vi "ex_allChanPropsMod.vi"(4 "error in (no error)":errorcluster, 5 "propertySource":string, 6 "DAQmx Channel":refnum<k21>, 7 "DAQmx Task":refnum<k21>) -> (0 "error out":errorcluster, 1 "TDM Property":T1, 2 "dup DAQmx Channel":refnum<k21>)   [LabVIEW 2020]
uses:
  <vilib>/express/express shared/ExFile.llb/ex_TdmProperty.ctl
  <vilib>/express/express shared/ex_EditUserDefinedProperties/usiDataType.ctl
  <vilib>/Platform/express/ex_EditUserDefinedProperties/ex_setTdmProperty_BLN.vi
  <vilib>/Platform/express/ex_EditUserDefinedProperties/ex_setTdmProperty_DBL.vi
  <vilib>/Platform/express/ex_EditUserDefinedProperties/ex_setTdmProperty_STR.vi
  <vilib>/Platform/express/ex_EditUserDefinedProperties/ex_setTdmProperty_I32.vi
  <vilib>/Platform/express/ex_EditUserDefinedProperties/ex_setTdmProperty_TME.vi
  <vilib>/Platform/express/ex_EditUserDefinedProperties/ex_setTdmProperty_1dDBL.vi
  <resource>/objmgr/daqmx.rc
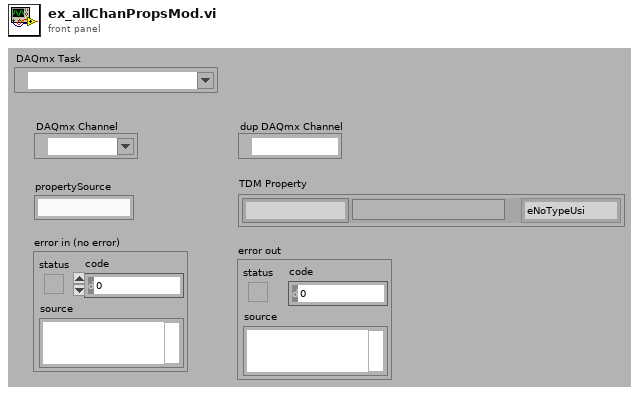
[diagram p1: front panel]
types:
  T1 = typedef "ex_TdmProperty.ctl" = cluster{"Name":string, "Type":T2, "Value":variant}
  T2 = typedef "usiDataType.ctl" = enum16{"eNoTypeUsi", "eInt8Usi", "eInt16Usi", "eInt32Usi", "eInt64Usi", "eUInt8Usi", "eUInt16Usi", "eUInt32Usi", "eUInt64Usi", "eFloat32Usi", "eFloat64Usi", "- 0", "- 1", "- 2", "- 3", "- 4", "- 5", "- 6", "- 7", "- 8", "- 9", "eString8Usi", "eString16Usi", "eStringUsi", "eEnumUsi", "- 10", "- 11", "- 12", "- 13", "- 14", "eTimeUsi", "- 15", "- 16", "- 17", "- 18", "- 19", "- 20", "- 21", "- 22", "- 23", "eInstanceUsi", "eStoreUsi"}
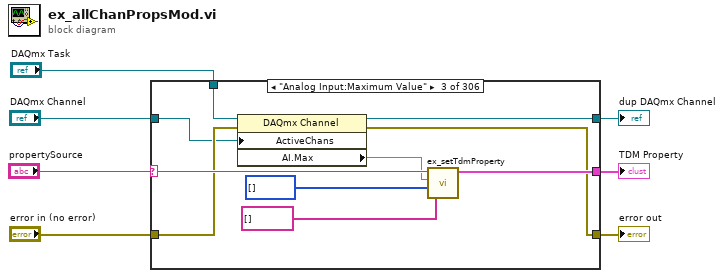
[diagram p0: block diagram]
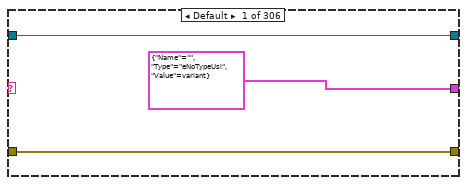
[diagram p2: hidden frame]
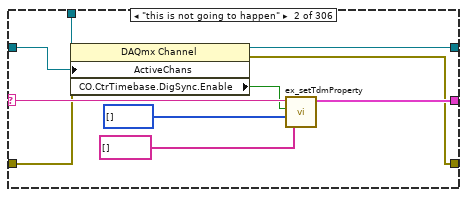
[diagram p3: hidden frame]
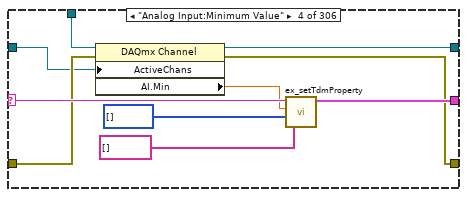
[diagram p4: hidden frame]
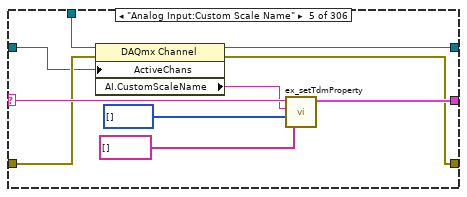
[diagram p5: hidden frame]
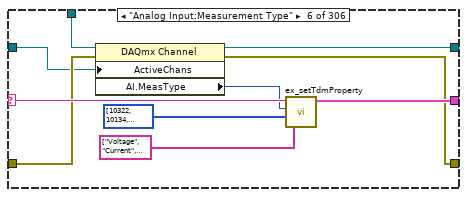
[diagram p6: hidden frame]
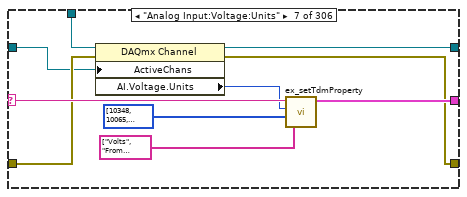
[diagram p7: hidden frame]
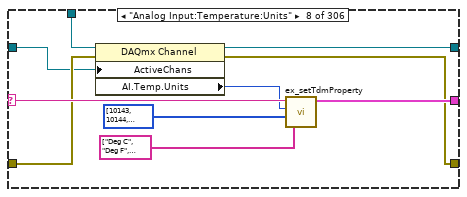
[diagram p8: hidden frame]
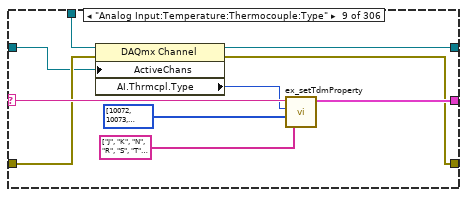
[diagram p9: hidden frame]
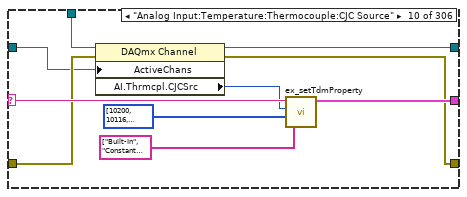
[diagram p10: hidden frame]
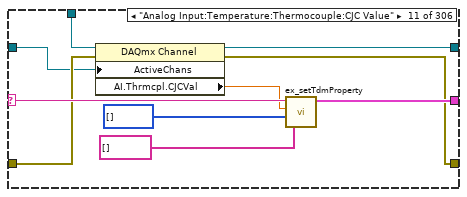
[diagram p11: hidden frame]
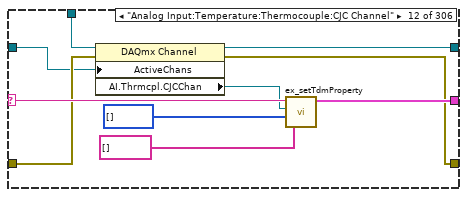
[diagram p12: hidden frame]
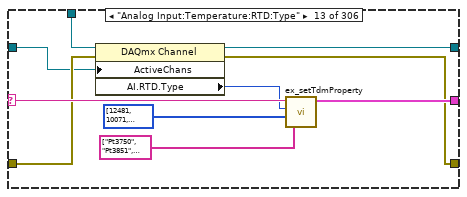
[diagram p13: hidden frame]
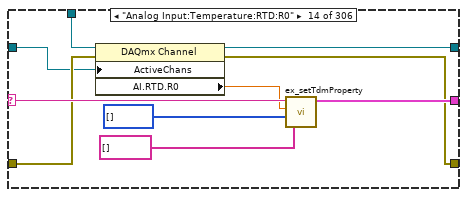
[diagram p14: hidden frame]
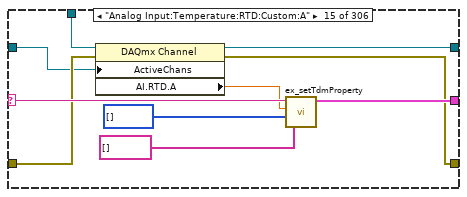
[diagram p15: hidden frame]
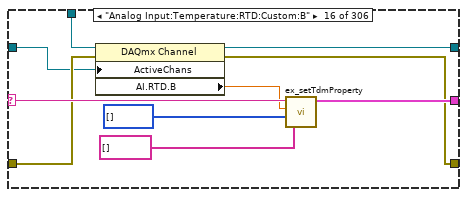
[diagram p16: hidden frame]
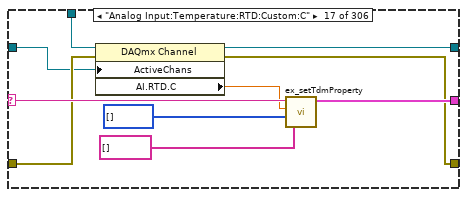
[diagram p17: hidden frame]
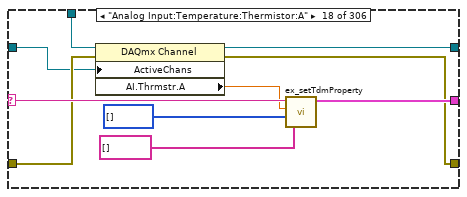
[diagram p18: hidden frame]
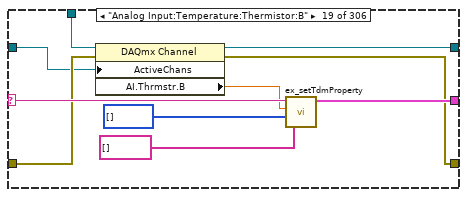
[diagram p19: hidden frame]
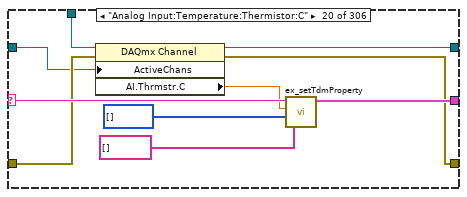
[diagram p20: hidden frame]
diagram:
  n1 = case shown="\"Analog Input:Maximum Value\"" "propertySource" {
    selector: "propertySource" -> [_ w19 w29 w39 w49 w59 w69 w79 w89 w99 w109 w119 w129 w139 w149 w159 w169 w179 w189 w199 w209 w219 w229 w239 w249 w259 w269 w279 w289 w299 w309 w319 w329 w339 w349 w359 w369 w379 w389 w399 w409 w419 w429 w439 w449 w459 w469 w479 w489 w499 w509 w519 w529 w539 w549 w559 w569 w579 w589 w599 w609 w619 w629 w639 w649 w659 w669 w679 w689 w699 w709 w719 w729 w739 w749 w759 w769 w779 w789 w799 w809 w819 w829 w839 w849 w859 w869 w879 w889 w899 w909 w919 w929 w939 w949 w959 w969 w979 w989 w999 w1009 w1019 w1029 w1039 w1049 w1059 w1069 w1079 w1089 w1099 w1109 w1119 w1129 w1139 w1149 w1159 w1169 w1179 w1189 w1199 w1209 w1219 w1229 w1239 w1249 w1259 w1269 w1279 w1289 w1299 w1309 w1319 w1329 w1339 w1349 w1359 w1369 w1379 w1389 w1399 w1409 w1419 w1429 w1439 w1449 w1459 w1469 w1479 w1489 w1499 w1509 w1519 w1529 w1539 w1549 w1559 w1569 w1579 w1589 w1599 w1609 w1619 w1629 w1639 w1649 w1659 w1669 w1679 w1689 w1699 w1709 w1719 w1729 w1739 w1749 w1759 w1769 w1779 w1789 w1799 w1809 w1819 w1829 w1839 w1849 w1859 w1869 w1879 w1889 w1899 w1909 w1919 w1929 w1939 w1949 w1959 w1969 w1979 w1989 w1999 w2009 w2019 w2029 w2039 w2049 w2059 w2069 w2079 w2089 w2099 w2109 w2119 w2129 w2139 w2149 w2159 w2169 w2179 w2189 w2199 w2209 w2219 w2229 w2239 w2249 w2259 w2269 w2279 w2289 w2299 w2309 w2319 w2329 w2339 w2349 w2359 w2369 w2379 w2389 w2399 w2409 w2419 w2429 w2439 w2449 w2459 w2469 w2479 w2489 w2499 w2509 w2519 w2529 w2539 w2549 w2559 w2569 w2579 w2589 w2599 w2609 w2619 w2629 w2639 w2649 w2659 w2669 w2679 w2689 w2699 w2709 w2719 w2729 w2739 w2749 w2759 w2769 w2779 w2789 w2799 w2809 w2819 w2829 w2839 w2849 w2859 w2869 w2879 w2889 w2899 w2909 w2919 w2929 w2939 w2949 w2959 w2969 w2979 w2989 w2999 w3009 w3019 w3029 w3039 w3049 w3059]
    tunnel: "error in (no error)" -> [w10 w17 w27 w37 w47 w57 w67 w77 w87 w97 w107 w117 w127 w137 w147 w157 w167 w177 w187 w197 w207 w217 w227 w237 w247 w257 w267 w277 w287 w297 w307 w317 w327 w337 w347 w357 w367 w377 w387 w397 w407 w417 w427 w437 w447 w457 w467 w477 w487 w497 w507 w517 w527 w537 w547 w557 w567 w577 w587 w597 w607 w617 w627 w637 w647 w657 w667 w677 w687 w697 w707 w717 w727 w737 w747 w757 w767 w777 w787 w797 w807 w817 w827 w837 w847 w857 w867 w877 w887 w897 w907 w917 w927 w937 w947 w957 w967 w977 w987 w997 w1007 w1017 w1027 w1037 w1047 w1057 w1067 w1077 w1087 w1097 w1107 w1117 w1127 w1137 w1147 w1157 w1167 w1177 w1187 w1197 w1207 w1217 w1227 w1237 w1247 w1257 w1267 w1277 w1287 w1297 w1307 w1317 w1327 w1337 w1347 w1357 w1367 w1377 w1387 w1397 w1407 w1417 w1427 w1437 w1447 w1457 w1467 w1477 w1487 w1497 w1507 w1517 w1527 w1537 w1547 w1557 w1567 w1577 w1587 w1597 w1607 w1617 w1627 w1637 w1647 w1657 w1667 w1677 w1687 w1697 w1707 w1717 w1727 w1737 w1747 w1757 w1767 w1777 w1787 w1797 w1807 w1817 w1827 w1837 w1847 w1857 w1867 w1877 w1887 w1897 w1907 w1917 w1927 w1937 w1947 w1957 w1967 w1977 w1987 w1997 w2007 w2017 w2027 w2037 w2047 w2057 w2067 w2077 w2087 w2097 w2107 w2117 w2127 w2137 w2147 w2157 w2167 w2177 w2187 w2197 w2207 w2217 w2227 w2237 w2247 w2257 w2267 w2277 w2287 w2297 w2307 w2317 w2327 w2337 w2347 w2357 w2367 w2377 w2387 w2397 w2407 w2417 w2427 w2437 w2447 w2457 w2467 w2477 w2487 w2497 w2507 w2517 w2527 w2537 w2547 w2557 w2567 w2577 w2587 w2597 w2607 w2617 w2627 w2637 w2647 w2657 w2667 w2677 w2687 w2697 w2707 w2717 w2727 w2737 w2747 w2757 w2767 w2777 w2787 w2797 w2807 w2817 w2827 w2837 w2847 w2857 w2867 w2877 w2887 w2897 w2907 w2917 w2927 w2937 w2947 w2957 w2967 w2977 w2987 w2997 w3007 w3017 w3027 w3037 w3047 w3057]
    tunnel: [w10 w16 w26 w36 w46 w56 w66 w76 w86 w96 w106 w116 w126 w136 w146 w156 w166 w176 w186 w196 w206 w216 w226 w236 w246 w256 w266 w276 w286 w296 w306 w316 w326 w336 w346 w356 w366 w376 w386 w396 w406 w416 w426 w436 w446 w456 w466 w476 w486 w496 w506 w516 w526 w536 w546 w556 w566 w576 w586 w596 w606 w616 w626 w636 w646 w656 w666 w676 w686 w696 w706 w716 w726 w736 w746 w756 w766 w776 w786 w796 w806 w816 w826 w836 w846 w856 w866 w876 w886 w896 w906 w916 w926 w936 w946 w956 w966 w976 w986 w996 w1006 w1016 w1026 w1036 w1046 w1056 w1066 w1076 w1086 w1096 w1106 w1116 w1126 w1136 w1146 w1156 w1166 w1176 w1186 w1196 w1206 w1216 w1226 w1236 w1246 w1256 w1266 w1276 w1286 w1296 w1306 w1316 w1326 w1336 w1346 w1356 w1366 w1376 w1386 w1396 w1406 w1416 w1426 w1436 w1446 w1456 w1466 w1476 w1486 w1496 w1506 w1516 w1526 w1536 w1546 w1556 w1566 w1576 w1586 w1596 w1606 w1616 w1626 w1636 w1646 w1656 w1666 w1676 w1686 w1696 w1706 w1716 w1726 w1736 w1746 w1756 w1766 w1776 w1786 w1796 w1806 w1816 w1826 w1836 w1846 w1856 w1866 w1876 w1886 w1896 w1906 w1916 w1926 w1936 w1946 w1956 w1966 w1976 w1986 w1996 w2006 w2016 w2026 w2036 w2046 w2056 w2066 w2076 w2086 w2096 w2106 w2116 w2126 w2136 w2146 w2156 w2166 w2176 w2186 w2196 w2206 w2216 w2226 w2236 w2246 w2256 w2266 w2276 w2286 w2296 w2306 w2316 w2326 w2336 w2346 w2356 w2366 w2376 w2386 w2396 w2406 w2416 w2426 w2436 w2446 w2456 w2466 w2476 w2486 w2496 w2506 w2516 w2526 w2536 w2546 w2556 w2566 w2576 w2586 w2596 w2606 w2616 w2626 w2636 w2646 w2656 w2666 w2676 w2686 w2696 w2706 w2716 w2726 w2736 w2746 w2756 w2766 w2776 w2786 w2796 w2806 w2816 w2826 w2836 w2846 w2856 w2866 w2876 w2886 w2896 w2906 w2916 w2926 w2936 w2946 w2956 w2966 w2976 w2986 w2996 w3006 w3016 w3026 w3036 w3046 w3056] -> w4
    tunnel: "DAQmx Channel" -> [w9 w12 w22 w32 w42 w52 w62 w72 w82 w92 w102 w112 w122 w132 w142 w152 w162 w172 w182 w192 w202 w212 w222 w232 w242 w252 w262 w272 w282 w292 w302 w312 w322 w332 w342 w352 w362 w372 w382 w392 w402 w412 w422 w432 w442 w452 w462 w472 w482 w492 w502 w512 w522 w532 w542 w552 w562 w572 w582 w592 w602 w612 w622 w632 w642 w652 w662 w672 w682 w692 w702 w712 w722 w732 w742 w752 w762 w772 w782 w792 w802 w812 w822 w832 w842 w852 w862 w872 w882 w892 w902 w912 w922 w932 w942 w952 w962 w972 w982 w992 w1002 w1012 w1022 w1032 w1042 w1052 w1062 w1072 w1082 w1092 w1102 w1112 w1122 w1132 w1142 w1152 w1162 w1172 w1182 w1192 w1202 w1212 w1222 w1232 w1242 w1252 w1262 w1272 w1282 w1292 w1302 w1312 w1322 w1332 w1342 w1352 w1362 w1372 w1382 w1392 w1402 w1412 w1422 w1432 w1442 w1452 w1462 w1472 w1482 w1492 w1502 w1512 w1522 w1532 w1542 w1552 w1562 w1572 w1582 w1592 w1602 w1612 w1622 w1632 w1642 w1652 w1662 w1672 w1682 w1692 w1702 w1712 w1722 w1732 w1742 w1752 w1762 w1772 w1782 w1792 w1802 w1812 w1822 w1832 w1842 w1852 w1862 w1872 w1882 w1892 w1902 w1912 w1922 w1932 w1942 w1952 w1962 w1972 w1982 w1992 w2002 w2012 w2022 w2032 w2042 w2052 w2062 w2072 w2082 w2092 w2102 w2112 w2122 w2132 w2142 w2152 w2162 w2172 w2182 w2192 w2202 w2212 w2222 w2232 w2242 w2252 w2262 w2272 w2282 w2292 w2302 w2312 w2322 w2332 w2342 w2352 w2362 w2372 w2382 w2392 w2402 w2412 w2422 w2432 w2442 w2452 w2462 w2472 w2482 w2492 w2502 w2512 w2522 w2532 w2542 w2552 w2562 w2572 w2582 w2592 w2602 w2612 w2622 w2632 w2642 w2652 w2662 w2672 w2682 w2692 w2702 w2712 w2722 w2732 w2742 w2752 w2762 w2772 w2782 w2792 w2802 w2812 w2822 w2832 w2842 w2852 w2862 w2872 w2882 w2892 w2902 w2912 w2922 w2932 w2942 w2952 w2962 w2972 w2982 w2992 w3002 w3012 w3022 w3032 w3042 w3052]
    tunnel: [w9 w20 w30 w40 w50 w60 w70 w80 w90 w100 w110 w120 w130 w140 w150 w160 w170 w180 w190 w200 w210 w220 w230 w240 w250 w260 w270 w280 w290 w300 w310 w320 w330 w340 w350 w360 w370 w380 w390 w400 w410 w420 w430 w440 w450 w460 w470 w480 w490 w500 w510 w520 w530 w540 w550 w560 w570 w580 w590 w600 w610 w620 w630 w640 w650 w660 w670 w680 w690 w700 w710 w720 w730 w740 w750 w760 w770 w780 w790 w800 w810 w820 w830 w840 w850 w860 w870 w880 w890 w900 w910 w920 w930 w940 w950 w960 w970 w980 w990 w1000 w1010 w1020 w1030 w1040 w1050 w1060 w1070 w1080 w1090 w1100 w1110 w1120 w1130 w1140 w1150 w1160 w1170 w1180 w1190 w1200 w1210 w1220 w1230 w1240 w1250 w1260 w1270 w1280 w1290 w1300 w1310 w1320 w1330 w1340 w1350 w1360 w1370 w1380 w1390 w1400 w1410 w1420 w1430 w1440 w1450 w1460 w1470 w1480 w1490 w1500 w1510 w1520 w1530 w1540 w1550 w1560 w1570 w1580 w1590 w1600 w1610 w1620 w1630 w1640 w1650 w1660 w1670 w1680 w1690 w1700 w1710 w1720 w1730 w1740 w1750 w1760 w1770 w1780 w1790 w1800 w1810 w1820 w1830 w1840 w1850 w1860 w1870 w1880 w1890 w1900 w1910 w1920 w1930 w1940 w1950 w1960 w1970 w1980 w1990 w2000 w2010 w2020 w2030 w2040 w2050 w2060 w2070 w2080 w2090 w2100 w2110 w2120 w2130 w2140 w2150 w2160 w2170 w2180 w2190 w2200 w2210 w2220 w2230 w2240 w2250 w2260 w2270 w2280 w2290 w2300 w2310 w2320 w2330 w2340 w2350 w2360 w2370 w2380 w2390 w2400 w2410 w2420 w2430 w2440 w2450 w2460 w2470 w2480 w2490 w2500 w2510 w2520 w2530 w2540 w2550 w2560 w2570 w2580 w2590 w2600 w2610 w2620 w2630 w2640 w2650 w2660 w2670 w2680 w2690 w2700 w2710 w2720 w2730 w2740 w2750 w2760 w2770 w2780 w2790 w2800 w2810 w2820 w2830 w2840 w2850 w2860 w2870 w2880 w2890 w2900 w2910 w2920 w2930 w2940 w2950 w2960 w2970 w2980 w2990 w3000 w3010 w3020 w3030 w3040 w3050 w3060] -> w6
    tunnel: [T1 {"Name"="", "Type"=enum."eNoTypeUsi", "Value"=variant} ("TDM Property") w18 w28 w38 w48 w58 w68 w78 w88 w98 w108 w118 w128 w138 w148 w158 w168 w178 w188 w198 w208 w218 w228 w238 w248 w258 w268 w278 w288 w298 w308 w318 w328 w338 w348 w358 w368 w378 w388 w398 w408 w418 w428 w438 w448 w458 w468 w478 w488 w498 w508 w518 w528 w538 w548 w558 w568 w578 w588 w598 w608 w618 w628 w638 w648 w658 w668 w678 w688 w698 w708 w718 w728 w738 w748 w758 w768 w778 w788 w798 w808 w818 w828 w838 w848 w858 w868 w878 w888 w898 w908 w918 w928 w938 w948 w958 w968 w978 w988 w998 w1008 w1018 w1028 w1038 w1048 w1058 w1068 w1078 w1088 w1098 w1108 w1118 w1128 w1138 w1148 w1158 w1168 w1178 w1188 w1198 w1208 w1218 w1228 w1238 w1248 w1258 w1268 w1278 w1288 w1298 w1308 w1318 w1328 w1338 w1348 w1358 w1368 w1378 w1388 w1398 w1408 w1418 w1428 w1438 w1448 w1458 w1468 w1478 w1488 w1498 w1508 w1518 w1528 w1538 w1548 w1558 w1568 w1578 w1588 w1598 w1608 w1618 w1628 w1638 w1648 w1658 w1668 w1678 w1688 w1698 w1708 w1718 w1728 w1738 w1748 w1758 w1768 w1778 w1788 w1798 w1808 w1818 w1828 w1838 w1848 w1858 w1868 w1878 w1888 w1898 w1908 w1918 w1928 w1938 w1948 w1958 w1968 w1978 w1988 w1998 w2008 w2018 w2028 w2038 w2048 w2058 w2068 w2078 w2088 w2098 w2108 w2118 w2128 w2138 w2148 w2158 w2168 w2178 w2188 w2198 w2208 w2218 w2228 w2238 w2248 w2258 w2268 w2278 w2288 w2298 w2308 w2318 w2328 w2338 w2348 w2358 w2368 w2378 w2388 w2398 w2408 w2418 w2428 w2438 w2448 w2458 w2468 w2478 w2488 w2498 w2508 w2518 w2528 w2538 w2548 w2558 w2568 w2578 w2588 w2598 w2608 w2618 w2628 w2638 w2648 w2658 w2668 w2678 w2688 w2698 w2708 w2718 w2728 w2738 w2748 w2758 w2768 w2778 w2788 w2798 w2808 w2818 w2828 w2838 w2848 w2858 w2868 w2878 w2888 w2898 w2908 w2918 w2928 w2938 w2948 w2958 w2968 w2978 w2988 w2998 w3008 w3018 w3028 w3038 w3048 w3058] -> w7
    tunnel: "DAQmx Task" -> [_ w11 w21 w31 w41 w51 w61 w71 w81 w91 w101 w111 w121 w131 w141 w151 w161 w171 w181 w191 w201 w211 w221 w231 w241 w251 w261 w271 w281 w291 w301 w311 w321 w331 w341 w351 w361 w371 w381 w391 w401 w411 w421 w431 w441 w451 w461 w471 w481 w491 w501 w511 w521 w531 w541 w551 w561 w571 w581 w591 w601 w611 w621 w631 w641 w651 w661 w671 w681 w691 w701 w711 w721 w731 w741 w751 w761 w771 w781 w791 w801 w811 w821 w831 w841 w851 w861 w871 w881 w891 w901 w911 w921 w931 w941 w951 w961 w971 w981 w991 w1001 w1011 w1021 w1031 w1041 w1051 w1061 w1071 w1081 w1091 w1101 w1111 w1121 w1131 w1141 w1151 w1161 w1171 w1181 w1191 w1201 w1211 w1221 w1231 w1241 w1251 w1261 w1271 w1281 w1291 w1301 w1311 w1321 w1331 w1341 w1351 w1361 w1371 w1381 w1391 w1401 w1411 w1421 w1431 w1441 w1451 w1461 w1471 w1481 w1491 w1501 w1511 w1521 w1531 w1541 w1551 w1561 w1571 w1581 w1591 w1601 w1611 w1621 w1631 w1641 w1651 w1661 w1671 w1681 w1691 w1701 w1711 w1721 w1731 w1741 w1751 w1761 w1771 w1781 w1791 w1801 w1811 w1821 w1831 w1841 w1851 w1861 w1871 w1881 w1891 w1901 w1911 w1921 w1931 w1941 w1951 w1961 w1971 w1981 w1991 w2001 w2011 w2021 w2031 w2041 w2051 w2061 w2071 w2081 w2091 w2101 w2111 w2121 w2131 w2141 w2151 w2161 w2171 w2181 w2191 w2201 w2211 w2221 w2231 w2241 w2251 w2261 w2271 w2281 w2291 w2301 w2311 w2321 w2331 w2341 w2351 w2361 w2371 w2381 w2391 w2401 w2411 w2421 w2431 w2441 w2451 w2461 w2471 w2481 w2491 w2501 w2511 w2521 w2531 w2541 w2551 w2561 w2571 w2581 w2591 w2601 w2611 w2621 w2631 w2641 w2651 w2661 w2671 w2681 w2691 w2701 w2711 w2721 w2731 w2741 w2751 w2761 w2771 w2781 w2791 w2801 w2811 w2821 w2831 w2841 w2851 w2861 w2871 w2881 w2891 w2901 w2911 w2921 w2931 w2941 w2951 w2961 w2971 w2981 w2991 w3001 w3011 w3021 w3031 w3041 w3051]
    frame Default {
    }
    frame "this is not going to happen" {
      n2 = property class="DAQmx Channel"(reference=w11, error in=w17, "ActiveChans"=w12) -> (reference out=w20:refnum<k21>, error out=w16:errorcluster, "CO.CtrTimebase.DigSync.Enable"=w13:bool)
      n3 = call-poly <vilib>:"ex_setTdmProperty.vi"("Strings"=string[] [], "Values"=i32[] [], "Value"=w13, "Name"=w19) -> ("output cluster"=w18:T1)  [unwired: 3 in]
    }
    frame "Analog Input:Maximum Value" {
      n4 = property class="DAQmx Channel"(reference=w21, error in=w27, "ActiveChans"=w22) -> (reference out=w30:refnum<k21>, error out=w26:errorcluster, "AI.Max"=w23:dbl)
      n5 = call-poly <vilib>:"ex_setTdmProperty.vi"("Strings"=string[] [], "Values"=i32[] [], "Value"=w23, "Name"=w29) -> ("output cluster"=w28:T1)  [unwired: 3 in]
    }
    frame "Analog Input:Minimum Value" {
      n6 = property class="DAQmx Channel"(reference=w31, error in=w37, "ActiveChans"=w32) -> (reference out=w40:refnum<k21>, error out=w36:errorcluster, "AI.Min"=w33:dbl)
      n7 = call-poly <vilib>:"ex_setTdmProperty.vi"("Strings"=string[] [], "Values"=i32[] [], "Value"=w33, "Name"=w39) -> ("output cluster"=w38:T1)  [unwired: 3 in]
    }
    frame "Analog Input:Custom Scale Name" {
      n8 = property class="DAQmx Channel"(reference=w41, error in=w47, "ActiveChans"=w42) -> (reference out=w50:refnum<k21>, error out=w46:errorcluster, "AI.CustomScaleName"=w43:tag)
      n9 = call-poly <vilib>:"ex_setTdmProperty.vi"("Strings"=string[] [], "Values"=i32[] [], "Value"=w43, "Name"=w49) -> ("output cluster"=w48:T1)  [unwired: 3 in]
    }
    frame "Analog Input:Measurement Type" {
      n10 = property class="DAQmx Channel"(reference=w51, error in=w57, "ActiveChans"=w52) -> (reference out=w60:refnum<k21>, error out=w56:errorcluster, "AI.MeasType"=w53:i32)
      n11 = call-poly <vilib>:"ex_setTdmProperty.vi"("Strings"=string[] ["Voltage", "Current", "More:Voltage:Custom with Excitation", "Frequency", "Resistance", "Temperature:Thermocouple", "Temperature:Thermistor", "Temperature:RTD", "Temperature:Built-in Sensor", "Strain Gage", "Position:LVDT", "Position:RVDT", "Accelerometer", "Sound Pressure:Microphone", "TEDS Sensor"], "Values"=i32[] [10322, 10134, 10323, 10181, 10278, 10303, 10302, 10301, 10311, 10300, 10352, 10353, 10356, 10354, 12531], "Value"=w53, "Name"=w59) -> ("output cluster"=w58:T1)  [unwired: 3 in]
    }
    frame "Analog Input:Voltage:Units" {
      n12 = property class="DAQmx Channel"(reference=w61, error in=w67, "ActiveChans"=w62) -> (reference out=w70:refnum<k21>, error out=w66:errorcluster, "AI.Voltage.Units"=w63:i32)
      n13 = call-poly <vilib>:"ex_setTdmProperty.vi"("Strings"=string[] ["Volts", "From Custom Scale", "From TEDS"], "Values"=i32[] [10348, 10065, 12516], "Value"=w63, "Name"=w69) -> ("output cluster"=w68:T1)  [unwired: 3 in]
    }
    frame "Analog Input:Temperature:Units" {
      n14 = property class="DAQmx Channel"(reference=w71, error in=w77, "ActiveChans"=w72) -> (reference out=w80:refnum<k21>, error out=w76:errorcluster, "AI.Temp.Units"=w73:i32)
      n15 = call-poly <vilib>:"ex_setTdmProperty.vi"("Strings"=string[] ["Deg C", "Deg F", "Kelvins", "Deg R", "From Custom Scale"], "Values"=i32[] [10143, 10144, 10325, 10145, 10065], "Value"=w73, "Name"=w79) -> ("output cluster"=w78:T1)  [unwired: 3 in]
    }
    frame "Analog Input:Temperature:Thermocouple:Type" {
      n16 = property class="DAQmx Channel"(reference=w81, error in=w87, "ActiveChans"=w82) -> (reference out=w90:refnum<k21>, error out=w86:errorcluster, "AI.Thrmcpl.Type"=w83:i32)
      n17 = call-poly <vilib>:"ex_setTdmProperty.vi"("Strings"=string[] ["J", "K", "N", "R", "S", "T", "B", "E"], "Values"=i32[] [10072, 10073, 10077, 10082, 10085, 10086, 10047, 10055], "Value"=w83, "Name"=w89) -> ("output cluster"=w88:T1)  [unwired: 3 in]
    }
    frame "Analog Input:Temperature:Thermocouple:CJC Source" {
      n18 = property class="DAQmx Channel"(reference=w91, error in=w97, "ActiveChans"=w92) -> (reference out=w100:refnum<k21>, error out=w96:errorcluster, "AI.Thrmcpl.CJCSrc"=w93:i32)
      n19 = call-poly <vilib>:"ex_setTdmProperty.vi"("Strings"=string[] ["Built-In", "Constant Value", "Channel"], "Values"=i32[] [10200, 10116, 10113], "Value"=w93, "Name"=w99) -> ("output cluster"=w98:T1)  [unwired: 3 in]
    }
    frame "Analog Input:Temperature:Thermocouple:CJC Value" {
      n20 = property class="DAQmx Channel"(reference=w101, error in=w107, "ActiveChans"=w102) -> (reference out=w110:refnum<k21>, error out=w106:errorcluster, "AI.Thrmcpl.CJCVal"=w103:dbl)
      n21 = call-poly <vilib>:"ex_setTdmProperty.vi"("Strings"=string[] [], "Values"=i32[] [], "Value"=w103, "Name"=w109) -> ("output cluster"=w108:T1)  [unwired: 3 in]
    }
    frame "Analog Input:Temperature:Thermocouple:CJC Channel" {
      n22 = property class="DAQmx Channel"(reference=w111, error in=w117, "ActiveChans"=w112) -> (reference out=w120:refnum<k21>, error out=w116:errorcluster, "AI.Thrmcpl.CJCChan"=w113:refnum<k21>)
      n23 = call-poly <vilib>:"ex_setTdmProperty.vi"("Strings"=string[] [], "Values"=i32[] [], "Value"=w113, "Name"=w119) -> ("output cluster"=w118:T1)  [unwired: 3 in]
    }
    frame "Analog Input:Temperature:RTD:Type" {
      n24 = property class="DAQmx Channel"(reference=w121, error in=w127, "ActiveChans"=w122) -> (reference out=w130:refnum<k21>, error out=w126:errorcluster, "AI.RTD.Type"=w123:i32)
      n25 = call-poly <vilib>:"ex_setTdmProperty.vi"("Strings"=string[] ["Pt3750", "Pt3851", "Pt3911", "Pt3916", "Pt3920", "Pt3928", "Custom"], "Values"=i32[] [12481, 10071, 12482, 10069, 10053, 12483, 10137], "Value"=w123, "Name"=w129) -> ("output cluster"=w128:T1)  [unwired: 3 in]
    }
    frame "Analog Input:Temperature:RTD:R0" {
      n26 = property class="DAQmx Channel"(reference=w131, error in=w137, "ActiveChans"=w132) -> (reference out=w140:refnum<k21>, error out=w136:errorcluster, "AI.RTD.R0"=w133:dbl)
      n27 = call-poly <vilib>:"ex_setTdmProperty.vi"("Strings"=string[] [], "Values"=i32[] [], "Value"=w133, "Name"=w139) -> ("output cluster"=w138:T1)  [unwired: 3 in]
    }
    frame "Analog Input:Temperature:RTD:Custom:A" {
      n28 = property class="DAQmx Channel"(reference=w141, error in=w147, "ActiveChans"=w142) -> (reference out=w150:refnum<k21>, error out=w146:errorcluster, "AI.RTD.A"=w143:dbl)
      n29 = call-poly <vilib>:"ex_setTdmProperty.vi"("Strings"=string[] [], "Values"=i32[] [], "Value"=w143, "Name"=w149) -> ("output cluster"=w148:T1)  [unwired: 3 in]
    }
    frame "Analog Input:Temperature:RTD:Custom:B" {
      n30 = property class="DAQmx Channel"(reference=w151, error in=w157, "ActiveChans"=w152) -> (reference out=w160:refnum<k21>, error out=w156:errorcluster, "AI.RTD.B"=w153:dbl)
      n31 = call-poly <vilib>:"ex_setTdmProperty.vi"("Strings"=string[] [], "Values"=i32[] [], "Value"=w153, "Name"=w159) -> ("output cluster"=w158:T1)  [unwired: 3 in]
    }
    frame "Analog Input:Temperature:RTD:Custom:C" {
      n32 = property class="DAQmx Channel"(reference=w161, error in=w167, "ActiveChans"=w162) -> (reference out=w170:refnum<k21>, error out=w166:errorcluster, "AI.RTD.C"=w163:dbl)
      n33 = call-poly <vilib>:"ex_setTdmProperty.vi"("Strings"=string[] [], "Values"=i32[] [], "Value"=w163, "Name"=w169) -> ("output cluster"=w168:T1)  [unwired: 3 in]
    }
    frame "Analog Input:Temperature:Thermistor:A" {
      n34 = property class="DAQmx Channel"(reference=w171, error in=w177, "ActiveChans"=w172) -> (reference out=w180:refnum<k21>, error out=w176:errorcluster, "AI.Thrmstr.A"=w173:dbl)
      n35 = call-poly <vilib>:"ex_setTdmProperty.vi"("Strings"=string[] [], "Values"=i32[] [], "Value"=w173, "Name"=w179) -> ("output cluster"=w178:T1)  [unwired: 3 in]
    }
    frame "Analog Input:Temperature:Thermistor:B" {
      n36 = property class="DAQmx Channel"(reference=w181, error in=w187, "ActiveChans"=w182) -> (reference out=w190:refnum<k21>, error out=w186:errorcluster, "AI.Thrmstr.B"=w183:dbl)
      n37 = call-poly <vilib>:"ex_setTdmProperty.vi"("Strings"=string[] [], "Values"=i32[] [], "Value"=w183, "Name"=w189) -> ("output cluster"=w188:T1)  [unwired: 3 in]
    }
    frame "Analog Input:Temperature:Thermistor:C" {
      n38 = property class="DAQmx Channel"(reference=w191, error in=w197, "ActiveChans"=w192) -> (reference out=w200:refnum<k21>, error out=w196:errorcluster, "AI.Thrmstr.C"=w193:dbl)
      n39 = call-poly <vilib>:"ex_setTdmProperty.vi"("Strings"=string[] [], "Values"=i32[] [], "Value"=w193, "Name"=w199) -> ("output cluster"=w198:T1)  [unwired: 3 in]
    }
    frame "Analog Input:Temperature:Thermistor:R1" {
      n40 = property class="DAQmx Channel"(reference=w201, error in=w207, "ActiveChans"=w202) -> (reference out=w210:refnum<k21>, error out=w206:errorcluster, "AI.Thrmstr.R1"=w203:dbl)
      n41 = call-poly <vilib>:"ex_setTdmProperty.vi"("Strings"=string[] [], "Values"=i32[] [], "Value"=w203, "Name"=w209) -> ("output cluster"=w208:T1)  [unwired: 3 in]
    }
    frame "Analog Input:Temperature:Advanced:Force Read from Channel" {
      n42 = property class="DAQmx Channel"(reference=w211, error in=w217, "ActiveChans"=w212) -> (reference out=w220:refnum<k21>, error out=w216:errorcluster, "AI.ForceReadFromChan"=w213:bool)
      n43 = call-poly <vilib>:"ex_setTdmProperty.vi"("Strings"=string[] [], "Values"=i32[] [], "Value"=w213, "Name"=w219) -> ("output cluster"=w218:T1)  [unwired: 3 in]
    }
    frame "Analog Input:Current:Units" {
      n44 = property class="DAQmx Channel"(reference=w221, error in=w227, "ActiveChans"=w222) -> (reference out=w230:refnum<k21>, error out=w226:errorcluster, "AI.Current.Units"=w223:i32)
      n45 = call-poly <vilib>:"ex_setTdmProperty.vi"("Strings"=string[] ["Amps", "From Custom Scale", "From TEDS"], "Values"=i32[] [10342, 10065, 12516], "Value"=w223, "Name"=w229) -> ("output cluster"=w228:T1)  [unwired: 3 in]
    }
    frame "Analog Input:Strain:Units" {
      n46 = property class="DAQmx Channel"(reference=w231, error in=w237, "ActiveChans"=w232) -> (reference out=w240:refnum<k21>, error out=w236:errorcluster, "AI.Strain.Units"=w233:i32)
      n47 = call-poly <vilib>:"ex_setTdmProperty.vi"("Strings"=string[] ["Strain", "From Custom Scale"], "Values"=i32[] [10299, 10065], "Value"=w233, "Name"=w239) -> ("output cluster"=w238:T1)  [unwired: 3 in]
    }
    frame "Analog Input:Strain:Strain Gage:Gage Factor" {
      n48 = property class="DAQmx Channel"(reference=w241, error in=w247, "ActiveChans"=w242) -> (reference out=w250:refnum<k21>, error out=w246:errorcluster, "AI.StrainGage.GageFactor"=w243:dbl)
      n49 = call-poly <vilib>:"ex_setTdmProperty.vi"("Strings"=string[] [], "Values"=i32[] [], "Value"=w243, "Name"=w249) -> ("output cluster"=w248:T1)  [unwired: 3 in]
    }
    frame "Analog Input:Strain:Strain Gage:Poisson Ratio" {
      n50 = property class="DAQmx Channel"(reference=w251, error in=w257, "ActiveChans"=w252) -> (reference out=w260:refnum<k21>, error out=w256:errorcluster, "AI.StrainGage.PoissonRatio"=w253:dbl)
      n51 = call-poly <vilib>:"ex_setTdmProperty.vi"("Strings"=string[] [], "Values"=i32[] [], "Value"=w253, "Name"=w259) -> ("output cluster"=w258:T1)  [unwired: 3 in]
    }
    frame "Analog Input:Strain:Strain Gage:Configuration" {
      n52 = property class="DAQmx Channel"(reference=w261, error in=w267, "ActiveChans"=w262) -> (reference out=w270:refnum<k21>, error out=w266:errorcluster, "AI.StrainGage.Cfg"=w263:i32)
      n53 = call-poly <vilib>:"ex_setTdmProperty.vi"("Strings"=string[] ["Full Bridge I", "Full Bridge II", "Full Bridge III", "Half Bridge I", "Half Bridge II", "Quarter Bridge I", "Quarter Bridge II"], "Values"=i32[] [10183, 10184, 10185, 10188, 10189, 10271, 10272], "Value"=w263, "Name"=w269) -> ("output cluster"=w268:T1)  [unwired: 3 in]
    }
    frame "Analog Input:Resistance:Units" {
      n54 = property class="DAQmx Channel"(reference=w271, error in=w277, "ActiveChans"=w272) -> (reference out=w280:refnum<k21>, error out=w276:errorcluster, "AI.Resistance.Units"=w273:i32)
      n55 = call-poly <vilib>:"ex_setTdmProperty.vi"("Strings"=string[] ["Ohms", "From Custom Scale", "From TEDS"], "Values"=i32[] [10384, 10065, 12516], "Value"=w273, "Name"=w279) -> ("output cluster"=w278:T1)  [unwired: 3 in]
    }
    frame "Analog Input:Frequency:Units" {
      n56 = property class="DAQmx Channel"(reference=w281, error in=w287, "ActiveChans"=w282) -> (reference out=w290:refnum<k21>, error out=w286:errorcluster, "AI.Freq.Units"=w283:i32)
      n57 = call-poly <vilib>:"ex_setTdmProperty.vi"("Strings"=string[] ["Hz", "From Custom Scale"], "Values"=i32[] [10373, 10065], "Value"=w283, "Name"=w289) -> ("output cluster"=w288:T1)  [unwired: 3 in]
    }
    frame "Analog Input:Frequency:Voltage:Threshold Level" {
      n58 = property class="DAQmx Channel"(reference=w291, error in=w297, "ActiveChans"=w292) -> (reference out=w300:refnum<k21>, error out=w296:errorcluster, "AI.Freq.ThreshVoltage"=w293:dbl)
      n59 = call-poly <vilib>:"ex_setTdmProperty.vi"("Strings"=string[] [], "Values"=i32[] [], "Value"=w293, "Name"=w299) -> ("output cluster"=w298:T1)  [unwired: 3 in]
    }
    frame "Analog Input:Frequency:Voltage:Hysteresis" {
      n60 = property class="DAQmx Channel"(reference=w301, error in=w307, "ActiveChans"=w302) -> (reference out=w310:refnum<k21>, error out=w306:errorcluster, "AI.Freq.Hyst"=w303:dbl)
      n61 = call-poly <vilib>:"ex_setTdmProperty.vi"("Strings"=string[] [], "Values"=i32[] [], "Value"=w303, "Name"=w309) -> ("output cluster"=w308:T1)  [unwired: 3 in]
    }
    frame "Analog Input:Position:LVDT:Units" {
      n62 = property class="DAQmx Channel"(reference=w311, error in=w317, "ActiveChans"=w312) -> (reference out=w320:refnum<k21>, error out=w316:errorcluster, "AI.LVDT.Units"=w313:i32)
      n63 = call-poly <vilib>:"ex_setTdmProperty.vi"("Strings"=string[] ["Meters", "Inches", "From Custom Scale"], "Values"=i32[] [10219, 10379, 10065], "Value"=w313, "Name"=w319) -> ("output cluster"=w318:T1)  [unwired: 3 in]
    }
    frame "Analog Input:Position:LVDT:Sensitivity" {
      n64 = property class="DAQmx Channel"(reference=w321, error in=w327, "ActiveChans"=w322) -> (reference out=w330:refnum<k21>, error out=w326:errorcluster, "AI.LVDT.Sensitivity"=w323:dbl)
      n65 = call-poly <vilib>:"ex_setTdmProperty.vi"("Strings"=string[] [], "Values"=i32[] [], "Value"=w323, "Name"=w329) -> ("output cluster"=w328:T1)  [unwired: 3 in]
    }
    frame "Analog Input:Position:LVDT:Sensitivity Units" {
      n66 = property class="DAQmx Channel"(reference=w331, error in=w337, "ActiveChans"=w332) -> (reference out=w340:refnum<k21>, error out=w336:errorcluster, "AI.LVDT.SensitivityUnits"=w333:i32)
      n67 = call-poly <vilib>:"ex_setTdmProperty.vi"("Strings"=string[] ["mVolts/Volt/mMeter", "mVolts/Volt/0.001 Inch"], "Values"=i32[] [12506, 12505], "Value"=w333, "Name"=w339) -> ("output cluster"=w338:T1)  [unwired: 3 in]
    }
    frame "Analog Input:Position:RVDT:Units" {
      n68 = property class="DAQmx Channel"(reference=w341, error in=w347, "ActiveChans"=w342) -> (reference out=w350:refnum<k21>, error out=w346:errorcluster, "AI.RVDT.Units"=w343:i32)
      n69 = call-poly <vilib>:"ex_setTdmProperty.vi"("Strings"=string[] ["Degrees", "Radians", "From Custom Scale"], "Values"=i32[] [10146, 10273, 10065], "Value"=w343, "Name"=w349) -> ("output cluster"=w348:T1)  [unwired: 3 in]
    }
    frame "Analog Input:Position:RVDT:Sensitivity" {
      n70 = property class="DAQmx Channel"(reference=w351, error in=w357, "ActiveChans"=w352) -> (reference out=w360:refnum<k21>, error out=w356:errorcluster, "AI.RVDT.Sensitivity"=w353:dbl)
      n71 = call-poly <vilib>:"ex_setTdmProperty.vi"("Strings"=string[] [], "Values"=i32[] [], "Value"=w353, "Name"=w359) -> ("output cluster"=w358:T1)  [unwired: 3 in]
    }
    frame "Analog Input:Position:RVDT:Sensitivity Units" {
      n72 = property class="DAQmx Channel"(reference=w361, error in=w367, "ActiveChans"=w362) -> (reference out=w370:refnum<k21>, error out=w366:errorcluster, "AI.RVDT.SensitivityUnits"=w363:i32)
      n73 = call-poly <vilib>:"ex_setTdmProperty.vi"("Strings"=string[] ["mVolts/Volt/Degree", "mVolts/Volt/Radian"], "Values"=i32[] [12507, 12508], "Value"=w363, "Name"=w369) -> ("output cluster"=w368:T1)  [unwired: 3 in]
    }
    frame "Analog Input:Sound Pressure:Maximum Sound Pressure Level" {
      n74 = property class="DAQmx Channel"(reference=w371, error in=w377, "ActiveChans"=w372) -> (reference out=w380:refnum<k21>, error out=w376:errorcluster, "AI.SoundPressure.MaxSoundPressureLvl"=w373:dbl)
      n75 = call-poly <vilib>:"ex_setTdmProperty.vi"("Strings"=string[] [], "Values"=i32[] [], "Value"=w373, "Name"=w379) -> ("output cluster"=w378:T1)  [unwired: 3 in]
    }
    frame "Analog Input:Sound Pressure:Units" {
      n76 = property class="DAQmx Channel"(reference=w381, error in=w387, "ActiveChans"=w382) -> (reference out=w390:refnum<k21>, error out=w386:errorcluster, "AI.SoundPressure.Units"=w383:i32)
      n77 = call-poly <vilib>:"ex_setTdmProperty.vi"("Strings"=string[] ["Pascals", "From Custom Scale"], "Values"=i32[] [10081, 10065], "Value"=w383, "Name"=w389) -> ("output cluster"=w388:T1)  [unwired: 3 in]
    }
    frame "Analog Input:Sound Pressure:Microphone:Sensitivity" {
      n78 = property class="DAQmx Channel"(reference=w391, error in=w397, "ActiveChans"=w392) -> (reference out=w400:refnum<k21>, error out=w396:errorcluster, "AI.Microphone.Sensitivity"=w393:dbl)
      n79 = call-poly <vilib>:"ex_setTdmProperty.vi"("Strings"=string[] [], "Values"=i32[] [], "Value"=w393, "Name"=w399) -> ("output cluster"=w398:T1)  [unwired: 3 in]
    }
    frame "Analog Input:Acceleration:Units" {
      n80 = property class="DAQmx Channel"(reference=w401, error in=w407, "ActiveChans"=w402) -> (reference out=w410:refnum<k21>, error out=w406:errorcluster, "AI.Accel.Units"=w403:i32)
      n81 = call-poly <vilib>:"ex_setTdmProperty.vi"("Strings"=string[] ["g", "m/s^2", "From Custom Scale"], "Values"=i32[] [10186, 12470, 10065], "Value"=w403, "Name"=w409) -> ("output cluster"=w408:T1)  [unwired: 3 in]
    }
    frame "Analog Input:Acceleration:Accelerometer:Sensitivity" {
      n82 = property class="DAQmx Channel"(reference=w411, error in=w417, "ActiveChans"=w412) -> (reference out=w420:refnum<k21>, error out=w416:errorcluster, "AI.Accel.Sensitivity"=w413:dbl)
      n83 = call-poly <vilib>:"ex_setTdmProperty.vi"("Strings"=string[] [], "Values"=i32[] [], "Value"=w413, "Name"=w419) -> ("output cluster"=w418:T1)  [unwired: 3 in]
    }
    frame "Analog Input:Acceleration:Accelerometer:Sensitivity Units" {
      n84 = property class="DAQmx Channel"(reference=w421, error in=w427, "ActiveChans"=w422) -> (reference out=w430:refnum<k21>, error out=w426:errorcluster, "AI.Accel.SensitivityUnits"=w423:i32)
      n85 = call-poly <vilib>:"ex_setTdmProperty.vi"("Strings"=string[] ["mVolts/g", "Volts/g"], "Values"=i32[] [12509, 12510], "Value"=w423, "Name"=w429) -> ("output cluster"=w428:T1)  [unwired: 3 in]
    }
    frame "Analog Input:TEDS:Units" {
      n86 = property class="DAQmx Channel"(reference=w431, error in=w437, "ActiveChans"=w432) -> (reference out=w440:refnum<k21>, error out=w436:errorcluster, "AI.TEDS.Units"=w433:string)
      n87 = call-poly <vilib>:"ex_setTdmProperty.vi"("Strings"=string[] [], "Values"=i32[] [], "Value"=w433, "Name"=w439) -> ("output cluster"=w438:T1)  [unwired: 3 in]
    }
    frame "Analog Input:General Properties:Input Configuration:Coupling" {
      n88 = property class="DAQmx Channel"(reference=w441, error in=w447, "ActiveChans"=w442) -> (reference out=w450:refnum<k21>, error out=w446:errorcluster, "AI.Coupling"=w443:i32)
      n89 = call-poly <vilib>:"ex_setTdmProperty.vi"("Strings"=string[] ["AC", "DC", "GND"], "Values"=i32[] [10045, 10050, 10066], "Value"=w443, "Name"=w449) -> ("output cluster"=w448:T1)  [unwired: 3 in]
    }
    frame "Analog Input:General Properties:Input Configuration:Impedance" {
      n90 = property class="DAQmx Channel"(reference=w451, error in=w457, "ActiveChans"=w452) -> (reference out=w460:refnum<k21>, error out=w456:errorcluster, "AI.Impedance"=w453:dbl)
      n91 = call-poly <vilib>:"ex_setTdmProperty.vi"("Strings"=string[] ["50 Ohms", "75 Ohms", "1 M Ohm", "10 G Ohms"], "Values"=i32[] [50, 75, 1000000, 2147483647], "Value"=w453, "Name"=w459) -> ("output cluster"=w458:T1)  [unwired: 3 in]
    }
    frame "Analog Input:General Properties:Input Configuration:Terminal Configuration" {
      n92 = property class="DAQmx Channel"(reference=w461, error in=w467, "ActiveChans"=w462) -> (reference out=w470:refnum<k21>, error out=w466:errorcluster, "AI.TermCfg"=w463:i32)
      n93 = call-poly <vilib>:"ex_setTdmProperty.vi"("Strings"=string[] ["RSE", "NRSE", "Differential", "Pseudodifferential"], "Values"=i32[] [10083, 10078, 10106, 12529], "Value"=w463, "Name"=w469) -> ("output cluster"=w468:T1)  [unwired: 3 in]
    }
    frame "Analog Input:General Properties:Input Configuration:Input Source" {
      n94 = property class="DAQmx Channel"(reference=w471, error in=w477, "ActiveChans"=w472) -> (reference out=w480:refnum<k21>, error out=w476:errorcluster, "AI.InputSrc"=w473:string)
      n95 = call-poly <vilib>:"ex_setTdmProperty.vi"("Strings"=string[] [], "Values"=i32[] [], "Value"=w473, "Name"=w479) -> ("output cluster"=w478:T1)  [unwired: 3 in]
    }
    frame "Analog Input:General Properties:Signal Conditioning:Resistance Configuration" {
      n96 = property class="DAQmx Channel"(reference=w481, error in=w487, "ActiveChans"=w482) -> (reference out=w490:refnum<k21>, error out=w486:errorcluster, "AI.ResistanceCfg"=w483:i32)
      n97 = call-poly <vilib>:"ex_setTdmProperty.vi"("Strings"=string[] ["2-Wire", "3-Wire", "4-Wire"], "Values"=i32[] [2, 3, 4], "Value"=w483, "Name"=w489) -> ("output cluster"=w488:T1)  [unwired: 3 in]
    }
    frame "Analog Input:General Properties:Signal Conditioning:Lead Wire Resistance" {
      n98 = property class="DAQmx Channel"(reference=w491, error in=w497, "ActiveChans"=w492) -> (reference out=w500:refnum<k21>, error out=w496:errorcluster, "AI.LeadWireResistance"=w493:dbl)
      n99 = call-poly <vilib>:"ex_setTdmProperty.vi"("Strings"=string[] [], "Values"=i32[] [], "Value"=w493, "Name"=w499) -> ("output cluster"=w498:T1)  [unwired: 3 in]
    }
    frame "Analog Input:General Properties:Signal Conditioning:Bridge:Configuration" {
      n100 = property class="DAQmx Channel"(reference=w501, error in=w507, "ActiveChans"=w502) -> (reference out=w510:refnum<k21>, error out=w506:errorcluster, "AI.Bridge.Cfg"=w503:i32)
      n101 = call-poly <vilib>:"ex_setTdmProperty.vi"("Strings"=string[] ["Full Bridge", "Half Bridge", "Quarter Bridge", "No Bridge"], "Values"=i32[] [10182, 10187, 10270, 10228], "Value"=w503, "Name"=w509) -> ("output cluster"=w508:T1)  [unwired: 3 in]
    }
    frame "Analog Input:General Properties:Signal Conditioning:Bridge:Nominal Resistance" {
      n102 = property class="DAQmx Channel"(reference=w511, error in=w517, "ActiveChans"=w512) -> (reference out=w520:refnum<k21>, error out=w516:errorcluster, "AI.Bridge.NomResistance"=w513:dbl)
      n103 = call-poly <vilib>:"ex_setTdmProperty.vi"("Strings"=string[] [], "Values"=i32[] [], "Value"=w513, "Name"=w519) -> ("output cluster"=w518:T1)  [unwired: 3 in]
    }
    frame "Analog Input:General Properties:Signal Conditioning:Bridge:Initial Bridge Voltage" {
      n104 = property class="DAQmx Channel"(reference=w521, error in=w527, "ActiveChans"=w522) -> (reference out=w530:refnum<k21>, error out=w526:errorcluster, "AI.Bridge.InitialVoltage"=w523:dbl)
      n105 = call-poly <vilib>:"ex_setTdmProperty.vi"("Strings"=string[] [], "Values"=i32[] [], "Value"=w523, "Name"=w529) -> ("output cluster"=w528:T1)  [unwired: 3 in]
    }
    frame "Analog Input:General Properties:Signal Conditioning:Bridge:Shunt Cal:Shunt Cal Enable" {
      n106 = property class="DAQmx Channel"(reference=w531, error in=w537, "ActiveChans"=w532) -> (reference out=w540:refnum<k21>, error out=w536:errorcluster, "AI.Bridge.ShuntCal.Enable"=w533:bool)
      n107 = call-poly <vilib>:"ex_setTdmProperty.vi"("Strings"=string[] [], "Values"=i32[] [], "Value"=w533, "Name"=w539) -> ("output cluster"=w538:T1)  [unwired: 3 in]
    }
    frame "Analog Input:General Properties:Signal Conditioning:Bridge:Shunt Cal:Shunt Cal Select" {
      n108 = property class="DAQmx Channel"(reference=w541, error in=w547, "ActiveChans"=w542) -> (reference out=w550:refnum<k21>, error out=w546:errorcluster, "AI.Bridge.ShuntCal.Select"=w543:i32)
      n109 = call-poly <vilib>:"ex_setTdmProperty.vi"("Strings"=string[] ["A", "B", "A and B"], "Values"=i32[] [12513, 12514, 12515], "Value"=w543, "Name"=w549) -> ("output cluster"=w548:T1)  [unwired: 3 in]
    }
    frame "Analog Input:General Properties:Signal Conditioning:Bridge:Shunt Cal:Gain Adjustment" {
      n110 = property class="DAQmx Channel"(reference=w551, error in=w557, "ActiveChans"=w552) -> (reference out=w560:refnum<k21>, error out=w556:errorcluster, "AI.Bridge.ShuntCal.GainAdjust"=w553:dbl)
      n111 = call-poly <vilib>:"ex_setTdmProperty.vi"("Strings"=string[] [], "Values"=i32[] [], "Value"=w553, "Name"=w559) -> ("output cluster"=w558:T1)  [unwired: 3 in]
    }
    frame "Analog Input:General Properties:Signal Conditioning:Bridge:Balance:Coarse Potentiometer" {
      n112 = property class="DAQmx Channel"(reference=w561, error in=w567, "ActiveChans"=w562) -> (reference out=w570:refnum<k21>, error out=w566:errorcluster, "AI.Bridge.Balance.CoarsePot"=w563:i32)
      n113 = call-poly <vilib>:"ex_setTdmProperty.vi"("Strings"=string[] [], "Values"=i32[] [], "Value"=w563, "Name"=w569) -> ("output cluster"=w568:T1)  [unwired: 3 in]
    }
    frame "Analog Input:General Properties:Signal Conditioning:Bridge:Balance:Fine Potentiometer" {
      n114 = property class="DAQmx Channel"(reference=w571, error in=w577, "ActiveChans"=w572) -> (reference out=w580:refnum<k21>, error out=w576:errorcluster, "AI.Bridge.Balance.FinePot"=w573:i32)
      n115 = call-poly <vilib>:"ex_setTdmProperty.vi"("Strings"=string[] [], "Values"=i32[] [], "Value"=w573, "Name"=w579) -> ("output cluster"=w578:T1)  [unwired: 3 in]
    }
    frame "Analog Input:General Properties:Signal Conditioning:Current Shunt Resistor:Location" {
      n116 = property class="DAQmx Channel"(reference=w581, error in=w587, "ActiveChans"=w582) -> (reference out=w590:refnum<k21>, error out=w586:errorcluster, "AI.CurrentShunt.Loc"=w583:i32)
      n117 = call-poly <vilib>:"ex_setTdmProperty.vi"("Strings"=string[] ["Internal", "External"], "Values"=i32[] [10200, 10167], "Value"=w583, "Name"=w589) -> ("output cluster"=w588:T1)  [unwired: 3 in]
    }
    frame "Analog Input:General Properties:Signal Conditioning:Current Shunt Resistor:Value" {
      n118 = property class="DAQmx Channel"(reference=w591, error in=w597, "ActiveChans"=w592) -> (reference out=w600:refnum<k21>, error out=w596:errorcluster, "AI.CurrentShunt.Resistance"=w593:dbl)
      n119 = call-poly <vilib>:"ex_setTdmProperty.vi"("Strings"=string[] [], "Values"=i32[] [], "Value"=w593, "Name"=w599) -> ("output cluster"=w598:T1)  [unwired: 3 in]
    }
    frame "Analog Input:General Properties:Signal Conditioning:Excitation:Source" {
      n120 = property class="DAQmx Channel"(reference=w601, error in=w607, "ActiveChans"=w602) -> (reference out=w610:refnum<k21>, error out=w606:errorcluster, "AI.Excit.Src"=w603:i32)
      n121 = call-poly <vilib>:"ex_setTdmProperty.vi"("Strings"=string[] ["Internal", "External", "None"], "Values"=i32[] [10200, 10167, 10230], "Value"=w603, "Name"=w609) -> ("output cluster"=w608:T1)  [unwired: 3 in]
    }
    frame "Analog Input:General Properties:Signal Conditioning:Excitation:Value" {
      n122 = property class="DAQmx Channel"(reference=w611, error in=w617, "ActiveChans"=w612) -> (reference out=w620:refnum<k21>, error out=w616:errorcluster, "AI.Excit.Val"=w613:dbl)
      n123 = call-poly <vilib>:"ex_setTdmProperty.vi"("Strings"=string[] [], "Values"=i32[] [], "Value"=w613, "Name"=w619) -> ("output cluster"=w618:T1)  [unwired: 3 in]
    }
    frame "Analog Input:General Properties:Signal Conditioning:Excitation:Advanced:Use Excitation For Scaling" {
      n124 = property class="DAQmx Channel"(reference=w621, error in=w627, "ActiveChans"=w622) -> (reference out=w630:refnum<k21>, error out=w626:errorcluster, "AI.Excit.UseForScaling"=w623:bool)
      n125 = call-poly <vilib>:"ex_setTdmProperty.vi"("Strings"=string[] [], "Values"=i32[] [], "Value"=w623, "Name"=w629) -> ("output cluster"=w628:T1)  [unwired: 3 in]
    }
    frame "Analog Input:General Properties:Signal Conditioning:Excitation:Advanced:Use Multiplexed Excitation" {
      n126 = property class="DAQmx Channel"(reference=w631, error in=w637, "ActiveChans"=w632) -> (reference out=w640:refnum<k21>, error out=w636:errorcluster, "AI.Excit.UseMultiplexed"=w633:bool)
      n127 = call-poly <vilib>:"ex_setTdmProperty.vi"("Strings"=string[] [], "Values"=i32[] [], "Value"=w633, "Name"=w639) -> ("output cluster"=w638:T1)  [unwired: 3 in]
    }
    frame "Analog Input:General Properties:Signal Conditioning:Excitation:Advanced:Actual Excitation Value" {
      n128 = property class="DAQmx Channel"(reference=w641, error in=w647, "ActiveChans"=w642) -> (reference out=w650:refnum<k21>, error out=w646:errorcluster, "AI.Excit.ActualVal"=w643:dbl)
      n129 = call-poly <vilib>:"ex_setTdmProperty.vi"("Strings"=string[] [], "Values"=i32[] [], "Value"=w643, "Name"=w649) -> ("output cluster"=w648:T1)  [unwired: 3 in]
    }
    frame "Analog Input:General Properties:Signal Conditioning:Excitation:Advanced:DC or AC" {
      n130 = property class="DAQmx Channel"(reference=w651, error in=w657, "ActiveChans"=w652) -> (reference out=w660:refnum<k21>, error out=w656:errorcluster, "AI.Excit.DCorAC"=w653:i32)
      n131 = call-poly <vilib>:"ex_setTdmProperty.vi"("Strings"=string[] ["DC", "AC"], "Values"=i32[] [10050, 10045], "Value"=w653, "Name"=w659) -> ("output cluster"=w658:T1)  [unwired: 3 in]
    }
    frame "Analog Input:General Properties:Signal Conditioning:Excitation:Advanced:Voltage or Current" {
      n132 = property class="DAQmx Channel"(reference=w661, error in=w667, "ActiveChans"=w662) -> (reference out=w670:refnum<k21>, error out=w666:errorcluster, "AI.Excit.VoltageOrCurrent"=w663:i32)
      n133 = call-poly <vilib>:"ex_setTdmProperty.vi"("Strings"=string[] ["Voltage", "Current"], "Values"=i32[] [10322, 10134], "Value"=w663, "Name"=w669) -> ("output cluster"=w668:T1)  [unwired: 3 in]
    }
    frame "Analog Input:General Properties:Signal Conditioning:Excitation:AC Excitation:Frequency" {
      n134 = property class="DAQmx Channel"(reference=w671, error in=w677, "ActiveChans"=w672) -> (reference out=w680:refnum<k21>, error out=w676:errorcluster, "AI.ACExcit.Freq"=w673:dbl)
      n135 = call-poly <vilib>:"ex_setTdmProperty.vi"("Strings"=string[] [], "Values"=i32[] [], "Value"=w673, "Name"=w679) -> ("output cluster"=w678:T1)  [unwired: 3 in]
    }
    frame "Analog Input:General Properties:Signal Conditioning:Excitation:AC Excitation:Synchronization Enable" {
      n136 = property class="DAQmx Channel"(reference=w681, error in=w687, "ActiveChans"=w682) -> (reference out=w690:refnum<k21>, error out=w686:errorcluster, "AI.ACExcit.SyncEnable"=w683:bool)
      n137 = call-poly <vilib>:"ex_setTdmProperty.vi"("Strings"=string[] [], "Values"=i32[] [], "Value"=w683, "Name"=w689) -> ("output cluster"=w688:T1)  [unwired: 3 in]
    }
    frame "Analog Input:General Properties:Signal Conditioning:Excitation:AC Excitation:Wire Mode" {
      n138 = property class="DAQmx Channel"(reference=w691, error in=w697, "ActiveChans"=w692) -> (reference out=w700:refnum<k21>, error out=w696:errorcluster, "AI.ACExcit.WireMode"=w693:i32)
      n139 = call-poly <vilib>:"ex_setTdmProperty.vi"("Strings"=string[] ["4-Wire", "5-Wire"], "Values"=i32[] [4, 5], "Value"=w693, "Name"=w699) -> ("output cluster"=w698:T1)  [unwired: 3 in]
    }
    frame "Analog Input:General Properties:Signal Conditioning:Probe/Attenuator:Attenuation Value" {
      n140 = property class="DAQmx Channel"(reference=w701, error in=w707, "ActiveChans"=w702) -> (reference out=w710:refnum<k21>, error out=w706:errorcluster, "AI.Atten"=w703:dbl)
      n141 = call-poly <vilib>:"ex_setTdmProperty.vi"("Strings"=string[] [], "Values"=i32[] [], "Value"=w703, "Name"=w709) -> ("output cluster"=w708:T1)  [unwired: 3 in]
    }
    frame "Analog Input:General Properties:Filter:Analog Lowpass:Enable" {
      n142 = property class="DAQmx Channel"(reference=w711, error in=w717, "ActiveChans"=w712) -> (reference out=w720:refnum<k21>, error out=w716:errorcluster, "AI.Lowpass.Enable"=w713:bool)
      n143 = call-poly <vilib>:"ex_setTdmProperty.vi"("Strings"=string[] [], "Values"=i32[] [], "Value"=w713, "Name"=w719) -> ("output cluster"=w718:T1)  [unwired: 3 in]
    }
    frame "Analog Input:General Properties:Filter:Analog Lowpass:Cutoff Frequency" {
      n144 = property class="DAQmx Channel"(reference=w721, error in=w727, "ActiveChans"=w722) -> (reference out=w730:refnum<k21>, error out=w726:errorcluster, "AI.Lowpass.CutoffFreq"=w723:dbl)
      n145 = call-poly <vilib>:"ex_setTdmProperty.vi"("Strings"=string[] [], "Values"=i32[] [], "Value"=w723, "Name"=w729) -> ("output cluster"=w728:T1)  [unwired: 3 in]
    }
    frame "Analog Input:General Properties:Filter:Analog Lowpass:Advanced:Switched Capacitor:Clock Source" {
      n146 = property class="DAQmx Channel"(reference=w731, error in=w737, "ActiveChans"=w732) -> (reference out=w740:refnum<k21>, error out=w736:errorcluster, "AI.Lowpass.SwitchCap.ClkSrc"=w733:i32)
      n147 = call-poly <vilib>:"ex_setTdmProperty.vi"("Strings"=string[] ["Internal", "External"], "Values"=i32[] [10200, 10167], "Value"=w733, "Name"=w739) -> ("output cluster"=w738:T1)  [unwired: 3 in]
    }
    frame "Analog Input:General Properties:Filter:Analog Lowpass:Advanced:Switched Capacitor:External Clock Frequency" {
      n148 = property class="DAQmx Channel"(reference=w741, error in=w747, "ActiveChans"=w742) -> (reference out=w750:refnum<k21>, error out=w746:errorcluster, "AI.Lowpass.SwitchCap.ExtClkFreq"=w743:dbl)
      n149 = call-poly <vilib>:"ex_setTdmProperty.vi"("Strings"=string[] [], "Values"=i32[] [], "Value"=w743, "Name"=w749) -> ("output cluster"=w748:T1)  [unwired: 3 in]
    }
    frame "Analog Input:General Properties:Filter:Analog Lowpass:Advanced:Switched Capacitor:External Clock Divisor" {
      n150 = property class="DAQmx Channel"(reference=w751, error in=w757, "ActiveChans"=w752) -> (reference out=w760:refnum<k21>, error out=w756:errorcluster, "AI.Lowpass.SwitchCap.ExtClkDiv"=w753:u32)
      n151 = call-poly <vilib>:"ex_setTdmProperty.vi"("Strings"=string[] [], "Values"=i32[] [], "Value"=w753, "Name"=w759) -> ("output cluster"=w758:T1)  [unwired: 3 in]
    }
    frame "Analog Input:General Properties:Filter:Analog Lowpass:Advanced:Switched Capacitor:Output Clock Divisor" {
      n152 = property class="DAQmx Channel"(reference=w761, error in=w767, "ActiveChans"=w762) -> (reference out=w770:refnum<k21>, error out=w766:errorcluster, "AI.Lowpass.SwitchCap.OutClkDiv"=w763:u32)
      n153 = call-poly <vilib>:"ex_setTdmProperty.vi"("Strings"=string[] [], "Values"=i32[] [], "Value"=w763, "Name"=w769) -> ("output cluster"=w768:T1)  [unwired: 3 in]
    }
    frame "Analog Input:General Properties:Digitizer/ADC:Resolution Units" {
      n154 = property class="DAQmx Channel"(reference=w771, error in=w777, "ActiveChans"=w772) -> (reference out=w780:refnum<k21>, error out=w776:errorcluster, "AI.ResolutionUnits"=w773:i32)
      n155 = call-poly <vilib>:"ex_setTdmProperty.vi"("Strings"=string[] ["Bits"], "Values"=i32[] [10109], "Value"=w773, "Name"=w779) -> ("output cluster"=w778:T1)  [unwired: 3 in]
    }
    frame "Analog Input:General Properties:Digitizer/ADC:Resolution Value" {
      n156 = property class="DAQmx Channel"(reference=w781, error in=w787, "ActiveChans"=w782) -> (reference out=w790:refnum<k21>, error out=w786:errorcluster, "AI.Resolution"=w783:dbl)
      n157 = call-poly <vilib>:"ex_setTdmProperty.vi"("Strings"=string[] [], "Values"=i32[] [], "Value"=w783, "Name"=w789) -> ("output cluster"=w788:T1)  [unwired: 3 in]
    }
    frame "Analog Input:General Properties:Digitizer/ADC:Raw Sample Size" {
      n158 = property class="DAQmx Channel"(reference=w791, error in=w797, "ActiveChans"=w792) -> (reference out=w800:refnum<k21>, error out=w796:errorcluster, "AI.RawSampSize"=w793:u32)
      n159 = call-poly <vilib>:"ex_setTdmProperty.vi"("Strings"=string[] [], "Values"=i32[] [], "Value"=w793, "Name"=w799) -> ("output cluster"=w798:T1)  [unwired: 3 in]
    }
    frame "Analog Input:General Properties:Digitizer/ADC:Raw Sample Justification" {
      n160 = property class="DAQmx Channel"(reference=w801, error in=w807, "ActiveChans"=w802) -> (reference out=w810:refnum<k21>, error out=w806:errorcluster, "AI.RawSampJustification"=w803:i32)
      n161 = call-poly <vilib>:"ex_setTdmProperty.vi"("Strings"=string[] ["Right-Justified", "Left-Justified"], "Values"=i32[] [10279, 10209], "Value"=w803, "Name"=w809) -> ("output cluster"=w808:T1)  [unwired: 3 in]
    }
    frame "Analog Input:General Properties:Digitizer/ADC:Dither:Enable" {
      n162 = property class="DAQmx Channel"(reference=w811, error in=w817, "ActiveChans"=w812) -> (reference out=w820:refnum<k21>, error out=w816:errorcluster, "AI.Dither.Enable"=w813:bool)
      n163 = call-poly <vilib>:"ex_setTdmProperty.vi"("Strings"=string[] [], "Values"=i32[] [], "Value"=w813, "Name"=w819) -> ("output cluster"=w818:T1)  [unwired: 3 in]
    }
    frame "Analog Input:General Properties:Channel Calibration:Has Valid Calibration Information" {
      n164 = property class="DAQmx Channel"(reference=w821, error in=w827, "ActiveChans"=w822) -> (reference out=w830:refnum<k21>, error out=w826:errorcluster, "AI.ChanCal.HasValidCalInfo"=w823:bool)
      n165 = call-poly <vilib>:"ex_setTdmProperty.vi"("Strings"=string[] [], "Values"=i32[] [], "Value"=w823, "Name"=w829) -> ("output cluster"=w828:T1)  [unwired: 3 in]
    }
    frame "Analog Input:General Properties:Channel Calibration:Enable Calibration" {
      n166 = property class="DAQmx Channel"(reference=w831, error in=w837, "ActiveChans"=w832) -> (reference out=w840:refnum<k21>, error out=w836:errorcluster, "AI.ChanCal.EnableCal"=w833:bool)
      n167 = call-poly <vilib>:"ex_setTdmProperty.vi"("Strings"=string[] [], "Values"=i32[] [], "Value"=w833, "Name"=w839) -> ("output cluster"=w838:T1)  [unwired: 3 in]
    }
    frame "Analog Input:General Properties:Channel Calibration:Apply Calibration If Expired" {
      n168 = property class="DAQmx Channel"(reference=w841, error in=w847, "ActiveChans"=w842) -> (reference out=w850:refnum<k21>, error out=w846:errorcluster, "AI.ChanCal.ApplyCalIfExp"=w843:bool)
      n169 = call-poly <vilib>:"ex_setTdmProperty.vi"("Strings"=string[] [], "Values"=i32[] [], "Value"=w843, "Name"=w849) -> ("output cluster"=w848:T1)  [unwired: 3 in]
    }
    frame "Analog Input:General Properties:Channel Calibration:Calibration Date" {
      n170 = property class="DAQmx Channel"(reference=w851, error in=w857, "ActiveChans"=w852) -> (reference out=w860:refnum<k21>, error out=w856:errorcluster, "AI.ChanCal.CalDate"=w853:timestamp)
      n171 = call-poly <vilib>:"ex_setTdmProperty.vi"("Strings"=string[] [], "Values"=i32[] [], "Value"=w853, "Name"=w859) -> ("output cluster"=w858:T1)  [unwired: 3 in]
    }
    frame "Analog Input:General Properties:Channel Calibration:Expiration Date" {
      n172 = property class="DAQmx Channel"(reference=w861, error in=w867, "ActiveChans"=w862) -> (reference out=w870:refnum<k21>, error out=w866:errorcluster, "AI.ChanCal.ExpDate"=w863:timestamp)
      n173 = call-poly <vilib>:"ex_setTdmProperty.vi"("Strings"=string[] [], "Values"=i32[] [], "Value"=w863, "Name"=w869) -> ("output cluster"=w868:T1)  [unwired: 3 in]
    }
    frame "Analog Input:General Properties:Channel Calibration:Scaling Parameters:Scale Type" {
      n174 = property class="DAQmx Channel"(reference=w871, error in=w877, "ActiveChans"=w872) -> (reference out=w880:refnum<k21>, error out=w876:errorcluster, "AI.ChanCal.ScaleType"=w873:i32)
      n175 = call-poly <vilib>:"ex_setTdmProperty.vi"("Strings"=string[] ["Polynomial", "Table"], "Values"=i32[] [10449, 10450], "Value"=w873, "Name"=w879) -> ("output cluster"=w878:T1)  [unwired: 3 in]
    }
    frame "Analog Input:General Properties:Channel Calibration:Scaling Parameters:Table:Pre-Scaled Values" {
      n176 = property class="DAQmx Channel"(reference=w881, error in=w887, "ActiveChans"=w882) -> (reference out=w890:refnum<k21>, error out=w886:errorcluster, "AI.ChanCal.Table.PreScaledVals"=w883:dbl[])
      n177 = call-poly <vilib>:"ex_setTdmProperty.vi"("Strings"=string[] [], "Values"=i32[] [], "Value"=w883, "Name"=w889) -> ("output cluster"=w888:T1)  [unwired: 3 in]
    }
    frame "Analog Input:General Properties:Channel Calibration:Scaling Parameters:Table:Scaled Values" {
      n178 = property class="DAQmx Channel"(reference=w891, error in=w897, "ActiveChans"=w892) -> (reference out=w900:refnum<k21>, error out=w896:errorcluster, "AI.ChanCal.Table.ScaledVals"=w893:dbl[])
      n179 = call-poly <vilib>:"ex_setTdmProperty.vi"("Strings"=string[] [], "Values"=i32[] [], "Value"=w893, "Name"=w899) -> ("output cluster"=w898:T1)  [unwired: 3 in]
    }
    frame "Analog Input:General Properties:Channel Calibration:Scaling Parameters:Polynomial:Forward Coefficients" {
      n180 = property class="DAQmx Channel"(reference=w901, error in=w907, "ActiveChans"=w902) -> (reference out=w910:refnum<k21>, error out=w906:errorcluster, "AI.ChanCal.Poly.ForwardCoeff"=w903:dbl[])
      n181 = call-poly <vilib>:"ex_setTdmProperty.vi"("Strings"=string[] [], "Values"=i32[] [], "Value"=w903, "Name"=w909) -> ("output cluster"=w908:T1)  [unwired: 3 in]
    }
    frame "Analog Input:General Properties:Channel Calibration:Scaling Parameters:Polynomial:Reverse Coefficients" {
      n182 = property class="DAQmx Channel"(reference=w911, error in=w917, "ActiveChans"=w912) -> (reference out=w920:refnum<k21>, error out=w916:errorcluster, "AI.ChanCal.Poly.ReverseCoeff"=w913:dbl[])
      n183 = call-poly <vilib>:"ex_setTdmProperty.vi"("Strings"=string[] [], "Values"=i32[] [], "Value"=w913, "Name"=w919) -> ("output cluster"=w918:T1)  [unwired: 3 in]
    }
    frame "Analog Input:General Properties:Channel Calibration:Operator Name" {
      n184 = property class="DAQmx Channel"(reference=w921, error in=w927, "ActiveChans"=w922) -> (reference out=w930:refnum<k21>, error out=w926:errorcluster, "AI.ChanCal.OperatorName"=w923:string)
      n185 = call-poly <vilib>:"ex_setTdmProperty.vi"("Strings"=string[] [], "Values"=i32[] [], "Value"=w923, "Name"=w929) -> ("output cluster"=w928:T1)  [unwired: 3 in]
    }
    frame "Analog Input:General Properties:Channel Calibration:Description" {
      n186 = property class="DAQmx Channel"(reference=w931, error in=w937, "ActiveChans"=w932) -> (reference out=w940:refnum<k21>, error out=w936:errorcluster, "AI.ChanCal.Desc"=w933:string)
      n187 = call-poly <vilib>:"ex_setTdmProperty.vi"("Strings"=string[] [], "Values"=i32[] [], "Value"=w933, "Name"=w939) -> ("output cluster"=w938:T1)  [unwired: 3 in]
    }
    frame "Analog Input:General Properties:Channel Calibration:Verification:Reference Values" {
      n188 = property class="DAQmx Channel"(reference=w941, error in=w947, "ActiveChans"=w942) -> (reference out=w950:refnum<k21>, error out=w946:errorcluster, "AI.ChanCal.Verif.RefVals"=w943:dbl[])
      n189 = call-poly <vilib>:"ex_setTdmProperty.vi"("Strings"=string[] [], "Values"=i32[] [], "Value"=w943, "Name"=w949) -> ("output cluster"=w948:T1)  [unwired: 3 in]
    }
    frame "Analog Input:General Properties:Channel Calibration:Verification:Acquired Values" {
      n190 = property class="DAQmx Channel"(reference=w951, error in=w957, "ActiveChans"=w952) -> (reference out=w960:refnum<k21>, error out=w956:errorcluster, "AI.ChanCal.Verif.AcqVals"=w953:dbl[])
      n191 = call-poly <vilib>:"ex_setTdmProperty.vi"("Strings"=string[] [], "Values"=i32[] [], "Value"=w953, "Name"=w959) -> ("output cluster"=w958:T1)  [unwired: 3 in]
    }
    frame "Analog Input:General Properties:Advanced:Range:High" {
      n192 = property class="DAQmx Channel"(reference=w961, error in=w967, "ActiveChans"=w962) -> (reference out=w970:refnum<k21>, error out=w966:errorcluster, "AI.Rng.High"=w963:dbl)
      n193 = call-poly <vilib>:"ex_setTdmProperty.vi"("Strings"=string[] [], "Values"=i32[] [], "Value"=w963, "Name"=w969) -> ("output cluster"=w968:T1)  [unwired: 3 in]
    }
    frame "Analog Input:General Properties:Advanced:Range:Low" {
      n194 = property class="DAQmx Channel"(reference=w971, error in=w977, "ActiveChans"=w972) -> (reference out=w980:refnum<k21>, error out=w976:errorcluster, "AI.Rng.Low"=w973:dbl)
      n195 = call-poly <vilib>:"ex_setTdmProperty.vi"("Strings"=string[] [], "Values"=i32[] [], "Value"=w973, "Name"=w979) -> ("output cluster"=w978:T1)  [unwired: 3 in]
    }
    frame "Analog Input:General Properties:Advanced:Gain:Gain Value" {
      n196 = property class="DAQmx Channel"(reference=w981, error in=w987, "ActiveChans"=w982) -> (reference out=w990:refnum<k21>, error out=w986:errorcluster, "AI.Gain"=w983:dbl)
      n197 = call-poly <vilib>:"ex_setTdmProperty.vi"("Strings"=string[] [], "Values"=i32[] [], "Value"=w983, "Name"=w989) -> ("output cluster"=w988:T1)  [unwired: 3 in]
    }
    frame "Analog Input:General Properties:Advanced:Sample and Hold Enable" {
      n198 = property class="DAQmx Channel"(reference=w991, error in=w997, "ActiveChans"=w992) -> (reference out=w1000:refnum<k21>, error out=w996:errorcluster, "AI.SampAndHold.Enable"=w993:bool)
      n199 = call-poly <vilib>:"ex_setTdmProperty.vi"("Strings"=string[] [], "Values"=i32[] [], "Value"=w993, "Name"=w999) -> ("output cluster"=w998:T1)  [unwired: 3 in]
    }
    frame "Analog Input:General Properties:Advanced:High Accuracy Settings:Auto Zero Mode" {
      n200 = property class="DAQmx Channel"(reference=w1001, error in=w1007, "ActiveChans"=w1002) -> (reference out=w1010:refnum<k21>, error out=w1006:errorcluster, "AI.AutoZeroMode"=w1003:i32)
      n201 = call-poly <vilib>:"ex_setTdmProperty.vi"("Strings"=string[] ["None", "Once"], "Values"=i32[] [10230, 10244], "Value"=w1003, "Name"=w1009) -> ("output cluster"=w1008:T1)  [unwired: 3 in]
    }
    frame "Analog Input:General Properties:Advanced:Data Transfer and Memory:Data Transfer Mechanism" {
      n202 = property class="DAQmx Channel"(reference=w1011, error in=w1017, "ActiveChans"=w1012) -> (reference out=w1020:refnum<k21>, error out=w1016:errorcluster, "AI.DataXferMech"=w1013:i32)
      n203 = call-poly <vilib>:"ex_setTdmProperty.vi"("Strings"=string[] ["DMA", "Interrupts", "Programmed I/O"], "Values"=i32[] [10054, 10204, 10264], "Value"=w1013, "Name"=w1019) -> ("output cluster"=w1018:T1)  [unwired: 3 in]
    }
    frame "Analog Input:General Properties:Advanced:Data Transfer and Memory:Data Transfer Request Condition" {
      n204 = property class="DAQmx Channel"(reference=w1021, error in=w1027, "ActiveChans"=w1022) -> (reference out=w1030:refnum<k21>, error out=w1026:errorcluster, "AI.DataXferReqCond"=w1023:i32)
      n205 = call-poly <vilib>:"ex_setTdmProperty.vi"("Strings"=string[] ["Onboard Memory More than Half Full", "Onboard Memory Not Empty", "Onboard Memory Custom Threshold", "When Acquisition Complete"], "Values"=i32[] [10237, 10241, 12577, 12546], "Value"=w1023, "Name"=w1029) -> ("output cluster"=w1028:T1)  [unwired: 3 in]
    }
    frame "Analog Input:General Properties:Advanced:Data Transfer and Memory:Data Transfer Custom Threshold" {
      n206 = property class="DAQmx Channel"(reference=w1031, error in=w1037, "ActiveChans"=w1032) -> (reference out=w1040:refnum<k21>, error out=w1036:errorcluster, "AI.DataXferCustomThreshold"=w1033:u32)
      n207 = call-poly <vilib>:"ex_setTdmProperty.vi"("Strings"=string[] [], "Values"=i32[] [], "Value"=w1033, "Name"=w1039) -> ("output cluster"=w1038:T1)  [unwired: 3 in]
    }
    frame "Analog Input:General Properties:Advanced:Data Transfer and Memory:Memory Mapping for Programmed IO Enable" {
      n208 = property class="DAQmx Channel"(reference=w1041, error in=w1047, "ActiveChans"=w1042) -> (reference out=w1050:refnum<k21>, error out=w1046:errorcluster, "AI.MemMapEnable"=w1043:bool)
      n209 = call-poly <vilib>:"ex_setTdmProperty.vi"("Strings"=string[] [], "Values"=i32[] [], "Value"=w1043, "Name"=w1049) -> ("output cluster"=w1048:T1)  [unwired: 3 in]
    }
    frame "Analog Input:General Properties:Advanced:Data Transfer and Memory:Compression:Raw Data Compression Type" {
      n210 = property class="DAQmx Channel"(reference=w1051, error in=w1057, "ActiveChans"=w1052) -> (reference out=w1060:refnum<k21>, error out=w1056:errorcluster, "AI.RawDataCompressionType"=w1053:i32)
      n211 = call-poly <vilib>:"ex_setTdmProperty.vi"("Strings"=string[] ["None", "Lossless Packing", "Lossy LSB Removal"], "Values"=i32[] [10230, 12555, 12556], "Value"=w1053, "Name"=w1059) -> ("output cluster"=w1058:T1)  [unwired: 3 in]
    }
    frame "Analog Input:General Properties:Advanced:Data Transfer and Memory:Compression:Lossy LSB Removal:Compressed Sample Size" {
      n212 = property class="DAQmx Channel"(reference=w1061, error in=w1067, "ActiveChans"=w1062) -> (reference out=w1070:refnum<k21>, error out=w1066:errorcluster, "AI.LossyLSBRemoval.CompressedSampSize"=w1063:u32)
      n213 = call-poly <vilib>:"ex_setTdmProperty.vi"("Strings"=string[] [], "Values"=i32[] [], "Value"=w1063, "Name"=w1069) -> ("output cluster"=w1068:T1)  [unwired: 3 in]
    }
    frame "Analog Input:General Properties:Advanced:Device Scaling Coefficients:Device Scaling Coefficients" {
      n214 = property class="DAQmx Channel"(reference=w1071, error in=w1077, "ActiveChans"=w1072) -> (reference out=w1080:refnum<k21>, error out=w1076:errorcluster, "AI.DevScalingCoeff"=w1073:dbl[])
      n215 = call-poly <vilib>:"ex_setTdmProperty.vi"("Strings"=string[] [], "Values"=i32[] [], "Value"=w1073, "Name"=w1079) -> ("output cluster"=w1078:T1)  [unwired: 3 in]
    }
    frame "Analog Input:General Properties:Advanced:Enhanced Alias Rejection Enable" {
      n216 = property class="DAQmx Channel"(reference=w1081, error in=w1087, "ActiveChans"=w1082) -> (reference out=w1090:refnum<k21>, error out=w1086:errorcluster, "AI.EnhancedAliasRejectionEnable"=w1083:bool)
      n217 = call-poly <vilib>:"ex_setTdmProperty.vi"("Strings"=string[] [], "Values"=i32[] [], "Value"=w1083, "Name"=w1089) -> ("output cluster"=w1088:T1)  [unwired: 3 in]
    }
    frame "Analog Output:Maximum Value" {
      n218 = property class="DAQmx Channel"(reference=w1091, error in=w1097, "ActiveChans"=w1092) -> (reference out=w1100:refnum<k21>, error out=w1096:errorcluster, "AO.Max"=w1093:dbl)
      n219 = call-poly <vilib>:"ex_setTdmProperty.vi"("Strings"=string[] [], "Values"=i32[] [], "Value"=w1093, "Name"=w1099) -> ("output cluster"=w1098:T1)  [unwired: 3 in]
    }
    frame "Analog Output:Minimum Value" {
      n220 = property class="DAQmx Channel"(reference=w1101, error in=w1107, "ActiveChans"=w1102) -> (reference out=w1110:refnum<k21>, error out=w1106:errorcluster, "AO.Min"=w1103:dbl)
      n221 = call-poly <vilib>:"ex_setTdmProperty.vi"("Strings"=string[] [], "Values"=i32[] [], "Value"=w1103, "Name"=w1109) -> ("output cluster"=w1108:T1)  [unwired: 3 in]
    }
    frame "Analog Output:Custom Scale Name" {
      n222 = property class="DAQmx Channel"(reference=w1111, error in=w1117, "ActiveChans"=w1112) -> (reference out=w1120:refnum<k21>, error out=w1116:errorcluster, "AO.CustomScaleName"=w1113:tag)
      n223 = call-poly <vilib>:"ex_setTdmProperty.vi"("Strings"=string[] [], "Values"=i32[] [], "Value"=w1113, "Name"=w1119) -> ("output cluster"=w1118:T1)  [unwired: 3 in]
    }
    frame "Analog Output:Output Type" {
      n224 = property class="DAQmx Channel"(reference=w1121, error in=w1127, "ActiveChans"=w1122) -> (reference out=w1130:refnum<k21>, error out=w1126:errorcluster, "AO.OutputType"=w1123:i32)
      n225 = call-poly <vilib>:"ex_setTdmProperty.vi"("Strings"=string[] ["Voltage", "Current"], "Values"=i32[] [10322, 10134], "Value"=w1123, "Name"=w1129) -> ("output cluster"=w1128:T1)  [unwired: 3 in]
    }
    frame "Analog Output:Voltage:Units" {
      n226 = property class="DAQmx Channel"(reference=w1131, error in=w1137, "ActiveChans"=w1132) -> (reference out=w1140:refnum<k21>, error out=w1136:errorcluster, "AO.Voltage.Units"=w1133:i32)
      n227 = call-poly <vilib>:"ex_setTdmProperty.vi"("Strings"=string[] ["Volts", "From Custom Scale"], "Values"=i32[] [10348, 10065], "Value"=w1133, "Name"=w1139) -> ("output cluster"=w1138:T1)  [unwired: 3 in]
    }
    frame "Analog Output:Current:Units" {
      n228 = property class="DAQmx Channel"(reference=w1141, error in=w1147, "ActiveChans"=w1142) -> (reference out=w1150:refnum<k21>, error out=w1146:errorcluster, "AO.Current.Units"=w1143:i32)
      n229 = call-poly <vilib>:"ex_setTdmProperty.vi"("Strings"=string[] ["Amps", "From Custom Scale", "From TEDS"], "Values"=i32[] [10342, 10065, 12516], "Value"=w1143, "Name"=w1149) -> ("output cluster"=w1148:T1)  [unwired: 3 in]
    }
    frame "Analog Output:General Properties:Output Configuration:Output Impedance" {
      n230 = property class="DAQmx Channel"(reference=w1151, error in=w1157, "ActiveChans"=w1152) -> (reference out=w1160:refnum<k21>, error out=w1156:errorcluster, "AO.OutputImpedance"=w1153:dbl)
      n231 = call-poly <vilib>:"ex_setTdmProperty.vi"("Strings"=string[] [], "Values"=i32[] [], "Value"=w1153, "Name"=w1159) -> ("output cluster"=w1158:T1)  [unwired: 3 in]
    }
    frame "Analog Output:General Properties:Output Configuration:Load Impedance" {
      n232 = property class="DAQmx Channel"(reference=w1161, error in=w1167, "ActiveChans"=w1162) -> (reference out=w1170:refnum<k21>, error out=w1166:errorcluster, "AO.LoadImpedance"=w1163:dbl)
      n233 = call-poly <vilib>:"ex_setTdmProperty.vi"("Strings"=string[] [], "Values"=i32[] [], "Value"=w1163, "Name"=w1169) -> ("output cluster"=w1168:T1)  [unwired: 3 in]
    }
    frame "Analog Output:General Properties:Output Configuration:Idle Output Behavior" {
      n234 = property class="DAQmx Channel"(reference=w1171, error in=w1177, "ActiveChans"=w1172) -> (reference out=w1180:refnum<k21>, error out=w1176:errorcluster, "AO.IdleOutputBehavior"=w1173:i32)
      n235 = call-poly <vilib>:"ex_setTdmProperty.vi"("Strings"=string[] ["Zero Volts", "High Impedance", "Maintain Existing Value"], "Values"=i32[] [12526, 12527, 12528], "Value"=w1173, "Name"=w1179) -> ("output cluster"=w1178:T1)  [unwired: 3 in]
    }
    frame "Analog Output:General Properties:Output Configuration:Terminal Configuration" {
      n236 = property class="DAQmx Channel"(reference=w1181, error in=w1187, "ActiveChans"=w1182) -> (reference out=w1190:refnum<k21>, error out=w1186:errorcluster, "AO.TermCfg"=w1183:i32)
      n237 = call-poly <vilib>:"ex_setTdmProperty.vi"("Strings"=string[] ["RSE", "Differential", "Pseudodifferential"], "Values"=i32[] [10083, 10106, 12529], "Value"=w1183, "Name"=w1189) -> ("output cluster"=w1188:T1)  [unwired: 3 in]
    }
    frame "Analog Output:General Properties:DAC:Resolution Units" {
      n238 = property class="DAQmx Channel"(reference=w1191, error in=w1197, "ActiveChans"=w1192) -> (reference out=w1200:refnum<k21>, error out=w1196:errorcluster, "AO.ResolutionUnits"=w1193:i32)
      n239 = call-poly <vilib>:"ex_setTdmProperty.vi"("Strings"=string[] ["Bits"], "Values"=i32[] [10109], "Value"=w1193, "Name"=w1199) -> ("output cluster"=w1198:T1)  [unwired: 3 in]
    }
    frame "Analog Output:General Properties:DAC:Resolution Value" {
      n240 = property class="DAQmx Channel"(reference=w1201, error in=w1207, "ActiveChans"=w1202) -> (reference out=w1210:refnum<k21>, error out=w1206:errorcluster, "AO.Resolution"=w1203:dbl)
      n241 = call-poly <vilib>:"ex_setTdmProperty.vi"("Strings"=string[] [], "Values"=i32[] [], "Value"=w1203, "Name"=w1209) -> ("output cluster"=w1208:T1)  [unwired: 3 in]
    }
    frame "Analog Output:General Properties:DAC:Range:High" {
      n242 = property class="DAQmx Channel"(reference=w1211, error in=w1217, "ActiveChans"=w1212) -> (reference out=w1220:refnum<k21>, error out=w1216:errorcluster, "AO.DAC.Rng.High"=w1213:dbl)
      n243 = call-poly <vilib>:"ex_setTdmProperty.vi"("Strings"=string[] [], "Values"=i32[] [], "Value"=w1213, "Name"=w1219) -> ("output cluster"=w1218:T1)  [unwired: 3 in]
    }
    frame "Analog Output:General Properties:DAC:Range:Low" {
      n244 = property class="DAQmx Channel"(reference=w1221, error in=w1227, "ActiveChans"=w1222) -> (reference out=w1230:refnum<k21>, error out=w1226:errorcluster, "AO.DAC.Rng.Low"=w1223:dbl)
      n245 = call-poly <vilib>:"ex_setTdmProperty.vi"("Strings"=string[] [], "Values"=i32[] [], "Value"=w1223, "Name"=w1229) -> ("output cluster"=w1228:T1)  [unwired: 3 in]
    }
    frame "Analog Output:General Properties:DAC:Reference Voltage:Connect DAC Reference to Ground" {
      n246 = property class="DAQmx Channel"(reference=w1231, error in=w1237, "ActiveChans"=w1232) -> (reference out=w1240:refnum<k21>, error out=w1236:errorcluster, "AO.DAC.Ref.ConnToGnd"=w1233:bool)
      n247 = call-poly <vilib>:"ex_setTdmProperty.vi"("Strings"=string[] [], "Values"=i32[] [], "Value"=w1233, "Name"=w1239) -> ("output cluster"=w1238:T1)  [unwired: 3 in]
    }
    frame "Analog Output:General Properties:DAC:Reference Voltage:Allow Connecting DAC Reference to Ground at Runtime" {
      n248 = property class="DAQmx Channel"(reference=w1241, error in=w1247, "ActiveChans"=w1242) -> (reference out=w1250:refnum<k21>, error out=w1246:errorcluster, "AO.DAC.Ref.AllowConnToGnd"=w1243:bool)
      n249 = call-poly <vilib>:"ex_setTdmProperty.vi"("Strings"=string[] [], "Values"=i32[] [], "Value"=w1243, "Name"=w1249) -> ("output cluster"=w1248:T1)  [unwired: 3 in]
    }
    frame "Analog Output:General Properties:DAC:Reference Voltage:Source" {
      n250 = property class="DAQmx Channel"(reference=w1251, error in=w1257, "ActiveChans"=w1252) -> (reference out=w1260:refnum<k21>, error out=w1256:errorcluster, "AO.DAC.Ref.Src"=w1253:i32)
      n251 = call-poly <vilib>:"ex_setTdmProperty.vi"("Strings"=string[] ["Internal", "External"], "Values"=i32[] [10200, 10167], "Value"=w1253, "Name"=w1259) -> ("output cluster"=w1258:T1)  [unwired: 3 in]
    }
    frame "Analog Output:General Properties:DAC:Reference Voltage:External Source" {
      n252 = property class="DAQmx Channel"(reference=w1261, error in=w1267, "ActiveChans"=w1262) -> (reference out=w1270:refnum<k21>, error out=w1266:errorcluster, "AO.DAC.Ref.ExtSrc"=w1263:string)
      n253 = call-poly <vilib>:"ex_setTdmProperty.vi"("Strings"=string[] [], "Values"=i32[] [], "Value"=w1263, "Name"=w1269) -> ("output cluster"=w1268:T1)  [unwired: 3 in]
    }
    frame "Analog Output:General Properties:DAC:Reference Voltage:Value" {
      n254 = property class="DAQmx Channel"(reference=w1271, error in=w1277, "ActiveChans"=w1272) -> (reference out=w1280:refnum<k21>, error out=w1276:errorcluster, "AO.DAC.Ref.Val"=w1273:dbl)
      n255 = call-poly <vilib>:"ex_setTdmProperty.vi"("Strings"=string[] [], "Values"=i32[] [], "Value"=w1273, "Name"=w1279) -> ("output cluster"=w1278:T1)  [unwired: 3 in]
    }
    frame "Analog Output:General Properties:DAC:Offset Voltage:Source" {
      n256 = property class="DAQmx Channel"(reference=w1281, error in=w1287, "ActiveChans"=w1282) -> (reference out=w1290:refnum<k21>, error out=w1286:errorcluster, "AO.DAC.Offset.Src"=w1283:i32)
      n257 = call-poly <vilib>:"ex_setTdmProperty.vi"("Strings"=string[] ["Internal", "External"], "Values"=i32[] [10200, 10167], "Value"=w1283, "Name"=w1289) -> ("output cluster"=w1288:T1)  [unwired: 3 in]
    }
    frame "Analog Output:General Properties:DAC:Offset Voltage:External Source" {
      n258 = property class="DAQmx Channel"(reference=w1291, error in=w1297, "ActiveChans"=w1292) -> (reference out=w1300:refnum<k21>, error out=w1296:errorcluster, "AO.DAC.Offset.ExtSrc"=w1293:string)
      n259 = call-poly <vilib>:"ex_setTdmProperty.vi"("Strings"=string[] [], "Values"=i32[] [], "Value"=w1293, "Name"=w1299) -> ("output cluster"=w1298:T1)  [unwired: 3 in]
    }
    frame "Analog Output:General Properties:DAC:Offset Voltage:Value" {
      n260 = property class="DAQmx Channel"(reference=w1301, error in=w1307, "ActiveChans"=w1302) -> (reference out=w1310:refnum<k21>, error out=w1306:errorcluster, "AO.DAC.Offset.Val"=w1303:dbl)
      n261 = call-poly <vilib>:"ex_setTdmProperty.vi"("Strings"=string[] [], "Values"=i32[] [], "Value"=w1303, "Name"=w1309) -> ("output cluster"=w1308:T1)  [unwired: 3 in]
    }
    frame "Analog Output:General Properties:DAC:Reglitching Enable" {
      n262 = property class="DAQmx Channel"(reference=w1311, error in=w1317, "ActiveChans"=w1312) -> (reference out=w1320:refnum<k21>, error out=w1316:errorcluster, "AO.ReglitchEnable"=w1313:bool)
      n263 = call-poly <vilib>:"ex_setTdmProperty.vi"("Strings"=string[] [], "Values"=i32[] [], "Value"=w1313, "Name"=w1319) -> ("output cluster"=w1318:T1)  [unwired: 3 in]
    }
    frame "Analog Output:General Properties:Advanced:Gain:Gain Value" {
      n264 = property class="DAQmx Channel"(reference=w1321, error in=w1327, "ActiveChans"=w1322) -> (reference out=w1330:refnum<k21>, error out=w1326:errorcluster, "AO.Gain"=w1323:dbl)
      n265 = call-poly <vilib>:"ex_setTdmProperty.vi"("Strings"=string[] [], "Values"=i32[] [], "Value"=w1323, "Name"=w1329) -> ("output cluster"=w1328:T1)  [unwired: 3 in]
    }
    frame "Analog Output:General Properties:Advanced:Data Transfer and Memory:Use Only Onboard Memory" {
      n266 = property class="DAQmx Channel"(reference=w1331, error in=w1337, "ActiveChans"=w1332) -> (reference out=w1340:refnum<k21>, error out=w1336:errorcluster, "AO.UseOnlyOnBrdMem"=w1333:bool)
      n267 = call-poly <vilib>:"ex_setTdmProperty.vi"("Strings"=string[] [], "Values"=i32[] [], "Value"=w1333, "Name"=w1339) -> ("output cluster"=w1338:T1)  [unwired: 3 in]
    }
    frame "Analog Output:General Properties:Advanced:Data Transfer and Memory:Data Transfer Mechanism" {
      n268 = property class="DAQmx Channel"(reference=w1341, error in=w1347, "ActiveChans"=w1342) -> (reference out=w1350:refnum<k21>, error out=w1346:errorcluster, "AO.DataXferMech"=w1343:i32)
      n269 = call-poly <vilib>:"ex_setTdmProperty.vi"("Strings"=string[] ["DMA", "Interrupts", "Programmed I/O"], "Values"=i32[] [10054, 10204, 10264], "Value"=w1343, "Name"=w1349) -> ("output cluster"=w1348:T1)  [unwired: 3 in]
    }
    frame "Analog Output:General Properties:Advanced:Data Transfer and Memory:Data Transfer Request Condition" {
      n270 = property class="DAQmx Channel"(reference=w1351, error in=w1357, "ActiveChans"=w1352) -> (reference out=w1360:refnum<k21>, error out=w1356:errorcluster, "AO.DataXferReqCond"=w1353:i32)
      n271 = call-poly <vilib>:"ex_setTdmProperty.vi"("Strings"=string[] ["Onboard Memory Empty", "Onboard Memory Half Full or Less", "Onboard Memory Less than Full"], "Values"=i32[] [10235, 10239, 10242], "Value"=w1353, "Name"=w1359) -> ("output cluster"=w1358:T1)  [unwired: 3 in]
    }
    frame "Analog Output:General Properties:Advanced:Data Transfer and Memory:Memory Mapping for Programmed IO Enable" {
      n272 = property class="DAQmx Channel"(reference=w1361, error in=w1367, "ActiveChans"=w1362) -> (reference out=w1370:refnum<k21>, error out=w1366:errorcluster, "AO.MemMapEnable"=w1363:bool)
      n273 = call-poly <vilib>:"ex_setTdmProperty.vi"("Strings"=string[] [], "Values"=i32[] [], "Value"=w1363, "Name"=w1369) -> ("output cluster"=w1368:T1)  [unwired: 3 in]
    }
    frame "Analog Output:General Properties:Advanced:Device Scaling Coefficients:Device Scaling Coefficients" {
      n274 = property class="DAQmx Channel"(reference=w1371, error in=w1377, "ActiveChans"=w1372) -> (reference out=w1380:refnum<k21>, error out=w1376:errorcluster, "AO.DevScalingCoeff"=w1373:dbl[])
      n275 = call-poly <vilib>:"ex_setTdmProperty.vi"("Strings"=string[] [], "Values"=i32[] [], "Value"=w1373, "Name"=w1379) -> ("output cluster"=w1378:T1)  [unwired: 3 in]
    }
    frame "Analog Output:General Properties:Advanced:Enhanced Image Rejection Enable" {
      n276 = property class="DAQmx Channel"(reference=w1381, error in=w1387, "ActiveChans"=w1382) -> (reference out=w1390:refnum<k21>, error out=w1386:errorcluster, "AO.EnhancedImageRejectionEnable"=w1383:bool)
      n277 = call-poly <vilib>:"ex_setTdmProperty.vi"("Strings"=string[] [], "Values"=i32[] [], "Value"=w1383, "Name"=w1389) -> ("output cluster"=w1388:T1)  [unwired: 3 in]
    }
    frame "Digital Input:Invert Lines" {
      n278 = property class="DAQmx Channel"(reference=w1391, error in=w1397, "ActiveChans"=w1392) -> (reference out=w1400:refnum<k21>, error out=w1396:errorcluster, "DI.InvertLines"=w1393:bool)
      n279 = call-poly <vilib>:"ex_setTdmProperty.vi"("Strings"=string[] [], "Values"=i32[] [], "Value"=w1393, "Name"=w1399) -> ("output cluster"=w1398:T1)  [unwired: 3 in]
    }
    frame "Digital Input:Number of Lines" {
      n280 = property class="DAQmx Channel"(reference=w1401, error in=w1407, "ActiveChans"=w1402) -> (reference out=w1410:refnum<k21>, error out=w1406:errorcluster, "DI.NumLines"=w1403:u32)
      n281 = call-poly <vilib>:"ex_setTdmProperty.vi"("Strings"=string[] [], "Values"=i32[] [], "Value"=w1403, "Name"=w1409) -> ("output cluster"=w1408:T1)  [unwired: 3 in]
    }
    frame "Digital Input:Digital Filter:Enable" {
      n282 = property class="DAQmx Channel"(reference=w1411, error in=w1417, "ActiveChans"=w1412) -> (reference out=w1420:refnum<k21>, error out=w1416:errorcluster, "DI.DigFltr.Enable"=w1413:bool)
      n283 = call-poly <vilib>:"ex_setTdmProperty.vi"("Strings"=string[] [], "Values"=i32[] [], "Value"=w1413, "Name"=w1419) -> ("output cluster"=w1418:T1)  [unwired: 3 in]
    }
    frame "Digital Input:Digital Filter:Minimum Pulse Width" {
      n284 = property class="DAQmx Channel"(reference=w1421, error in=w1427, "ActiveChans"=w1422) -> (reference out=w1430:refnum<k21>, error out=w1426:errorcluster, "DI.DigFltr.MinPulseWidth"=w1423:dbl)
      n285 = call-poly <vilib>:"ex_setTdmProperty.vi"("Strings"=string[] [], "Values"=i32[] [], "Value"=w1423, "Name"=w1429) -> ("output cluster"=w1428:T1)  [unwired: 3 in]
    }
    frame "Digital Input:Tristate" {
      n286 = property class="DAQmx Channel"(reference=w1431, error in=w1437, "ActiveChans"=w1432) -> (reference out=w1440:refnum<k21>, error out=w1436:errorcluster, "DI.Tristate"=w1433:bool)
      n287 = call-poly <vilib>:"ex_setTdmProperty.vi"("Strings"=string[] [], "Values"=i32[] [], "Value"=w1433, "Name"=w1439) -> ("output cluster"=w1438:T1)  [unwired: 3 in]
    }
    frame "Digital Input:General Properties:Advanced:Data Transfer and Memory:Data Transfer Mechanism" {
      n288 = property class="DAQmx Channel"(reference=w1441, error in=w1447, "ActiveChans"=w1442) -> (reference out=w1450:refnum<k21>, error out=w1446:errorcluster, "DI.DataXferMech"=w1443:i32)
      n289 = call-poly <vilib>:"ex_setTdmProperty.vi"("Strings"=string[] ["DMA", "Interrupts", "Programmed I/O"], "Values"=i32[] [10054, 10204, 10264], "Value"=w1443, "Name"=w1449) -> ("output cluster"=w1448:T1)  [unwired: 3 in]
    }
    frame "Digital Input:General Properties:Advanced:Data Transfer and Memory:Data Transfer Request Condition" {
      n290 = property class="DAQmx Channel"(reference=w1451, error in=w1457, "ActiveChans"=w1452) -> (reference out=w1460:refnum<k21>, error out=w1456:errorcluster, "DI.DataXferReqCond"=w1453:i32)
      n291 = call-poly <vilib>:"ex_setTdmProperty.vi"("Strings"=string[] ["Onboard Memory More than Half Full", "Onboard Memory Not Empty", "Onboard Memory Custom Threshold", "When Acquisition Complete"], "Values"=i32[] [10237, 10241, 12577, 12546], "Value"=w1453, "Name"=w1459) -> ("output cluster"=w1458:T1)  [unwired: 3 in]
    }
    frame "Digital Output:Output Drive Type" {
      n292 = property class="DAQmx Channel"(reference=w1461, error in=w1467, "ActiveChans"=w1462) -> (reference out=w1470:refnum<k21>, error out=w1466:errorcluster, "DO.OutputDriveType"=w1463:i32)
      n293 = call-poly <vilib>:"ex_setTdmProperty.vi"("Strings"=string[] ["Active Drive", "Open Collector"], "Values"=i32[] [12573, 12574], "Value"=w1463, "Name"=w1469) -> ("output cluster"=w1468:T1)  [unwired: 3 in]
    }
    frame "Digital Output:Invert Lines" {
      n294 = property class="DAQmx Channel"(reference=w1471, error in=w1477, "ActiveChans"=w1472) -> (reference out=w1480:refnum<k21>, error out=w1476:errorcluster, "DO.InvertLines"=w1473:bool)
      n295 = call-poly <vilib>:"ex_setTdmProperty.vi"("Strings"=string[] [], "Values"=i32[] [], "Value"=w1473, "Name"=w1479) -> ("output cluster"=w1478:T1)  [unwired: 3 in]
    }
    frame "Digital Output:Number of Lines" {
      n296 = property class="DAQmx Channel"(reference=w1481, error in=w1487, "ActiveChans"=w1482) -> (reference out=w1490:refnum<k21>, error out=w1486:errorcluster, "DO.NumLines"=w1483:u32)
      n297 = call-poly <vilib>:"ex_setTdmProperty.vi"("Strings"=string[] [], "Values"=i32[] [], "Value"=w1483, "Name"=w1489) -> ("output cluster"=w1488:T1)  [unwired: 3 in]
    }
    frame "Digital Output:Tristate" {
      n298 = property class="DAQmx Channel"(reference=w1491, error in=w1497, "ActiveChans"=w1492) -> (reference out=w1500:refnum<k21>, error out=w1496:errorcluster, "DO.Tristate"=w1493:bool)
      n299 = call-poly <vilib>:"ex_setTdmProperty.vi"("Strings"=string[] [], "Values"=i32[] [], "Value"=w1493, "Name"=w1499) -> ("output cluster"=w1498:T1)  [unwired: 3 in]
    }
    frame "Digital Output:General Properties:Advanced:Data Transfer and Memory:Use Only Onboard Memory" {
      n300 = property class="DAQmx Channel"(reference=w1501, error in=w1507, "ActiveChans"=w1502) -> (reference out=w1510:refnum<k21>, error out=w1506:errorcluster, "DO.UseOnlyOnBrdMem"=w1503:bool)
      n301 = call-poly <vilib>:"ex_setTdmProperty.vi"("Strings"=string[] [], "Values"=i32[] [], "Value"=w1503, "Name"=w1509) -> ("output cluster"=w1508:T1)  [unwired: 3 in]
    }
    frame "Digital Output:General Properties:Advanced:Data Transfer and Memory:Data Transfer Mechanism" {
      n302 = property class="DAQmx Channel"(reference=w1511, error in=w1517, "ActiveChans"=w1512) -> (reference out=w1520:refnum<k21>, error out=w1516:errorcluster, "DO.DataXferMech"=w1513:i32)
      n303 = call-poly <vilib>:"ex_setTdmProperty.vi"("Strings"=string[] ["DMA", "Interrupts", "Programmed I/O"], "Values"=i32[] [10054, 10204, 10264], "Value"=w1513, "Name"=w1519) -> ("output cluster"=w1518:T1)  [unwired: 3 in]
    }
    frame "Digital Output:General Properties:Advanced:Data Transfer and Memory:Data Transfer Request Condition" {
      n304 = property class="DAQmx Channel"(reference=w1521, error in=w1527, "ActiveChans"=w1522) -> (reference out=w1530:refnum<k21>, error out=w1526:errorcluster, "DO.DataXferReqCond"=w1523:i32)
      n305 = call-poly <vilib>:"ex_setTdmProperty.vi"("Strings"=string[] ["Onboard Memory Empty", "Onboard Memory Half Full or Less", "Onboard Memory Less than Full"], "Values"=i32[] [10235, 10239, 10242], "Value"=w1523, "Name"=w1529) -> ("output cluster"=w1528:T1)  [unwired: 3 in]
    }
    frame "Counter Input:Maximum Value" {
      n306 = property class="DAQmx Channel"(reference=w1531, error in=w1537, "ActiveChans"=w1532) -> (reference out=w1540:refnum<k21>, error out=w1536:errorcluster, "CI.Max"=w1533:dbl)
      n307 = call-poly <vilib>:"ex_setTdmProperty.vi"("Strings"=string[] [], "Values"=i32[] [], "Value"=w1533, "Name"=w1539) -> ("output cluster"=w1538:T1)  [unwired: 3 in]
    }
    frame "Counter Input:Minimum Value" {
      n308 = property class="DAQmx Channel"(reference=w1541, error in=w1547, "ActiveChans"=w1542) -> (reference out=w1550:refnum<k21>, error out=w1546:errorcluster, "CI.Min"=w1543:dbl)
      n309 = call-poly <vilib>:"ex_setTdmProperty.vi"("Strings"=string[] [], "Values"=i32[] [], "Value"=w1543, "Name"=w1549) -> ("output cluster"=w1548:T1)  [unwired: 3 in]
    }
    frame "Counter Input:Custom Scale Name" {
      n310 = property class="DAQmx Channel"(reference=w1551, error in=w1557, "ActiveChans"=w1552) -> (reference out=w1560:refnum<k21>, error out=w1556:errorcluster, "CI.CustomScaleName"=w1553:tag)
      n311 = call-poly <vilib>:"ex_setTdmProperty.vi"("Strings"=string[] [], "Values"=i32[] [], "Value"=w1553, "Name"=w1559) -> ("output cluster"=w1558:T1)  [unwired: 3 in]
    }
    frame "Counter Input:Measurement Type" {
      n312 = property class="DAQmx Channel"(reference=w1561, error in=w1567, "ActiveChans"=w1562) -> (reference out=w1570:refnum<k21>, error out=w1566:errorcluster, "CI.MeasType"=w1563:i32)
      n313 = call-poly <vilib>:"ex_setTdmProperty.vi"("Strings"=string[] ["Count Edges", "Frequency", "Period", "Pulse Width", "Semi Period", "Position:Angular Encoder", "Position:Linear Encoder", "Two Edge Separation", "GPS Timestamp"], "Values"=i32[] [10125, 10179, 10256, 10359, 10289, 10360, 10361, 10267, 10362], "Value"=w1563, "Name"=w1569) -> ("output cluster"=w1568:T1)  [unwired: 3 in]
    }
    frame "Counter Input:Frequency:Units" {
      n314 = property class="DAQmx Channel"(reference=w1571, error in=w1577, "ActiveChans"=w1572) -> (reference out=w1580:refnum<k21>, error out=w1576:errorcluster, "CI.Freq.Units"=w1573:i32)
      n315 = call-poly <vilib>:"ex_setTdmProperty.vi"("Strings"=string[] ["Hz", "Ticks", "From Custom Scale"], "Values"=i32[] [10373, 10304, 10065], "Value"=w1573, "Name"=w1579) -> ("output cluster"=w1578:T1)  [unwired: 3 in]
    }
    frame "Counter Input:Frequency:Input Terminal" {
      n316 = property class="DAQmx Channel"(reference=w1581, error in=w1587, "ActiveChans"=w1582) -> (reference out=w1590:refnum<k21>, error out=w1586:errorcluster, "CI.Freq.Term"=w1583:tag)
      n317 = call-poly <vilib>:"ex_setTdmProperty.vi"("Strings"=string[] [], "Values"=i32[] [], "Value"=w1583, "Name"=w1589) -> ("output cluster"=w1588:T1)  [unwired: 3 in]
    }
    frame "Counter Input:Frequency:Starting Edge" {
      n318 = property class="DAQmx Channel"(reference=w1591, error in=w1597, "ActiveChans"=w1592) -> (reference out=w1600:refnum<k21>, error out=w1596:errorcluster, "CI.Freq.StartingEdge"=w1593:i32)
      n319 = call-poly <vilib>:"ex_setTdmProperty.vi"("Strings"=string[] ["Rising", "Falling"], "Values"=i32[] [10280, 10171], "Value"=w1593, "Name"=w1599) -> ("output cluster"=w1598:T1)  [unwired: 3 in]
    }
    frame "Counter Input:Frequency:Measurement Specifications:Method" {
      n320 = property class="DAQmx Channel"(reference=w1601, error in=w1607, "ActiveChans"=w1602) -> (reference out=w1610:refnum<k21>, error out=w1606:errorcluster, "CI.Freq.MeasMeth"=w1603:i32)
      n321 = call-poly <vilib>:"ex_setTdmProperty.vi"("Strings"=string[] ["Low Frequency with 1 Counter", "High Frequency with 2 Counters", "Large Range with 2 Counters"], "Values"=i32[] [10105, 10157, 10205], "Value"=w1603, "Name"=w1609) -> ("output cluster"=w1608:T1)  [unwired: 3 in]
    }
    frame "Counter Input:Frequency:Measurement Specifications:High Frequency:Measurement Time" {
      n322 = property class="DAQmx Channel"(reference=w1611, error in=w1617, "ActiveChans"=w1612) -> (reference out=w1620:refnum<k21>, error out=w1616:errorcluster, "CI.Freq.MeasTime"=w1613:dbl)
      n323 = call-poly <vilib>:"ex_setTdmProperty.vi"("Strings"=string[] [], "Values"=i32[] [], "Value"=w1613, "Name"=w1619) -> ("output cluster"=w1618:T1)  [unwired: 3 in]
    }
    frame "Counter Input:Frequency:Measurement Specifications:Large Range:Divisor" {
      n324 = property class="DAQmx Channel"(reference=w1621, error in=w1627, "ActiveChans"=w1622) -> (reference out=w1630:refnum<k21>, error out=w1626:errorcluster, "CI.Freq.Div"=w1623:u32)
      n325 = call-poly <vilib>:"ex_setTdmProperty.vi"("Strings"=string[] [], "Values"=i32[] [], "Value"=w1623, "Name"=w1629) -> ("output cluster"=w1628:T1)  [unwired: 3 in]
    }
    frame "Counter Input:Frequency:Digital Filter:Enable" {
      n326 = property class="DAQmx Channel"(reference=w1631, error in=w1637, "ActiveChans"=w1632) -> (reference out=w1640:refnum<k21>, error out=w1636:errorcluster, "CI.Freq.DigFltr.Enable"=w1633:bool)
      n327 = call-poly <vilib>:"ex_setTdmProperty.vi"("Strings"=string[] [], "Values"=i32[] [], "Value"=w1633, "Name"=w1639) -> ("output cluster"=w1638:T1)  [unwired: 3 in]
    }
    frame "Counter Input:Frequency:Digital Filter:Minimum Pulse Width" {
      n328 = property class="DAQmx Channel"(reference=w1641, error in=w1647, "ActiveChans"=w1642) -> (reference out=w1650:refnum<k21>, error out=w1646:errorcluster, "CI.Freq.DigFltr.MinPulseWidth"=w1643:dbl)
      n329 = call-poly <vilib>:"ex_setTdmProperty.vi"("Strings"=string[] [], "Values"=i32[] [], "Value"=w1643, "Name"=w1649) -> ("output cluster"=w1648:T1)  [unwired: 3 in]
    }
    frame "Counter Input:Frequency:Digital Filter:Timebase:Source" {
      n330 = property class="DAQmx Channel"(reference=w1651, error in=w1657, "ActiveChans"=w1652) -> (reference out=w1660:refnum<k21>, error out=w1656:errorcluster, "CI.Freq.DigFltr.TimebaseSrc"=w1653:tag)
      n331 = call-poly <vilib>:"ex_setTdmProperty.vi"("Strings"=string[] [], "Values"=i32[] [], "Value"=w1653, "Name"=w1659) -> ("output cluster"=w1658:T1)  [unwired: 3 in]
    }
    frame "Counter Input:Frequency:Digital Filter:Timebase:Rate" {
      n332 = property class="DAQmx Channel"(reference=w1661, error in=w1667, "ActiveChans"=w1662) -> (reference out=w1670:refnum<k21>, error out=w1666:errorcluster, "CI.Freq.DigFltr.TimebaseRate"=w1663:dbl)
      n333 = call-poly <vilib>:"ex_setTdmProperty.vi"("Strings"=string[] [], "Values"=i32[] [], "Value"=w1663, "Name"=w1669) -> ("output cluster"=w1668:T1)  [unwired: 3 in]
    }
    frame "Counter Input:Frequency:Digital Synchronization:Enable" {
      n334 = property class="DAQmx Channel"(reference=w1671, error in=w1677, "ActiveChans"=w1672) -> (reference out=w1680:refnum<k21>, error out=w1676:errorcluster, "CI.Freq.DigSync.Enable"=w1673:bool)
      n335 = call-poly <vilib>:"ex_setTdmProperty.vi"("Strings"=string[] [], "Values"=i32[] [], "Value"=w1673, "Name"=w1679) -> ("output cluster"=w1678:T1)  [unwired: 3 in]
    }
    frame "Counter Input:Period:Units" {
      n336 = property class="DAQmx Channel"(reference=w1681, error in=w1687, "ActiveChans"=w1682) -> (reference out=w1690:refnum<k21>, error out=w1686:errorcluster, "CI.Period.Units"=w1683:i32)
      n337 = call-poly <vilib>:"ex_setTdmProperty.vi"("Strings"=string[] ["Seconds", "Ticks", "From Custom Scale"], "Values"=i32[] [10364, 10304, 10065], "Value"=w1683, "Name"=w1689) -> ("output cluster"=w1688:T1)  [unwired: 3 in]
    }
    frame "Counter Input:Period:Input Terminal" {
      n338 = property class="DAQmx Channel"(reference=w1691, error in=w1697, "ActiveChans"=w1692) -> (reference out=w1700:refnum<k21>, error out=w1696:errorcluster, "CI.Period.Term"=w1693:tag)
      n339 = call-poly <vilib>:"ex_setTdmProperty.vi"("Strings"=string[] [], "Values"=i32[] [], "Value"=w1693, "Name"=w1699) -> ("output cluster"=w1698:T1)  [unwired: 3 in]
    }
    frame "Counter Input:Period:Starting Edge" {
      n340 = property class="DAQmx Channel"(reference=w1701, error in=w1707, "ActiveChans"=w1702) -> (reference out=w1710:refnum<k21>, error out=w1706:errorcluster, "CI.Period.StartingEdge"=w1703:i32)
      n341 = call-poly <vilib>:"ex_setTdmProperty.vi"("Strings"=string[] ["Rising", "Falling"], "Values"=i32[] [10280, 10171], "Value"=w1703, "Name"=w1709) -> ("output cluster"=w1708:T1)  [unwired: 3 in]
    }
    frame "Counter Input:Period:Measurement Specifications:Method" {
      n342 = property class="DAQmx Channel"(reference=w1711, error in=w1717, "ActiveChans"=w1712) -> (reference out=w1720:refnum<k21>, error out=w1716:errorcluster, "CI.Period.MeasMeth"=w1713:i32)
      n343 = call-poly <vilib>:"ex_setTdmProperty.vi"("Strings"=string[] ["Low Frequency with 1 Counter", "High Frequency with 2 Counters", "Large Range with 2 Counters"], "Values"=i32[] [10105, 10157, 10205], "Value"=w1713, "Name"=w1719) -> ("output cluster"=w1718:T1)  [unwired: 3 in]
    }
    frame "Counter Input:Period:Measurement Specifications:High Frequency:Measurement Time" {
      n344 = property class="DAQmx Channel"(reference=w1721, error in=w1727, "ActiveChans"=w1722) -> (reference out=w1730:refnum<k21>, error out=w1726:errorcluster, "CI.Period.MeasTime"=w1723:dbl)
      n345 = call-poly <vilib>:"ex_setTdmProperty.vi"("Strings"=string[] [], "Values"=i32[] [], "Value"=w1723, "Name"=w1729) -> ("output cluster"=w1728:T1)  [unwired: 3 in]
    }
    frame "Counter Input:Period:Measurement Specifications:Large Range:Divisor" {
      n346 = property class="DAQmx Channel"(reference=w1731, error in=w1737, "ActiveChans"=w1732) -> (reference out=w1740:refnum<k21>, error out=w1736:errorcluster, "CI.Period.Div"=w1733:u32)
      n347 = call-poly <vilib>:"ex_setTdmProperty.vi"("Strings"=string[] [], "Values"=i32[] [], "Value"=w1733, "Name"=w1739) -> ("output cluster"=w1738:T1)  [unwired: 3 in]
    }
    frame "Counter Input:Period:Digital Filter:Enable" {
      n348 = property class="DAQmx Channel"(reference=w1741, error in=w1747, "ActiveChans"=w1742) -> (reference out=w1750:refnum<k21>, error out=w1746:errorcluster, "CI.Period.DigFltr.Enable"=w1743:bool)
      n349 = call-poly <vilib>:"ex_setTdmProperty.vi"("Strings"=string[] [], "Values"=i32[] [], "Value"=w1743, "Name"=w1749) -> ("output cluster"=w1748:T1)  [unwired: 3 in]
    }
    frame "Counter Input:Period:Digital Filter:Minimum Pulse Width" {
      n350 = property class="DAQmx Channel"(reference=w1751, error in=w1757, "ActiveChans"=w1752) -> (reference out=w1760:refnum<k21>, error out=w1756:errorcluster, "CI.Period.DigFltr.MinPulseWidth"=w1753:dbl)
      n351 = call-poly <vilib>:"ex_setTdmProperty.vi"("Strings"=string[] [], "Values"=i32[] [], "Value"=w1753, "Name"=w1759) -> ("output cluster"=w1758:T1)  [unwired: 3 in]
    }
    frame "Counter Input:Period:Digital Filter:Timebase:Source" {
      n352 = property class="DAQmx Channel"(reference=w1761, error in=w1767, "ActiveChans"=w1762) -> (reference out=w1770:refnum<k21>, error out=w1766:errorcluster, "CI.Period.DigFltr.TimebaseSrc"=w1763:tag)
      n353 = call-poly <vilib>:"ex_setTdmProperty.vi"("Strings"=string[] [], "Values"=i32[] [], "Value"=w1763, "Name"=w1769) -> ("output cluster"=w1768:T1)  [unwired: 3 in]
    }
    frame "Counter Input:Period:Digital Filter:Timebase:Rate" {
      n354 = property class="DAQmx Channel"(reference=w1771, error in=w1777, "ActiveChans"=w1772) -> (reference out=w1780:refnum<k21>, error out=w1776:errorcluster, "CI.Period.DigFltr.TimebaseRate"=w1773:dbl)
      n355 = call-poly <vilib>:"ex_setTdmProperty.vi"("Strings"=string[] [], "Values"=i32[] [], "Value"=w1773, "Name"=w1779) -> ("output cluster"=w1778:T1)  [unwired: 3 in]
    }
    frame "Counter Input:Period:Digital Synchronization:Enable" {
      n356 = property class="DAQmx Channel"(reference=w1781, error in=w1787, "ActiveChans"=w1782) -> (reference out=w1790:refnum<k21>, error out=w1786:errorcluster, "CI.Period.DigSync.Enable"=w1783:bool)
      n357 = call-poly <vilib>:"ex_setTdmProperty.vi"("Strings"=string[] [], "Values"=i32[] [], "Value"=w1783, "Name"=w1789) -> ("output cluster"=w1788:T1)  [unwired: 3 in]
    }
    frame "Counter Input:Count Edges:Input Terminal" {
      n358 = property class="DAQmx Channel"(reference=w1791, error in=w1797, "ActiveChans"=w1792) -> (reference out=w1800:refnum<k21>, error out=w1796:errorcluster, "CI.CountEdges.Term"=w1793:tag)
      n359 = call-poly <vilib>:"ex_setTdmProperty.vi"("Strings"=string[] [], "Values"=i32[] [], "Value"=w1793, "Name"=w1799) -> ("output cluster"=w1798:T1)  [unwired: 3 in]
    }
    frame "Counter Input:Count Edges:Count Direction:Direction" {
      n360 = property class="DAQmx Channel"(reference=w1801, error in=w1807, "ActiveChans"=w1802) -> (reference out=w1810:refnum<k21>, error out=w1806:errorcluster, "CI.CountEdges.Dir"=w1803:i32)
      n361 = call-poly <vilib>:"ex_setTdmProperty.vi"("Strings"=string[] ["Count Up", "Count Down", "Externally Controlled"], "Values"=i32[] [10128, 10124, 10326], "Value"=w1803, "Name"=w1809) -> ("output cluster"=w1808:T1)  [unwired: 3 in]
    }
    frame "Counter Input:Count Edges:Count Direction:Terminal" {
      n362 = property class="DAQmx Channel"(reference=w1811, error in=w1817, "ActiveChans"=w1812) -> (reference out=w1820:refnum<k21>, error out=w1816:errorcluster, "CI.CountEdges.DirTerm"=w1813:tag)
      n363 = call-poly <vilib>:"ex_setTdmProperty.vi"("Strings"=string[] [], "Values"=i32[] [], "Value"=w1813, "Name"=w1819) -> ("output cluster"=w1818:T1)  [unwired: 3 in]
    }
    frame "Counter Input:Count Edges:Count Direction:Digital Filter:Enable" {
      n364 = property class="DAQmx Channel"(reference=w1821, error in=w1827, "ActiveChans"=w1822) -> (reference out=w1830:refnum<k21>, error out=w1826:errorcluster, "CI.CountEdges.CountDir.DigFltr.Enable"=w1823:bool)
      n365 = call-poly <vilib>:"ex_setTdmProperty.vi"("Strings"=string[] [], "Values"=i32[] [], "Value"=w1823, "Name"=w1829) -> ("output cluster"=w1828:T1)  [unwired: 3 in]
    }
    frame "Counter Input:Count Edges:Count Direction:Digital Filter:Minimum Pulse Width" {
      n366 = property class="DAQmx Channel"(reference=w1831, error in=w1837, "ActiveChans"=w1832) -> (reference out=w1840:refnum<k21>, error out=w1836:errorcluster, "CI.CountEdges.CountDir.DigFltr.MinPulseWidth"=w1833:dbl)
      n367 = call-poly <vilib>:"ex_setTdmProperty.vi"("Strings"=string[] [], "Values"=i32[] [], "Value"=w1833, "Name"=w1839) -> ("output cluster"=w1838:T1)  [unwired: 3 in]
    }
    frame "Counter Input:Count Edges:Count Direction:Digital Filter:Timebase:Source" {
      n368 = property class="DAQmx Channel"(reference=w1841, error in=w1847, "ActiveChans"=w1842) -> (reference out=w1850:refnum<k21>, error out=w1846:errorcluster, "CI.CountEdges.CountDir.DigFltr.TimebaseSrc"=w1843:tag)
      n369 = call-poly <vilib>:"ex_setTdmProperty.vi"("Strings"=string[] [], "Values"=i32[] [], "Value"=w1843, "Name"=w1849) -> ("output cluster"=w1848:T1)  [unwired: 3 in]
    }
    frame "Counter Input:Count Edges:Count Direction:Digital Filter:Timebase:Rate" {
      n370 = property class="DAQmx Channel"(reference=w1851, error in=w1857, "ActiveChans"=w1852) -> (reference out=w1860:refnum<k21>, error out=w1856:errorcluster, "CI.CountEdges.CountDir.DigFltr.TimebaseRate"=w1853:dbl)
      n371 = call-poly <vilib>:"ex_setTdmProperty.vi"("Strings"=string[] [], "Values"=i32[] [], "Value"=w1853, "Name"=w1859) -> ("output cluster"=w1858:T1)  [unwired: 3 in]
    }
    frame "Counter Input:Count Edges:Count Direction:Digital Synchronization:Enable" {
      n372 = property class="DAQmx Channel"(reference=w1861, error in=w1867, "ActiveChans"=w1862) -> (reference out=w1870:refnum<k21>, error out=w1866:errorcluster, "CI.CountEdges.CountDir.DigSync.Enable"=w1863:bool)
      n373 = call-poly <vilib>:"ex_setTdmProperty.vi"("Strings"=string[] [], "Values"=i32[] [], "Value"=w1863, "Name"=w1869) -> ("output cluster"=w1868:T1)  [unwired: 3 in]
    }
    frame "Counter Input:Count Edges:Initial Count" {
      n374 = property class="DAQmx Channel"(reference=w1871, error in=w1877, "ActiveChans"=w1872) -> (reference out=w1880:refnum<k21>, error out=w1876:errorcluster, "CI.CountEdges.InitialCnt"=w1873:u32)
      n375 = call-poly <vilib>:"ex_setTdmProperty.vi"("Strings"=string[] [], "Values"=i32[] [], "Value"=w1873, "Name"=w1879) -> ("output cluster"=w1878:T1)  [unwired: 3 in]
    }
    frame "Counter Input:Count Edges:Active Edge" {
      n376 = property class="DAQmx Channel"(reference=w1881, error in=w1887, "ActiveChans"=w1882) -> (reference out=w1890:refnum<k21>, error out=w1886:errorcluster, "CI.CountEdges.ActiveEdge"=w1883:i32)
      n377 = call-poly <vilib>:"ex_setTdmProperty.vi"("Strings"=string[] ["Rising", "Falling"], "Values"=i32[] [10280, 10171], "Value"=w1883, "Name"=w1889) -> ("output cluster"=w1888:T1)  [unwired: 3 in]
    }
    frame "Counter Input:Count Edges:Digital Filter:Enable" {
      n378 = property class="DAQmx Channel"(reference=w1891, error in=w1897, "ActiveChans"=w1892) -> (reference out=w1900:refnum<k21>, error out=w1896:errorcluster, "CI.CountEdges.DigFltr.Enable"=w1893:bool)
      n379 = call-poly <vilib>:"ex_setTdmProperty.vi"("Strings"=string[] [], "Values"=i32[] [], "Value"=w1893, "Name"=w1899) -> ("output cluster"=w1898:T1)  [unwired: 3 in]
    }
    frame "Counter Input:Count Edges:Digital Filter:Minimum Pulse Width" {
      n380 = property class="DAQmx Channel"(reference=w1901, error in=w1907, "ActiveChans"=w1902) -> (reference out=w1910:refnum<k21>, error out=w1906:errorcluster, "CI.CountEdges.DigFltr.MinPulseWidth"=w1903:dbl)
      n381 = call-poly <vilib>:"ex_setTdmProperty.vi"("Strings"=string[] [], "Values"=i32[] [], "Value"=w1903, "Name"=w1909) -> ("output cluster"=w1908:T1)  [unwired: 3 in]
    }
    frame "Counter Input:Count Edges:Digital Filter:Timebase:Source" {
      n382 = property class="DAQmx Channel"(reference=w1911, error in=w1917, "ActiveChans"=w1912) -> (reference out=w1920:refnum<k21>, error out=w1916:errorcluster, "CI.CountEdges.DigFltr.TimebaseSrc"=w1913:tag)
      n383 = call-poly <vilib>:"ex_setTdmProperty.vi"("Strings"=string[] [], "Values"=i32[] [], "Value"=w1913, "Name"=w1919) -> ("output cluster"=w1918:T1)  [unwired: 3 in]
    }
    frame "Counter Input:Count Edges:Digital Filter:Timebase:Rate" {
      n384 = property class="DAQmx Channel"(reference=w1921, error in=w1927, "ActiveChans"=w1922) -> (reference out=w1930:refnum<k21>, error out=w1926:errorcluster, "CI.CountEdges.DigFltr.TimebaseRate"=w1923:dbl)
      n385 = call-poly <vilib>:"ex_setTdmProperty.vi"("Strings"=string[] [], "Values"=i32[] [], "Value"=w1923, "Name"=w1929) -> ("output cluster"=w1928:T1)  [unwired: 3 in]
    }
    frame "Counter Input:Count Edges:Digital Synchronization:Enable" {
      n386 = property class="DAQmx Channel"(reference=w1931, error in=w1937, "ActiveChans"=w1932) -> (reference out=w1940:refnum<k21>, error out=w1936:errorcluster, "CI.CountEdges.DigSync.Enable"=w1933:bool)
      n387 = call-poly <vilib>:"ex_setTdmProperty.vi"("Strings"=string[] [], "Values"=i32[] [], "Value"=w1933, "Name"=w1939) -> ("output cluster"=w1938:T1)  [unwired: 3 in]
    }
    frame "Counter Input:Position:Angular Encoder:Units" {
      n388 = property class="DAQmx Channel"(reference=w1941, error in=w1947, "ActiveChans"=w1942) -> (reference out=w1950:refnum<k21>, error out=w1946:errorcluster, "CI.AngEncoder.Units"=w1943:i32)
      n389 = call-poly <vilib>:"ex_setTdmProperty.vi"("Strings"=string[] ["Degrees", "Radians", "Ticks", "From Custom Scale"], "Values"=i32[] [10146, 10273, 10304, 10065], "Value"=w1943, "Name"=w1949) -> ("output cluster"=w1948:T1)  [unwired: 3 in]
    }
    frame "Counter Input:Position:Angular Encoder:Pulses Per Revolution" {
      n390 = property class="DAQmx Channel"(reference=w1951, error in=w1957, "ActiveChans"=w1952) -> (reference out=w1960:refnum<k21>, error out=w1956:errorcluster, "CI.AngEncoder.PulsesPerRev"=w1953:u32)
      n391 = call-poly <vilib>:"ex_setTdmProperty.vi"("Strings"=string[] [], "Values"=i32[] [], "Value"=w1953, "Name"=w1959) -> ("output cluster"=w1958:T1)  [unwired: 3 in]
    }
    frame "Counter Input:Position:Angular Encoder:Initial Angle" {
      n392 = property class="DAQmx Channel"(reference=w1961, error in=w1967, "ActiveChans"=w1962) -> (reference out=w1970:refnum<k21>, error out=w1966:errorcluster, "CI.AngEncoder.InitialAngle"=w1963:dbl)
      n393 = call-poly <vilib>:"ex_setTdmProperty.vi"("Strings"=string[] [], "Values"=i32[] [], "Value"=w1963, "Name"=w1969) -> ("output cluster"=w1968:T1)  [unwired: 3 in]
    }
    frame "Counter Input:Position:Linear Encoder:Units" {
      n394 = property class="DAQmx Channel"(reference=w1971, error in=w1977, "ActiveChans"=w1972) -> (reference out=w1980:refnum<k21>, error out=w1976:errorcluster, "CI.LinEncoder.Units"=w1973:i32)
      n395 = call-poly <vilib>:"ex_setTdmProperty.vi"("Strings"=string[] ["Meters", "Inches", "Ticks", "From Custom Scale"], "Values"=i32[] [10219, 10379, 10304, 10065], "Value"=w1973, "Name"=w1979) -> ("output cluster"=w1978:T1)  [unwired: 3 in]
    }
    frame "Counter Input:Position:Linear Encoder:Distance Per Pulse" {
      n396 = property class="DAQmx Channel"(reference=w1981, error in=w1987, "ActiveChans"=w1982) -> (reference out=w1990:refnum<k21>, error out=w1986:errorcluster, "CI.LinEncoder.DistPerPulse"=w1983:dbl)
      n397 = call-poly <vilib>:"ex_setTdmProperty.vi"("Strings"=string[] [], "Values"=i32[] [], "Value"=w1983, "Name"=w1989) -> ("output cluster"=w1988:T1)  [unwired: 3 in]
    }
    frame "Counter Input:Position:Linear Encoder:Initial Position" {
      n398 = property class="DAQmx Channel"(reference=w1991, error in=w1997, "ActiveChans"=w1992) -> (reference out=w2000:refnum<k21>, error out=w1996:errorcluster, "CI.LinEncoder.InitialPos"=w1993:dbl)
      n399 = call-poly <vilib>:"ex_setTdmProperty.vi"("Strings"=string[] [], "Values"=i32[] [], "Value"=w1993, "Name"=w1999) -> ("output cluster"=w1998:T1)  [unwired: 3 in]
    }
    frame "Counter Input:Position:Decoding Type" {
      n400 = property class="DAQmx Channel"(reference=w2001, error in=w2007, "ActiveChans"=w2002) -> (reference out=w2010:refnum<k21>, error out=w2006:errorcluster, "CI.Encoder.DecodingType"=w2003:i32)
      n401 = call-poly <vilib>:"ex_setTdmProperty.vi"("Strings"=string[] ["X1", "X2", "X4", "Two Pulse Counting"], "Values"=i32[] [10090, 10091, 10092, 10313], "Value"=w2003, "Name"=w2009) -> ("output cluster"=w2008:T1)  [unwired: 3 in]
    }
    frame "Counter Input:Position:A Input:Terminal" {
      n402 = property class="DAQmx Channel"(reference=w2011, error in=w2017, "ActiveChans"=w2012) -> (reference out=w2020:refnum<k21>, error out=w2016:errorcluster, "CI.Encoder.AInputTerm"=w2013:tag)
      n403 = call-poly <vilib>:"ex_setTdmProperty.vi"("Strings"=string[] [], "Values"=i32[] [], "Value"=w2013, "Name"=w2019) -> ("output cluster"=w2018:T1)  [unwired: 3 in]
    }
    frame "Counter Input:Position:A Input:Digital Filter:Enable" {
      n404 = property class="DAQmx Channel"(reference=w2021, error in=w2027, "ActiveChans"=w2022) -> (reference out=w2030:refnum<k21>, error out=w2026:errorcluster, "CI.Encoder.AInput.DigFltr.Enable"=w2023:bool)
      n405 = call-poly <vilib>:"ex_setTdmProperty.vi"("Strings"=string[] [], "Values"=i32[] [], "Value"=w2023, "Name"=w2029) -> ("output cluster"=w2028:T1)  [unwired: 3 in]
    }
    frame "Counter Input:Position:A Input:Digital Filter:Minimum Pulse Width" {
      n406 = property class="DAQmx Channel"(reference=w2031, error in=w2037, "ActiveChans"=w2032) -> (reference out=w2040:refnum<k21>, error out=w2036:errorcluster, "CI.Encoder.AInput.DigFltr.MinPulseWidth"=w2033:dbl)
      n407 = call-poly <vilib>:"ex_setTdmProperty.vi"("Strings"=string[] [], "Values"=i32[] [], "Value"=w2033, "Name"=w2039) -> ("output cluster"=w2038:T1)  [unwired: 3 in]
    }
    frame "Counter Input:Position:A Input:Digital Filter:Timebase:Source" {
      n408 = property class="DAQmx Channel"(reference=w2041, error in=w2047, "ActiveChans"=w2042) -> (reference out=w2050:refnum<k21>, error out=w2046:errorcluster, "CI.Encoder.AInput.DigFltr.TimebaseSrc"=w2043:tag)
      n409 = call-poly <vilib>:"ex_setTdmProperty.vi"("Strings"=string[] [], "Values"=i32[] [], "Value"=w2043, "Name"=w2049) -> ("output cluster"=w2048:T1)  [unwired: 3 in]
    }
    frame "Counter Input:Position:A Input:Digital Filter:Timebase:Rate" {
      n410 = property class="DAQmx Channel"(reference=w2051, error in=w2057, "ActiveChans"=w2052) -> (reference out=w2060:refnum<k21>, error out=w2056:errorcluster, "CI.Encoder.AInput.DigFltr.TimebaseRate"=w2053:dbl)
      n411 = call-poly <vilib>:"ex_setTdmProperty.vi"("Strings"=string[] [], "Values"=i32[] [], "Value"=w2053, "Name"=w2059) -> ("output cluster"=w2058:T1)  [unwired: 3 in]
    }
    frame "Counter Input:Position:A Input:Digital Synchronization:Enable" {
      n412 = property class="DAQmx Channel"(reference=w2061, error in=w2067, "ActiveChans"=w2062) -> (reference out=w2070:refnum<k21>, error out=w2066:errorcluster, "CI.Encoder.AInput.DigSync.Enable"=w2063:bool)
      n413 = call-poly <vilib>:"ex_setTdmProperty.vi"("Strings"=string[] [], "Values"=i32[] [], "Value"=w2063, "Name"=w2069) -> ("output cluster"=w2068:T1)  [unwired: 3 in]
    }
    frame "Counter Input:Position:B Input:Terminal" {
      n414 = property class="DAQmx Channel"(reference=w2071, error in=w2077, "ActiveChans"=w2072) -> (reference out=w2080:refnum<k21>, error out=w2076:errorcluster, "CI.Encoder.BInputTerm"=w2073:tag)
      n415 = call-poly <vilib>:"ex_setTdmProperty.vi"("Strings"=string[] [], "Values"=i32[] [], "Value"=w2073, "Name"=w2079) -> ("output cluster"=w2078:T1)  [unwired: 3 in]
    }
    frame "Counter Input:Position:B Input:Digital Filter:Enable" {
      n416 = property class="DAQmx Channel"(reference=w2081, error in=w2087, "ActiveChans"=w2082) -> (reference out=w2090:refnum<k21>, error out=w2086:errorcluster, "CI.Encoder.BInput.DigFltr.Enable"=w2083:bool)
      n417 = call-poly <vilib>:"ex_setTdmProperty.vi"("Strings"=string[] [], "Values"=i32[] [], "Value"=w2083, "Name"=w2089) -> ("output cluster"=w2088:T1)  [unwired: 3 in]
    }
    frame "Counter Input:Position:B Input:Digital Filter:Minimum Pulse Width" {
      n418 = property class="DAQmx Channel"(reference=w2091, error in=w2097, "ActiveChans"=w2092) -> (reference out=w2100:refnum<k21>, error out=w2096:errorcluster, "CI.Encoder.BInput.DigFltr.MinPulseWidth"=w2093:dbl)
      n419 = call-poly <vilib>:"ex_setTdmProperty.vi"("Strings"=string[] [], "Values"=i32[] [], "Value"=w2093, "Name"=w2099) -> ("output cluster"=w2098:T1)  [unwired: 3 in]
    }
    frame "Counter Input:Position:B Input:Digital Filter:Timebase:Source" {
      n420 = property class="DAQmx Channel"(reference=w2101, error in=w2107, "ActiveChans"=w2102) -> (reference out=w2110:refnum<k21>, error out=w2106:errorcluster, "CI.Encoder.BInput.DigFltr.TimebaseSrc"=w2103:tag)
      n421 = call-poly <vilib>:"ex_setTdmProperty.vi"("Strings"=string[] [], "Values"=i32[] [], "Value"=w2103, "Name"=w2109) -> ("output cluster"=w2108:T1)  [unwired: 3 in]
    }
    frame "Counter Input:Position:B Input:Digital Filter:Timebase:Rate" {
      n422 = property class="DAQmx Channel"(reference=w2111, error in=w2117, "ActiveChans"=w2112) -> (reference out=w2120:refnum<k21>, error out=w2116:errorcluster, "CI.Encoder.BInput.DigFltr.TimebaseRate"=w2113:dbl)
      n423 = call-poly <vilib>:"ex_setTdmProperty.vi"("Strings"=string[] [], "Values"=i32[] [], "Value"=w2113, "Name"=w2119) -> ("output cluster"=w2118:T1)  [unwired: 3 in]
    }
    frame "Counter Input:Position:B Input:Digital Synchronization:Enable" {
      n424 = property class="DAQmx Channel"(reference=w2121, error in=w2127, "ActiveChans"=w2122) -> (reference out=w2130:refnum<k21>, error out=w2126:errorcluster, "CI.Encoder.BInput.DigSync.Enable"=w2123:bool)
      n425 = call-poly <vilib>:"ex_setTdmProperty.vi"("Strings"=string[] [], "Values"=i32[] [], "Value"=w2123, "Name"=w2129) -> ("output cluster"=w2128:T1)  [unwired: 3 in]
    }
    frame "Counter Input:Position:Z Input:Terminal" {
      n426 = property class="DAQmx Channel"(reference=w2131, error in=w2137, "ActiveChans"=w2132) -> (reference out=w2140:refnum<k21>, error out=w2136:errorcluster, "CI.Encoder.ZInputTerm"=w2133:tag)
      n427 = call-poly <vilib>:"ex_setTdmProperty.vi"("Strings"=string[] [], "Values"=i32[] [], "Value"=w2133, "Name"=w2139) -> ("output cluster"=w2138:T1)  [unwired: 3 in]
    }
    frame "Counter Input:Position:Z Input:Digital Filter:Enable" {
      n428 = property class="DAQmx Channel"(reference=w2141, error in=w2147, "ActiveChans"=w2142) -> (reference out=w2150:refnum<k21>, error out=w2146:errorcluster, "CI.Encoder.ZInput.DigFltr.Enable"=w2143:bool)
      n429 = call-poly <vilib>:"ex_setTdmProperty.vi"("Strings"=string[] [], "Values"=i32[] [], "Value"=w2143, "Name"=w2149) -> ("output cluster"=w2148:T1)  [unwired: 3 in]
    }
    frame "Counter Input:Position:Z Input:Digital Filter:Minimum Pulse Width" {
      n430 = property class="DAQmx Channel"(reference=w2151, error in=w2157, "ActiveChans"=w2152) -> (reference out=w2160:refnum<k21>, error out=w2156:errorcluster, "CI.Encoder.ZInput.DigFltr.MinPulseWidth"=w2153:dbl)
      n431 = call-poly <vilib>:"ex_setTdmProperty.vi"("Strings"=string[] [], "Values"=i32[] [], "Value"=w2153, "Name"=w2159) -> ("output cluster"=w2158:T1)  [unwired: 3 in]
    }
    frame "Counter Input:Position:Z Input:Digital Filter:Timebase:Source" {
      n432 = property class="DAQmx Channel"(reference=w2161, error in=w2167, "ActiveChans"=w2162) -> (reference out=w2170:refnum<k21>, error out=w2166:errorcluster, "CI.Encoder.ZInput.DigFltr.TimebaseSrc"=w2163:tag)
      n433 = call-poly <vilib>:"ex_setTdmProperty.vi"("Strings"=string[] [], "Values"=i32[] [], "Value"=w2163, "Name"=w2169) -> ("output cluster"=w2168:T1)  [unwired: 3 in]
    }
    frame "Counter Input:Position:Z Input:Digital Filter:Timebase:Rate" {
      n434 = property class="DAQmx Channel"(reference=w2171, error in=w2177, "ActiveChans"=w2172) -> (reference out=w2180:refnum<k21>, error out=w2176:errorcluster, "CI.Encoder.ZInput.DigFltr.TimebaseRate"=w2173:dbl)
      n435 = call-poly <vilib>:"ex_setTdmProperty.vi"("Strings"=string[] [], "Values"=i32[] [], "Value"=w2173, "Name"=w2179) -> ("output cluster"=w2178:T1)  [unwired: 3 in]
    }
    frame "Counter Input:Position:Z Input:Digital Synchronization:Enable" {
      n436 = property class="DAQmx Channel"(reference=w2181, error in=w2187, "ActiveChans"=w2182) -> (reference out=w2190:refnum<k21>, error out=w2186:errorcluster, "CI.Encoder.ZInput.DigSync.Enable"=w2183:bool)
      n437 = call-poly <vilib>:"ex_setTdmProperty.vi"("Strings"=string[] [], "Values"=i32[] [], "Value"=w2183, "Name"=w2189) -> ("output cluster"=w2188:T1)  [unwired: 3 in]
    }
    frame "Counter Input:Position:Z Index Enable" {
      n438 = property class="DAQmx Channel"(reference=w2191, error in=w2197, "ActiveChans"=w2192) -> (reference out=w2200:refnum<k21>, error out=w2196:errorcluster, "CI.Encoder.ZIndexEnable"=w2193:bool)
      n439 = call-poly <vilib>:"ex_setTdmProperty.vi"("Strings"=string[] [], "Values"=i32[] [], "Value"=w2193, "Name"=w2199) -> ("output cluster"=w2198:T1)  [unwired: 3 in]
    }
    frame "Counter Input:Position:Z Index Value" {
      n440 = property class="DAQmx Channel"(reference=w2201, error in=w2207, "ActiveChans"=w2202) -> (reference out=w2210:refnum<k21>, error out=w2206:errorcluster, "CI.Encoder.ZIndexVal"=w2203:dbl)
      n441 = call-poly <vilib>:"ex_setTdmProperty.vi"("Strings"=string[] [], "Values"=i32[] [], "Value"=w2203, "Name"=w2209) -> ("output cluster"=w2208:T1)  [unwired: 3 in]
    }
    frame "Counter Input:Position:Z Index Phase" {
      n442 = property class="DAQmx Channel"(reference=w2211, error in=w2217, "ActiveChans"=w2212) -> (reference out=w2220:refnum<k21>, error out=w2216:errorcluster, "CI.Encoder.ZIndexPhase"=w2213:i32)
      n443 = call-poly <vilib>:"ex_setTdmProperty.vi"("Strings"=string[] ["A High B High", "A High B Low", "A Low B High", "A Low B Low"], "Values"=i32[] [10040, 10041, 10042, 10043], "Value"=w2213, "Name"=w2219) -> ("output cluster"=w2218:T1)  [unwired: 3 in]
    }
    frame "Counter Input:Pulse Width:Units" {
      n444 = property class="DAQmx Channel"(reference=w2221, error in=w2227, "ActiveChans"=w2222) -> (reference out=w2230:refnum<k21>, error out=w2226:errorcluster, "CI.PulseWidth.Units"=w2223:i32)
      n445 = call-poly <vilib>:"ex_setTdmProperty.vi"("Strings"=string[] ["Seconds", "Ticks", "From Custom Scale"], "Values"=i32[] [10364, 10304, 10065], "Value"=w2223, "Name"=w2229) -> ("output cluster"=w2228:T1)  [unwired: 3 in]
    }
    frame "Counter Input:Pulse Width:Input Terminal" {
      n446 = property class="DAQmx Channel"(reference=w2231, error in=w2237, "ActiveChans"=w2232) -> (reference out=w2240:refnum<k21>, error out=w2236:errorcluster, "CI.PulseWidth.Term"=w2233:tag)
      n447 = call-poly <vilib>:"ex_setTdmProperty.vi"("Strings"=string[] [], "Values"=i32[] [], "Value"=w2233, "Name"=w2239) -> ("output cluster"=w2238:T1)  [unwired: 3 in]
    }
    frame "Counter Input:Pulse Width:Starting Edge" {
      n448 = property class="DAQmx Channel"(reference=w2241, error in=w2247, "ActiveChans"=w2242) -> (reference out=w2250:refnum<k21>, error out=w2246:errorcluster, "CI.PulseWidth.StartingEdge"=w2243:i32)
      n449 = call-poly <vilib>:"ex_setTdmProperty.vi"("Strings"=string[] ["Rising", "Falling"], "Values"=i32[] [10280, 10171], "Value"=w2243, "Name"=w2249) -> ("output cluster"=w2248:T1)  [unwired: 3 in]
    }
    frame "Counter Input:Pulse Width:Digital Filter:Enable" {
      n450 = property class="DAQmx Channel"(reference=w2251, error in=w2257, "ActiveChans"=w2252) -> (reference out=w2260:refnum<k21>, error out=w2256:errorcluster, "CI.PulseWidth.DigFltr.Enable"=w2253:bool)
      n451 = call-poly <vilib>:"ex_setTdmProperty.vi"("Strings"=string[] [], "Values"=i32[] [], "Value"=w2253, "Name"=w2259) -> ("output cluster"=w2258:T1)  [unwired: 3 in]
    }
    frame "Counter Input:Pulse Width:Digital Filter:Minimum Pulse Width" {
      n452 = property class="DAQmx Channel"(reference=w2261, error in=w2267, "ActiveChans"=w2262) -> (reference out=w2270:refnum<k21>, error out=w2266:errorcluster, "CI.PulseWidth.DigFltr.MinPulseWidth"=w2263:dbl)
      n453 = call-poly <vilib>:"ex_setTdmProperty.vi"("Strings"=string[] [], "Values"=i32[] [], "Value"=w2263, "Name"=w2269) -> ("output cluster"=w2268:T1)  [unwired: 3 in]
    }
    frame "Counter Input:Pulse Width:Digital Filter:Timebase:Source" {
      n454 = property class="DAQmx Channel"(reference=w2271, error in=w2277, "ActiveChans"=w2272) -> (reference out=w2280:refnum<k21>, error out=w2276:errorcluster, "CI.PulseWidth.DigFltr.TimebaseSrc"=w2273:tag)
      n455 = call-poly <vilib>:"ex_setTdmProperty.vi"("Strings"=string[] [], "Values"=i32[] [], "Value"=w2273, "Name"=w2279) -> ("output cluster"=w2278:T1)  [unwired: 3 in]
    }
    frame "Counter Input:Pulse Width:Digital Filter:Timebase:Rate" {
      n456 = property class="DAQmx Channel"(reference=w2281, error in=w2287, "ActiveChans"=w2282) -> (reference out=w2290:refnum<k21>, error out=w2286:errorcluster, "CI.PulseWidth.DigFltr.TimebaseRate"=w2283:dbl)
      n457 = call-poly <vilib>:"ex_setTdmProperty.vi"("Strings"=string[] [], "Values"=i32[] [], "Value"=w2283, "Name"=w2289) -> ("output cluster"=w2288:T1)  [unwired: 3 in]
    }
    frame "Counter Input:Pulse Width:Digital Synchronization:Enable" {
      n458 = property class="DAQmx Channel"(reference=w2291, error in=w2297, "ActiveChans"=w2292) -> (reference out=w2300:refnum<k21>, error out=w2296:errorcluster, "CI.PulseWidth.DigSync.Enable"=w2293:bool)
      n459 = call-poly <vilib>:"ex_setTdmProperty.vi"("Strings"=string[] [], "Values"=i32[] [], "Value"=w2293, "Name"=w2299) -> ("output cluster"=w2298:T1)  [unwired: 3 in]
    }
    frame "Counter Input:Two Edge Separation:Units" {
      n460 = property class="DAQmx Channel"(reference=w2301, error in=w2307, "ActiveChans"=w2302) -> (reference out=w2310:refnum<k21>, error out=w2306:errorcluster, "CI.TwoEdgeSep.Units"=w2303:i32)
      n461 = call-poly <vilib>:"ex_setTdmProperty.vi"("Strings"=string[] ["Seconds", "Ticks", "From Custom Scale"], "Values"=i32[] [10364, 10304, 10065], "Value"=w2303, "Name"=w2309) -> ("output cluster"=w2308:T1)  [unwired: 3 in]
    }
    frame "Counter Input:Two Edge Separation:First:Input Terminal" {
      n462 = property class="DAQmx Channel"(reference=w2311, error in=w2317, "ActiveChans"=w2312) -> (reference out=w2320:refnum<k21>, error out=w2316:errorcluster, "CI.TwoEdgeSep.First.Term"=w2313:tag)
      n463 = call-poly <vilib>:"ex_setTdmProperty.vi"("Strings"=string[] [], "Values"=i32[] [], "Value"=w2313, "Name"=w2319) -> ("output cluster"=w2318:T1)  [unwired: 3 in]
    }
    frame "Counter Input:Two Edge Separation:First:Edge" {
      n464 = property class="DAQmx Channel"(reference=w2321, error in=w2327, "ActiveChans"=w2322) -> (reference out=w2330:refnum<k21>, error out=w2326:errorcluster, "CI.TwoEdgeSep.First.Edge"=w2323:i32)
      n465 = call-poly <vilib>:"ex_setTdmProperty.vi"("Strings"=string[] ["Rising", "Falling"], "Values"=i32[] [10280, 10171], "Value"=w2323, "Name"=w2329) -> ("output cluster"=w2328:T1)  [unwired: 3 in]
    }
    frame "Counter Input:Two Edge Separation:First:Digital Filter:Enable" {
      n466 = property class="DAQmx Channel"(reference=w2331, error in=w2337, "ActiveChans"=w2332) -> (reference out=w2340:refnum<k21>, error out=w2336:errorcluster, "CI.TwoEdgeSep.First.DigFltr.Enable"=w2333:bool)
      n467 = call-poly <vilib>:"ex_setTdmProperty.vi"("Strings"=string[] [], "Values"=i32[] [], "Value"=w2333, "Name"=w2339) -> ("output cluster"=w2338:T1)  [unwired: 3 in]
    }
    frame "Counter Input:Two Edge Separation:First:Digital Filter:Minimum Pulse Width" {
      n468 = property class="DAQmx Channel"(reference=w2341, error in=w2347, "ActiveChans"=w2342) -> (reference out=w2350:refnum<k21>, error out=w2346:errorcluster, "CI.TwoEdgeSep.First.DigFltr.MinPulseWidth"=w2343:dbl)
      n469 = call-poly <vilib>:"ex_setTdmProperty.vi"("Strings"=string[] [], "Values"=i32[] [], "Value"=w2343, "Name"=w2349) -> ("output cluster"=w2348:T1)  [unwired: 3 in]
    }
    frame "Counter Input:Two Edge Separation:First:Digital Filter:Timebase:Source" {
      n470 = property class="DAQmx Channel"(reference=w2351, error in=w2357, "ActiveChans"=w2352) -> (reference out=w2360:refnum<k21>, error out=w2356:errorcluster, "CI.TwoEdgeSep.First.DigFltr.TimebaseSrc"=w2353:tag)
      n471 = call-poly <vilib>:"ex_setTdmProperty.vi"("Strings"=string[] [], "Values"=i32[] [], "Value"=w2353, "Name"=w2359) -> ("output cluster"=w2358:T1)  [unwired: 3 in]
    }
    frame "Counter Input:Two Edge Separation:First:Digital Filter:Timebase:Rate" {
      n472 = property class="DAQmx Channel"(reference=w2361, error in=w2367, "ActiveChans"=w2362) -> (reference out=w2370:refnum<k21>, error out=w2366:errorcluster, "CI.TwoEdgeSep.First.DigFltr.TimebaseRate"=w2363:dbl)
      n473 = call-poly <vilib>:"ex_setTdmProperty.vi"("Strings"=string[] [], "Values"=i32[] [], "Value"=w2363, "Name"=w2369) -> ("output cluster"=w2368:T1)  [unwired: 3 in]
    }
    frame "Counter Input:Two Edge Separation:First:Digital Synchronization:Enable" {
      n474 = property class="DAQmx Channel"(reference=w2371, error in=w2377, "ActiveChans"=w2372) -> (reference out=w2380:refnum<k21>, error out=w2376:errorcluster, "CI.TwoEdgeSep.First.DigSync.Enable"=w2373:bool)
      n475 = call-poly <vilib>:"ex_setTdmProperty.vi"("Strings"=string[] [], "Values"=i32[] [], "Value"=w2373, "Name"=w2379) -> ("output cluster"=w2378:T1)  [unwired: 3 in]
    }
    frame "Counter Input:Two Edge Separation:Second:Input Terminal" {
      n476 = property class="DAQmx Channel"(reference=w2381, error in=w2387, "ActiveChans"=w2382) -> (reference out=w2390:refnum<k21>, error out=w2386:errorcluster, "CI.TwoEdgeSep.Second.Term"=w2383:tag)
      n477 = call-poly <vilib>:"ex_setTdmProperty.vi"("Strings"=string[] [], "Values"=i32[] [], "Value"=w2383, "Name"=w2389) -> ("output cluster"=w2388:T1)  [unwired: 3 in]
    }
    frame "Counter Input:Two Edge Separation:Second:Edge" {
      n478 = property class="DAQmx Channel"(reference=w2391, error in=w2397, "ActiveChans"=w2392) -> (reference out=w2400:refnum<k21>, error out=w2396:errorcluster, "CI.TwoEdgeSep.Second.Edge"=w2393:i32)
      n479 = call-poly <vilib>:"ex_setTdmProperty.vi"("Strings"=string[] ["Rising", "Falling"], "Values"=i32[] [10280, 10171], "Value"=w2393, "Name"=w2399) -> ("output cluster"=w2398:T1)  [unwired: 3 in]
    }
    frame "Counter Input:Two Edge Separation:Second:Digital Filter:Enable" {
      n480 = property class="DAQmx Channel"(reference=w2401, error in=w2407, "ActiveChans"=w2402) -> (reference out=w2410:refnum<k21>, error out=w2406:errorcluster, "CI.TwoEdgeSep.Second.DigFltr.Enable"=w2403:bool)
      n481 = call-poly <vilib>:"ex_setTdmProperty.vi"("Strings"=string[] [], "Values"=i32[] [], "Value"=w2403, "Name"=w2409) -> ("output cluster"=w2408:T1)  [unwired: 3 in]
    }
    frame "Counter Input:Two Edge Separation:Second:Digital Filter:Minimum Pulse Width" {
      n482 = property class="DAQmx Channel"(reference=w2411, error in=w2417, "ActiveChans"=w2412) -> (reference out=w2420:refnum<k21>, error out=w2416:errorcluster, "CI.TwoEdgeSep.Second.DigFltr.MinPulseWidth"=w2413:dbl)
      n483 = call-poly <vilib>:"ex_setTdmProperty.vi"("Strings"=string[] [], "Values"=i32[] [], "Value"=w2413, "Name"=w2419) -> ("output cluster"=w2418:T1)  [unwired: 3 in]
    }
    frame "Counter Input:Two Edge Separation:Second:Digital Filter:Timebase:Source" {
      n484 = property class="DAQmx Channel"(reference=w2421, error in=w2427, "ActiveChans"=w2422) -> (reference out=w2430:refnum<k21>, error out=w2426:errorcluster, "CI.TwoEdgeSep.Second.DigFltr.TimebaseSrc"=w2423:tag)
      n485 = call-poly <vilib>:"ex_setTdmProperty.vi"("Strings"=string[] [], "Values"=i32[] [], "Value"=w2423, "Name"=w2429) -> ("output cluster"=w2428:T1)  [unwired: 3 in]
    }
    frame "Counter Input:Two Edge Separation:Second:Digital Filter:Timebase:Rate" {
      n486 = property class="DAQmx Channel"(reference=w2431, error in=w2437, "ActiveChans"=w2432) -> (reference out=w2440:refnum<k21>, error out=w2436:errorcluster, "CI.TwoEdgeSep.Second.DigFltr.TimebaseRate"=w2433:dbl)
      n487 = call-poly <vilib>:"ex_setTdmProperty.vi"("Strings"=string[] [], "Values"=i32[] [], "Value"=w2433, "Name"=w2439) -> ("output cluster"=w2438:T1)  [unwired: 3 in]
    }
    frame "Counter Input:Two Edge Separation:Second:Digital Synchronization:Enable" {
      n488 = property class="DAQmx Channel"(reference=w2441, error in=w2447, "ActiveChans"=w2442) -> (reference out=w2450:refnum<k21>, error out=w2446:errorcluster, "CI.TwoEdgeSep.Second.DigSync.Enable"=w2443:bool)
      n489 = call-poly <vilib>:"ex_setTdmProperty.vi"("Strings"=string[] [], "Values"=i32[] [], "Value"=w2443, "Name"=w2449) -> ("output cluster"=w2448:T1)  [unwired: 3 in]
    }
    frame "Counter Input:Semi-Period:Units" {
      n490 = property class="DAQmx Channel"(reference=w2451, error in=w2457, "ActiveChans"=w2452) -> (reference out=w2460:refnum<k21>, error out=w2456:errorcluster, "CI.SemiPeriod.Units"=w2453:i32)
      n491 = call-poly <vilib>:"ex_setTdmProperty.vi"("Strings"=string[] ["Seconds", "Ticks", "From Custom Scale"], "Values"=i32[] [10364, 10304, 10065], "Value"=w2453, "Name"=w2459) -> ("output cluster"=w2458:T1)  [unwired: 3 in]
    }
    frame "Counter Input:Semi-Period:Input Terminal" {
      n492 = property class="DAQmx Channel"(reference=w2461, error in=w2467, "ActiveChans"=w2462) -> (reference out=w2470:refnum<k21>, error out=w2466:errorcluster, "CI.SemiPeriod.Term"=w2463:tag)
      n493 = call-poly <vilib>:"ex_setTdmProperty.vi"("Strings"=string[] [], "Values"=i32[] [], "Value"=w2463, "Name"=w2469) -> ("output cluster"=w2468:T1)  [unwired: 3 in]
    }
    frame "Counter Input:Semi-Period:Starting Edge" {
      n494 = property class="DAQmx Channel"(reference=w2471, error in=w2477, "ActiveChans"=w2472) -> (reference out=w2480:refnum<k21>, error out=w2476:errorcluster, "CI.SemiPeriod.StartingEdge"=w2473:i32)
      n495 = call-poly <vilib>:"ex_setTdmProperty.vi"("Strings"=string[] ["Rising", "Falling"], "Values"=i32[] [10280, 10171], "Value"=w2473, "Name"=w2479) -> ("output cluster"=w2478:T1)  [unwired: 3 in]
    }
    frame "Counter Input:Semi-Period:Digital Filter:Enable" {
      n496 = property class="DAQmx Channel"(reference=w2481, error in=w2487, "ActiveChans"=w2482) -> (reference out=w2490:refnum<k21>, error out=w2486:errorcluster, "CI.SemiPeriod.DigFltr.Enable"=w2483:bool)
      n497 = call-poly <vilib>:"ex_setTdmProperty.vi"("Strings"=string[] [], "Values"=i32[] [], "Value"=w2483, "Name"=w2489) -> ("output cluster"=w2488:T1)  [unwired: 3 in]
    }
    frame "Counter Input:Semi-Period:Digital Filter:Minimum Pulse Width" {
      n498 = property class="DAQmx Channel"(reference=w2491, error in=w2497, "ActiveChans"=w2492) -> (reference out=w2500:refnum<k21>, error out=w2496:errorcluster, "CI.SemiPeriod.DigFltr.MinPulseWidth"=w2493:dbl)
      n499 = call-poly <vilib>:"ex_setTdmProperty.vi"("Strings"=string[] [], "Values"=i32[] [], "Value"=w2493, "Name"=w2499) -> ("output cluster"=w2498:T1)  [unwired: 3 in]
    }
    frame "Counter Input:Semi-Period:Digital Filter:Timebase:Source" {
      n500 = property class="DAQmx Channel"(reference=w2501, error in=w2507, "ActiveChans"=w2502) -> (reference out=w2510:refnum<k21>, error out=w2506:errorcluster, "CI.SemiPeriod.DigFltr.TimebaseSrc"=w2503:tag)
      n501 = call-poly <vilib>:"ex_setTdmProperty.vi"("Strings"=string[] [], "Values"=i32[] [], "Value"=w2503, "Name"=w2509) -> ("output cluster"=w2508:T1)  [unwired: 3 in]
    }
    frame "Counter Input:Semi-Period:Digital Filter:Timebase:Rate" {
      n502 = property class="DAQmx Channel"(reference=w2511, error in=w2517, "ActiveChans"=w2512) -> (reference out=w2520:refnum<k21>, error out=w2516:errorcluster, "CI.SemiPeriod.DigFltr.TimebaseRate"=w2513:dbl)
      n503 = call-poly <vilib>:"ex_setTdmProperty.vi"("Strings"=string[] [], "Values"=i32[] [], "Value"=w2513, "Name"=w2519) -> ("output cluster"=w2518:T1)  [unwired: 3 in]
    }
    frame "Counter Input:Semi-Period:Digital Synchronization:Enable" {
      n504 = property class="DAQmx Channel"(reference=w2521, error in=w2527, "ActiveChans"=w2522) -> (reference out=w2530:refnum<k21>, error out=w2526:errorcluster, "CI.SemiPeriod.DigSync.Enable"=w2523:bool)
      n505 = call-poly <vilib>:"ex_setTdmProperty.vi"("Strings"=string[] [], "Values"=i32[] [], "Value"=w2523, "Name"=w2529) -> ("output cluster"=w2528:T1)  [unwired: 3 in]
    }
    frame "Counter Input:Timestamp:Units" {
      n506 = property class="DAQmx Channel"(reference=w2531, error in=w2537, "ActiveChans"=w2532) -> (reference out=w2540:refnum<k21>, error out=w2536:errorcluster, "CI.Timestamp.Units"=w2533:i32)
      n507 = call-poly <vilib>:"ex_setTdmProperty.vi"("Strings"=string[] ["Seconds", "From Custom Scale"], "Values"=i32[] [10364, 10065], "Value"=w2533, "Name"=w2539) -> ("output cluster"=w2538:T1)  [unwired: 3 in]
    }
    frame "Counter Input:Timestamp:Initial Seconds" {
      n508 = property class="DAQmx Channel"(reference=w2541, error in=w2547, "ActiveChans"=w2542) -> (reference out=w2550:refnum<k21>, error out=w2546:errorcluster, "CI.Timestamp.InitialSeconds"=w2543:u32)
      n509 = call-poly <vilib>:"ex_setTdmProperty.vi"("Strings"=string[] [], "Values"=i32[] [], "Value"=w2543, "Name"=w2549) -> ("output cluster"=w2548:T1)  [unwired: 3 in]
    }
    frame "Counter Input:Timestamp:GPS:Synchronization Method" {
      n510 = property class="DAQmx Channel"(reference=w2551, error in=w2557, "ActiveChans"=w2552) -> (reference out=w2560:refnum<k21>, error out=w2556:errorcluster, "CI.GPS.SyncMethod"=w2553:i32)
      n511 = call-poly <vilib>:"ex_setTdmProperty.vi"("Strings"=string[] ["IRIG-B", "PPS", "None"], "Values"=i32[] [10070, 10080, 10230], "Value"=w2553, "Name"=w2559) -> ("output cluster"=w2558:T1)  [unwired: 3 in]
    }
    frame "Counter Input:Timestamp:GPS:Synchronization Source" {
      n512 = property class="DAQmx Channel"(reference=w2561, error in=w2567, "ActiveChans"=w2562) -> (reference out=w2570:refnum<k21>, error out=w2566:errorcluster, "CI.GPS.SyncSrc"=w2563:tag)
      n513 = call-poly <vilib>:"ex_setTdmProperty.vi"("Strings"=string[] [], "Values"=i32[] [], "Value"=w2563, "Name"=w2569) -> ("output cluster"=w2568:T1)  [unwired: 3 in]
    }
    frame "Counter Input:General Properties:Counter Timebase:Source" {
      n514 = property class="DAQmx Channel"(reference=w2571, error in=w2577, "ActiveChans"=w2572) -> (reference out=w2580:refnum<k21>, error out=w2576:errorcluster, "CI.CtrTimebaseSrc"=w2573:tag)
      n515 = call-poly <vilib>:"ex_setTdmProperty.vi"("Strings"=string[] [], "Values"=i32[] [], "Value"=w2573, "Name"=w2579) -> ("output cluster"=w2578:T1)  [unwired: 3 in]
    }
    frame "Counter Input:General Properties:Counter Timebase:Rate" {
      n516 = property class="DAQmx Channel"(reference=w2581, error in=w2587, "ActiveChans"=w2582) -> (reference out=w2590:refnum<k21>, error out=w2586:errorcluster, "CI.CtrTimebaseRate"=w2583:dbl)
      n517 = call-poly <vilib>:"ex_setTdmProperty.vi"("Strings"=string[] [], "Values"=i32[] [], "Value"=w2583, "Name"=w2589) -> ("output cluster"=w2588:T1)  [unwired: 3 in]
    }
    frame "Counter Input:General Properties:Counter Timebase:Active Edge" {
      n518 = property class="DAQmx Channel"(reference=w2591, error in=w2597, "ActiveChans"=w2592) -> (reference out=w2600:refnum<k21>, error out=w2596:errorcluster, "CI.CtrTimebaseActiveEdge"=w2593:i32)
      n519 = call-poly <vilib>:"ex_setTdmProperty.vi"("Strings"=string[] ["Rising", "Falling"], "Values"=i32[] [10280, 10171], "Value"=w2593, "Name"=w2599) -> ("output cluster"=w2598:T1)  [unwired: 3 in]
    }
    frame "Counter Input:General Properties:Counter Timebase:Digital Filter:Enable" {
      n520 = property class="DAQmx Channel"(reference=w2601, error in=w2607, "ActiveChans"=w2602) -> (reference out=w2610:refnum<k21>, error out=w2606:errorcluster, "CI.CtrTimebase.DigFltr.Enable"=w2603:bool)
      n521 = call-poly <vilib>:"ex_setTdmProperty.vi"("Strings"=string[] [], "Values"=i32[] [], "Value"=w2603, "Name"=w2609) -> ("output cluster"=w2608:T1)  [unwired: 3 in]
    }
    frame "Counter Input:General Properties:Counter Timebase:Digital Filter:Minimum Pulse Width" {
      n522 = property class="DAQmx Channel"(reference=w2611, error in=w2617, "ActiveChans"=w2612) -> (reference out=w2620:refnum<k21>, error out=w2616:errorcluster, "CI.CtrTimebase.DigFltr.MinPulseWidth"=w2613:dbl)
      n523 = call-poly <vilib>:"ex_setTdmProperty.vi"("Strings"=string[] [], "Values"=i32[] [], "Value"=w2613, "Name"=w2619) -> ("output cluster"=w2618:T1)  [unwired: 3 in]
    }
    frame "Counter Input:General Properties:Counter Timebase:Digital Filter:Timebase:Source" {
      n524 = property class="DAQmx Channel"(reference=w2621, error in=w2627, "ActiveChans"=w2622) -> (reference out=w2630:refnum<k21>, error out=w2626:errorcluster, "CI.CtrTimebase.DigFltr.TimebaseSrc"=w2623:tag)
      n525 = call-poly <vilib>:"ex_setTdmProperty.vi"("Strings"=string[] [], "Values"=i32[] [], "Value"=w2623, "Name"=w2629) -> ("output cluster"=w2628:T1)  [unwired: 3 in]
    }
    frame "Counter Input:General Properties:Counter Timebase:Digital Filter:Timebase:Rate" {
      n526 = property class="DAQmx Channel"(reference=w2631, error in=w2637, "ActiveChans"=w2632) -> (reference out=w2640:refnum<k21>, error out=w2636:errorcluster, "CI.CtrTimebase.DigFltr.TimebaseRate"=w2633:dbl)
      n527 = call-poly <vilib>:"ex_setTdmProperty.vi"("Strings"=string[] [], "Values"=i32[] [], "Value"=w2633, "Name"=w2639) -> ("output cluster"=w2638:T1)  [unwired: 3 in]
    }
    frame "Counter Input:General Properties:Counter Timebase:Digital Synchronization:Enable" {
      n528 = property class="DAQmx Channel"(reference=w2641, error in=w2647, "ActiveChans"=w2642) -> (reference out=w2650:refnum<k21>, error out=w2646:errorcluster, "CI.CtrTimebase.DigSync.Enable"=w2643:bool)
      n529 = call-poly <vilib>:"ex_setTdmProperty.vi"("Strings"=string[] [], "Values"=i32[] [], "Value"=w2643, "Name"=w2649) -> ("output cluster"=w2648:T1)  [unwired: 3 in]
    }
    frame "Counter Input:General Properties:More:Count" {
      n530 = property class="DAQmx Channel"(reference=w2651, error in=w2657, "ActiveChans"=w2652) -> (reference out=w2660:refnum<k21>, error out=w2656:errorcluster, "CI.Count"=w2653:u32)
      n531 = call-poly <vilib>:"ex_setTdmProperty.vi"("Strings"=string[] [], "Values"=i32[] [], "Value"=w2653, "Name"=w2659) -> ("output cluster"=w2658:T1)  [unwired: 3 in]
    }
    frame "Counter Input:General Properties:More:Output State" {
      n532 = property class="DAQmx Channel"(reference=w2661, error in=w2667, "ActiveChans"=w2662) -> (reference out=w2670:refnum<k21>, error out=w2666:errorcluster, "CI.OutputState"=w2663:i32)
      n533 = call-poly <vilib>:"ex_setTdmProperty.vi"("Strings"=string[] ["High", "Low"], "Values"=i32[] [10192, 10214], "Value"=w2663, "Name"=w2669) -> ("output cluster"=w2668:T1)  [unwired: 3 in]
    }
    frame "Counter Input:General Properties:More:Terminal Count Reached" {
      n534 = property class="DAQmx Channel"(reference=w2671, error in=w2677, "ActiveChans"=w2672) -> (reference out=w2680:refnum<k21>, error out=w2676:errorcluster, "CI.TCReached"=w2673:bool)
      n535 = call-poly <vilib>:"ex_setTdmProperty.vi"("Strings"=string[] [], "Values"=i32[] [], "Value"=w2673, "Name"=w2679) -> ("output cluster"=w2678:T1)  [unwired: 3 in]
    }
    frame "Counter Input:General Properties:More:Counter Timebase Master Timebase Divisor" {
      n536 = property class="DAQmx Channel"(reference=w2681, error in=w2687, "ActiveChans"=w2682) -> (reference out=w2690:refnum<k21>, error out=w2686:errorcluster, "CI.CtrTimebaseMasterTimebaseDiv"=w2683:u32)
      n537 = call-poly <vilib>:"ex_setTdmProperty.vi"("Strings"=string[] ["1", "200"], "Values"=i32[] [1, 200], "Value"=w2683, "Name"=w2689) -> ("output cluster"=w2688:T1)  [unwired: 3 in]
    }
    frame "Counter Input:General Properties:More:Advanced:Data Transfer and Memory:Data Transfer Mechanism" {
      n538 = property class="DAQmx Channel"(reference=w2691, error in=w2697, "ActiveChans"=w2692) -> (reference out=w2700:refnum<k21>, error out=w2696:errorcluster, "CI.DataXferMech"=w2693:i32)
      n539 = call-poly <vilib>:"ex_setTdmProperty.vi"("Strings"=string[] ["DMA", "Interrupts", "Programmed I/O"], "Values"=i32[] [10054, 10204, 10264], "Value"=w2693, "Name"=w2699) -> ("output cluster"=w2698:T1)  [unwired: 3 in]
    }
    frame "Counter Input:General Properties:More:Advanced:Data Transfer and Memory:Number Of Possibly Invalid Samples" {
      n540 = property class="DAQmx Channel"(reference=w2701, error in=w2707, "ActiveChans"=w2702) -> (reference out=w2710:refnum<k21>, error out=w2706:errorcluster, "CI.NumPossiblyInvalidSamps"=w2703:u32)
      n541 = call-poly <vilib>:"ex_setTdmProperty.vi"("Strings"=string[] [], "Values"=i32[] [], "Value"=w2703, "Name"=w2709) -> ("output cluster"=w2708:T1)  [unwired: 3 in]
    }
    frame "Counter Input:General Properties:More:Advanced:Duplicate Count Prevention" {
      n542 = property class="DAQmx Channel"(reference=w2711, error in=w2717, "ActiveChans"=w2712) -> (reference out=w2720:refnum<k21>, error out=w2716:errorcluster, "CI.DupCountPrevention"=w2713:bool)
      n543 = call-poly <vilib>:"ex_setTdmProperty.vi"("Strings"=string[] [], "Values"=i32[] [], "Value"=w2713, "Name"=w2719) -> ("output cluster"=w2718:T1)  [unwired: 3 in]
    }
    frame "Counter Input:General Properties:More:Advanced:Prescaler" {
      n544 = property class="DAQmx Channel"(reference=w2721, error in=w2727, "ActiveChans"=w2722) -> (reference out=w2730:refnum<k21>, error out=w2726:errorcluster, "CI.Prescaler"=w2723:u32)
      n545 = call-poly <vilib>:"ex_setTdmProperty.vi"("Strings"=string[] ["1", "2", "8"], "Values"=i32[] [1, 2, 8], "Value"=w2723, "Name"=w2729) -> ("output cluster"=w2728:T1)  [unwired: 3 in]
    }
    frame "Counter Output:Output Type" {
      n546 = property class="DAQmx Channel"(reference=w2731, error in=w2737, "ActiveChans"=w2732) -> (reference out=w2740:refnum<k21>, error out=w2736:errorcluster, "CO.OutputType"=w2733:i32)
      n547 = call-poly <vilib>:"ex_setTdmProperty.vi"("Strings"=string[] ["Pulse:Time", "Pulse:Frequency", "Pulse:Ticks"], "Values"=i32[] [10269, 10119, 10268], "Value"=w2733, "Name"=w2739) -> ("output cluster"=w2738:T1)  [unwired: 3 in]
    }
    frame "Counter Output:Pulse:Idle State" {
      n548 = property class="DAQmx Channel"(reference=w2741, error in=w2747, "ActiveChans"=w2742) -> (reference out=w2750:refnum<k21>, error out=w2746:errorcluster, "CO.Pulse.IdleState"=w2743:i32)
      n549 = call-poly <vilib>:"ex_setTdmProperty.vi"("Strings"=string[] ["High", "Low"], "Values"=i32[] [10192, 10214], "Value"=w2743, "Name"=w2749) -> ("output cluster"=w2748:T1)  [unwired: 3 in]
    }
    frame "Counter Output:Pulse:Output Terminal" {
      n550 = property class="DAQmx Channel"(reference=w2751, error in=w2757, "ActiveChans"=w2752) -> (reference out=w2760:refnum<k21>, error out=w2756:errorcluster, "CO.Pulse.Term"=w2753:tag)
      n551 = call-poly <vilib>:"ex_setTdmProperty.vi"("Strings"=string[] [], "Values"=i32[] [], "Value"=w2753, "Name"=w2759) -> ("output cluster"=w2758:T1)  [unwired: 3 in]
    }
    frame "Counter Output:Pulse:Time:Units" {
      n552 = property class="DAQmx Channel"(reference=w2761, error in=w2767, "ActiveChans"=w2762) -> (reference out=w2770:refnum<k21>, error out=w2766:errorcluster, "CO.Pulse.Time.Units"=w2763:i32)
      n553 = call-poly <vilib>:"ex_setTdmProperty.vi"("Strings"=string[] ["Seconds"], "Values"=i32[] [10364], "Value"=w2763, "Name"=w2769) -> ("output cluster"=w2768:T1)  [unwired: 3 in]
    }
    frame "Counter Output:Pulse:Time:High Time" {
      n554 = property class="DAQmx Channel"(reference=w2771, error in=w2777, "ActiveChans"=w2772) -> (reference out=w2780:refnum<k21>, error out=w2776:errorcluster, "CO.Pulse.HighTime"=w2773:dbl)
      n555 = call-poly <vilib>:"ex_setTdmProperty.vi"("Strings"=string[] [], "Values"=i32[] [], "Value"=w2773, "Name"=w2779) -> ("output cluster"=w2778:T1)  [unwired: 3 in]
    }
    frame "Counter Output:Pulse:Time:Low Time" {
      n556 = property class="DAQmx Channel"(reference=w2781, error in=w2787, "ActiveChans"=w2782) -> (reference out=w2790:refnum<k21>, error out=w2786:errorcluster, "CO.Pulse.LowTime"=w2783:dbl)
      n557 = call-poly <vilib>:"ex_setTdmProperty.vi"("Strings"=string[] [], "Values"=i32[] [], "Value"=w2783, "Name"=w2789) -> ("output cluster"=w2788:T1)  [unwired: 3 in]
    }
    frame "Counter Output:Pulse:Time:Initial Delay" {
      n558 = property class="DAQmx Channel"(reference=w2791, error in=w2797, "ActiveChans"=w2792) -> (reference out=w2800:refnum<k21>, error out=w2796:errorcluster, "CO.Pulse.Time.InitialDelay"=w2793:dbl)
      n559 = call-poly <vilib>:"ex_setTdmProperty.vi"("Strings"=string[] [], "Values"=i32[] [], "Value"=w2793, "Name"=w2799) -> ("output cluster"=w2798:T1)  [unwired: 3 in]
    }
    frame "Counter Output:Pulse:Frequency:Duty Cycle" {
      n560 = property class="DAQmx Channel"(reference=w2801, error in=w2807, "ActiveChans"=w2802) -> (reference out=w2810:refnum<k21>, error out=w2806:errorcluster, "CO.Pulse.DutyCyc"=w2803:dbl)
      n561 = call-poly <vilib>:"ex_setTdmProperty.vi"("Strings"=string[] [], "Values"=i32[] [], "Value"=w2803, "Name"=w2809) -> ("output cluster"=w2808:T1)  [unwired: 3 in]
    }
    frame "Counter Output:Pulse:Frequency:Units" {
      n562 = property class="DAQmx Channel"(reference=w2811, error in=w2817, "ActiveChans"=w2812) -> (reference out=w2820:refnum<k21>, error out=w2816:errorcluster, "CO.Pulse.Freq.Units"=w2813:i32)
      n563 = call-poly <vilib>:"ex_setTdmProperty.vi"("Strings"=string[] ["Hz"], "Values"=i32[] [10373], "Value"=w2813, "Name"=w2819) -> ("output cluster"=w2818:T1)  [unwired: 3 in]
    }
    frame "Counter Output:Pulse:Frequency:Frequency" {
      n564 = property class="DAQmx Channel"(reference=w2821, error in=w2827, "ActiveChans"=w2822) -> (reference out=w2830:refnum<k21>, error out=w2826:errorcluster, "CO.Pulse.Freq"=w2823:dbl)
      n565 = call-poly <vilib>:"ex_setTdmProperty.vi"("Strings"=string[] [], "Values"=i32[] [], "Value"=w2823, "Name"=w2829) -> ("output cluster"=w2828:T1)  [unwired: 3 in]
    }
    frame "Counter Output:Pulse:Frequency:Initial Delay" {
      n566 = property class="DAQmx Channel"(reference=w2831, error in=w2837, "ActiveChans"=w2832) -> (reference out=w2840:refnum<k21>, error out=w2836:errorcluster, "CO.Pulse.Freq.InitialDelay"=w2833:dbl)
      n567 = call-poly <vilib>:"ex_setTdmProperty.vi"("Strings"=string[] [], "Values"=i32[] [], "Value"=w2833, "Name"=w2839) -> ("output cluster"=w2838:T1)  [unwired: 3 in]
    }
    frame "Counter Output:Pulse:Ticks:High Ticks" {
      n568 = property class="DAQmx Channel"(reference=w2841, error in=w2847, "ActiveChans"=w2842) -> (reference out=w2850:refnum<k21>, error out=w2846:errorcluster, "CO.Pulse.HighTicks"=w2843:u32)
      n569 = call-poly <vilib>:"ex_setTdmProperty.vi"("Strings"=string[] [], "Values"=i32[] [], "Value"=w2843, "Name"=w2849) -> ("output cluster"=w2848:T1)  [unwired: 3 in]
    }
    frame "Counter Output:Pulse:Ticks:Low Ticks" {
      n570 = property class="DAQmx Channel"(reference=w2851, error in=w2857, "ActiveChans"=w2852) -> (reference out=w2860:refnum<k21>, error out=w2856:errorcluster, "CO.Pulse.LowTicks"=w2853:u32)
      n571 = call-poly <vilib>:"ex_setTdmProperty.vi"("Strings"=string[] [], "Values"=i32[] [], "Value"=w2853, "Name"=w2859) -> ("output cluster"=w2858:T1)  [unwired: 3 in]
    }
    frame "Counter Output:Pulse:Ticks:Initial Delay" {
      n572 = property class="DAQmx Channel"(reference=w2861, error in=w2867, "ActiveChans"=w2862) -> (reference out=w2870:refnum<k21>, error out=w2866:errorcluster, "CO.Pulse.Ticks.InitialDelay"=w2863:u32)
      n573 = call-poly <vilib>:"ex_setTdmProperty.vi"("Strings"=string[] [], "Values"=i32[] [], "Value"=w2863, "Name"=w2869) -> ("output cluster"=w2868:T1)  [unwired: 3 in]
    }
    frame "Counter Output:General Properties:Counter Timebase:Source" {
      n574 = property class="DAQmx Channel"(reference=w2871, error in=w2877, "ActiveChans"=w2872) -> (reference out=w2880:refnum<k21>, error out=w2876:errorcluster, "CO.CtrTimebaseSrc"=w2873:tag)
      n575 = call-poly <vilib>:"ex_setTdmProperty.vi"("Strings"=string[] [], "Values"=i32[] [], "Value"=w2873, "Name"=w2879) -> ("output cluster"=w2878:T1)  [unwired: 3 in]
    }
    frame "Counter Output:General Properties:Counter Timebase:Rate" {
      n576 = property class="DAQmx Channel"(reference=w2881, error in=w2887, "ActiveChans"=w2882) -> (reference out=w2890:refnum<k21>, error out=w2886:errorcluster, "CO.CtrTimebaseRate"=w2883:dbl)
      n577 = call-poly <vilib>:"ex_setTdmProperty.vi"("Strings"=string[] [], "Values"=i32[] [], "Value"=w2883, "Name"=w2889) -> ("output cluster"=w2888:T1)  [unwired: 3 in]
    }
    frame "Counter Output:General Properties:Counter Timebase:Active Edge" {
      n578 = property class="DAQmx Channel"(reference=w2891, error in=w2897, "ActiveChans"=w2892) -> (reference out=w2900:refnum<k21>, error out=w2896:errorcluster, "CO.CtrTimebaseActiveEdge"=w2893:i32)
      n579 = call-poly <vilib>:"ex_setTdmProperty.vi"("Strings"=string[] ["Rising", "Falling"], "Values"=i32[] [10280, 10171], "Value"=w2893, "Name"=w2899) -> ("output cluster"=w2898:T1)  [unwired: 3 in]
    }
    frame "Counter Output:General Properties:Counter Timebase:Digital Filter:Enable" {
      n580 = property class="DAQmx Channel"(reference=w2901, error in=w2907, "ActiveChans"=w2902) -> (reference out=w2910:refnum<k21>, error out=w2906:errorcluster, "CO.CtrTimebase.DigFltr.Enable"=w2903:bool)
      n581 = call-poly <vilib>:"ex_setTdmProperty.vi"("Strings"=string[] [], "Values"=i32[] [], "Value"=w2903, "Name"=w2909) -> ("output cluster"=w2908:T1)  [unwired: 3 in]
    }
    frame "Counter Output:General Properties:Counter Timebase:Digital Filter:Minimum Pulse Width" {
      n582 = property class="DAQmx Channel"(reference=w2911, error in=w2917, "ActiveChans"=w2912) -> (reference out=w2920:refnum<k21>, error out=w2916:errorcluster, "CO.CtrTimebase.DigFltr.MinPulseWidth"=w2913:dbl)
      n583 = call-poly <vilib>:"ex_setTdmProperty.vi"("Strings"=string[] [], "Values"=i32[] [], "Value"=w2913, "Name"=w2919) -> ("output cluster"=w2918:T1)  [unwired: 3 in]
    }
    frame "Counter Output:General Properties:Counter Timebase:Digital Filter:Timebase:Source" {
      n584 = property class="DAQmx Channel"(reference=w2921, error in=w2927, "ActiveChans"=w2922) -> (reference out=w2930:refnum<k21>, error out=w2926:errorcluster, "CO.CtrTimebase.DigFltr.TimebaseSrc"=w2923:tag)
      n585 = call-poly <vilib>:"ex_setTdmProperty.vi"("Strings"=string[] [], "Values"=i32[] [], "Value"=w2923, "Name"=w2929) -> ("output cluster"=w2928:T1)  [unwired: 3 in]
    }
    frame "Counter Output:General Properties:Counter Timebase:Digital Filter:Timebase:Rate" {
      n586 = property class="DAQmx Channel"(reference=w2931, error in=w2937, "ActiveChans"=w2932) -> (reference out=w2940:refnum<k21>, error out=w2936:errorcluster, "CO.CtrTimebase.DigFltr.TimebaseRate"=w2933:dbl)
      n587 = call-poly <vilib>:"ex_setTdmProperty.vi"("Strings"=string[] [], "Values"=i32[] [], "Value"=w2933, "Name"=w2939) -> ("output cluster"=w2938:T1)  [unwired: 3 in]
    }
    frame "Counter Output:General Properties:Counter Timebase:Digital Synchronization:Enable" {
      n588 = property class="DAQmx Channel"(reference=w2941, error in=w2947, "ActiveChans"=w2942) -> (reference out=w2950:refnum<k21>, error out=w2946:errorcluster, "CO.CtrTimebase.DigSync.Enable"=w2943:bool)
      n589 = call-poly <vilib>:"ex_setTdmProperty.vi"("Strings"=string[] [], "Values"=i32[] [], "Value"=w2943, "Name"=w2949) -> ("output cluster"=w2948:T1)  [unwired: 3 in]
    }
    frame "Counter Output:General Properties:More:Count" {
      n590 = property class="DAQmx Channel"(reference=w2951, error in=w2957, "ActiveChans"=w2952) -> (reference out=w2960:refnum<k21>, error out=w2956:errorcluster, "CO.Count"=w2953:u32)
      n591 = call-poly <vilib>:"ex_setTdmProperty.vi"("Strings"=string[] [], "Values"=i32[] [], "Value"=w2953, "Name"=w2959) -> ("output cluster"=w2958:T1)  [unwired: 3 in]
    }
    frame "Counter Output:General Properties:More:Output State" {
      n592 = property class="DAQmx Channel"(reference=w2961, error in=w2967, "ActiveChans"=w2962) -> (reference out=w2970:refnum<k21>, error out=w2966:errorcluster, "CO.OutputState"=w2963:i32)
      n593 = call-poly <vilib>:"ex_setTdmProperty.vi"("Strings"=string[] ["High", "Low"], "Values"=i32[] [10192, 10214], "Value"=w2963, "Name"=w2969) -> ("output cluster"=w2968:T1)  [unwired: 3 in]
    }
    frame "Counter Output:General Properties:More:Auto Increment Count" {
      n594 = property class="DAQmx Channel"(reference=w2971, error in=w2977, "ActiveChans"=w2972) -> (reference out=w2980:refnum<k21>, error out=w2976:errorcluster, "CO.AutoIncrCnt"=w2973:u32)
      n595 = call-poly <vilib>:"ex_setTdmProperty.vi"("Strings"=string[] [], "Values"=i32[] [], "Value"=w2973, "Name"=w2979) -> ("output cluster"=w2978:T1)  [unwired: 3 in]
    }
    frame "Counter Output:General Properties:More:Counter Timebase Master Timebase Divisor" {
      n596 = property class="DAQmx Channel"(reference=w2981, error in=w2987, "ActiveChans"=w2982) -> (reference out=w2990:refnum<k21>, error out=w2986:errorcluster, "CO.CtrTimebaseMasterTimebaseDiv"=w2983:u32)
      n597 = call-poly <vilib>:"ex_setTdmProperty.vi"("Strings"=string[] ["1", "200"], "Values"=i32[] [1, 200], "Value"=w2983, "Name"=w2989) -> ("output cluster"=w2988:T1)  [unwired: 3 in]
    }
    frame "Counter Output:General Properties:More:Pulse Done" {
      n598 = property class="DAQmx Channel"(reference=w2991, error in=w2997, "ActiveChans"=w2992) -> (reference out=w3000:refnum<k21>, error out=w2996:errorcluster, "CO.PulseDone"=w2993:bool)
      n599 = call-poly <vilib>:"ex_setTdmProperty.vi"("Strings"=string[] [], "Values"=i32[] [], "Value"=w2993, "Name"=w2999) -> ("output cluster"=w2998:T1)  [unwired: 3 in]
    }
    frame "Counter Output:General Properties:More:Advanced:Prescaler" {
      n600 = property class="DAQmx Channel"(reference=w3001, error in=w3007, "ActiveChans"=w3002) -> (reference out=w3010:refnum<k21>, error out=w3006:errorcluster, "CO.Prescaler"=w3003:u32)
      n601 = call-poly <vilib>:"ex_setTdmProperty.vi"("Strings"=string[] ["1", "2", "8"], "Values"=i32[] [1, 2, 8], "Value"=w3003, "Name"=w3009) -> ("output cluster"=w3008:T1)  [unwired: 3 in]
    }
    frame "Counter Output:General Properties:More:Advanced:Ready For New Value" {
      n602 = property class="DAQmx Channel"(reference=w3011, error in=w3017, "ActiveChans"=w3012) -> (reference out=w3020:refnum<k21>, error out=w3016:errorcluster, "CO.RdyForNewVal"=w3013:bool)
      n603 = call-poly <vilib>:"ex_setTdmProperty.vi"("Strings"=string[] [], "Values"=i32[] [], "Value"=w3013, "Name"=w3019) -> ("output cluster"=w3018:T1)  [unwired: 3 in]
    }
    frame "General Properties:Channel Type" {
      n604 = property class="DAQmx Channel"(reference=w3021, error in=w3027, "ActiveChans"=w3022) -> (reference out=w3030:refnum<k21>, error out=w3026:errorcluster, "ChanType"=w3023:i32)
      n605 = call-poly <vilib>:"ex_setTdmProperty.vi"("Strings"=string[] ["Analog Input", "Analog Output", "Digital Input", "Digital Output", "Counter Input", "Counter Output"], "Values"=i32[] [10100, 10102, 10151, 10153, 10131, 10132], "Value"=w3023, "Name"=w3029) -> ("output cluster"=w3028:T1)  [unwired: 3 in]
    }
    frame "General Properties:Physical Channel Name" {
      n606 = property class="DAQmx Channel"(reference=w3031, error in=w3037, "ActiveChans"=w3032) -> (reference out=w3040:refnum<k21>, error out=w3036:errorcluster, "PhysicalChanName"=w3033:tag)
      n607 = call-poly <vilib>:"ex_setTdmProperty.vi"("Strings"=string[] [], "Values"=i32[] [], "Value"=w3033, "Name"=w3039) -> ("output cluster"=w3038:T1)  [unwired: 3 in]
    }
    frame "General Properties:Description" {
      n608 = property class="DAQmx Channel"(reference=w3041, error in=w3047, "ActiveChans"=w3042) -> (reference out=w3050:refnum<k21>, error out=w3046:errorcluster, "Descr"=w3043:string)
      n609 = call-poly <vilib>:"ex_setTdmProperty.vi"("Strings"=string[] [], "Values"=i32[] [], "Value"=w3043, "Name"=w3049) -> ("output cluster"=w3048:T1)  [unwired: 3 in]
    }
    frame "General Properties:Is Global" {
      n610 = property class="DAQmx Channel"(reference=w3051, error in=w3057, "ActiveChans"=w3052) -> (reference out=w3060:refnum<k21>, error out=w3056:errorcluster, "IsGlobal"=w3053:bool)
      n611 = call-poly <vilib>:"ex_setTdmProperty.vi"("Strings"=string[] [], "Values"=i32[] [], "Value"=w3053, "Name"=w3059) -> ("output cluster"=w3058:T1)  [unwired: 3 in]
    }
  }
  "TDM Property" <- w7
  "dup DAQmx Channel" <- w6
  "error out" <- w4
